vi "ControlProgram5.0.vi"() -> ()   [LabVIEW 2016]
uses:
  <vilib>/Utility/error.llb/DialogType.ctl
  <vilib>/Utility/miscctls.llb/LVPoint32TypeDef.ctl
  <vilib>/DAQmx/write.llb/DAQmx Write (Digital Bool 1Line 1Point).vi
  <vilib>/DAQmx/create/channels.llb/DAQmx Create Channel (DO-Digital Output).vi
  <vilib>/platform/TimedLoop/XDataNode/XDataNode.xnode
  <vilib>/Platform/TimedLoop/XDataNode/nitl_modes.ctl
  <vilib>/Platform/TimedLoop/XDataNode/XDNodeRunTimeDep.lvlib
  <vilib>/Platform/TimedLoop/XDataNode/wakeup.ctl
  <vilib>/Platform/TimedLoop/XDataNode/timing_clust.ctl
  <vilib>/DAQmx/create/channels.llb/DAQmx Create Channel (AI-Voltage-Basic).vi
  <vilib>/DAQmx/create/channels.llb/DAQmx Create Channel (AO-Voltage-Basic).vi
  <vilib>/DAQmx/write.llb/DAQmx Write (Analog 1D DBL NChan 1Samp).vi
  <resource>/objmgr/daqmx.rc
  <vilib>/Analysis/NI_AALBase.lvlib
  <vilib>/Analysis/baseanly.llb/Mean (DBL).vi
  <vilib>/Instr/_visa.llb/VISA Configure Serial Port (Instr).vi
  <vilib>/Utility/inputDevices.llb/mouseAcquire.vi
  <vilib>/Utility/inputDevices.llb/closeMouse.vi
  <vilib>/DAQmx/read.llb/DAQmx Read (Analog 2D DBL NChan NSamp).vi
  <vilib>/DAQmx/configure/timing.llb/DAQmx Timing (Sample Clock).vi
panel:
  out "Chart Freq (Hz)":dbl
  out "Waveform Chart 3":dbl[][](graph)
  out "Cal values":T1={"AX alpha"=672.9952101249002, "BX alpha"=822.8320399167465, "AX kappa"=0.3432739170419873, "BX kappa"=0.22087046979741862, "AX offset"=-0.002065833400375715, "BX offset"=0.010483360643544744, "AY alpha"=702.0654168010462, "BY alpha"=773.6701766674906, "AY kappa"=0.33643150106915, "BY kappa"=0.2444549177225145, "AY offset"=-0.1177594339643395, "BY offset"=0.06470506082263472}
  in  "Inject Pump 1":bool
  in  "Inject Pump 2":bool
  in  "Tab Control 2":T2(tab)
  in  "Force FB script":bool
  in  "Got ADig bead":bool
  in  "Move Cap. 2 (ADig Top)":bool
  in  "Dump beads":bool
  in  "Got DNA bead":bool
  in  "Delta after tether":dbl=3.1
  in  "TA Cancel Save?":bool
  in  "Min fish\ndelta (V)":dbl=2.8 min=0.0 max=10.0 step=0.1
  in  "Max fish\ndelta (V)":dbl=3.8 min=0.0 max=10.0 step=0.1
  in  "Fish Speed (ms)":i32=3000
  in  "Wait (ms)":i32=1500
  in  "# attempts":dbl=10.0
  in  "Cutoff force (pN)":dbl=5.0
  in  "Raster after\n tether?":bool=TRUE
  out "Tether":bool
  out "Attempt #":i32
  in  "Cal @ Delta (V)":dbl=5.0
  in  "Cal stage position":i32=3
  in  "Conv Y (nm/V)":dbl=505.0
  in  "Conv X (nm/V)":dbl=892.0
  out "Cal Final Sampling Rate":dbl
  in  "Cal Averaging":i32=1
  in  "Wait before dip (s)":dbl=3.0
  in  "Start dipping after?":bool
  in  "Start trap delta (V)":dbl=3.85
  in  "Cancel dwell":bool
  in  "Pause dwell":bool
  in  "Return position":dbl=3.0
  in  "Dip duration":dbl=15.0
  in  "Dip position":dbl=4.0
  in  "Dip":bool
  out "Dip time":i32
  out "error out":errorcluster
  in  "Stop":bool=TRUE
  in  "?":T3(tab)=enum."Mouse control"
  in  "Save N sets":bool
  in  "N sets":i32=200
  in  "Cal sets to save":i32=25
  in  "Reset data stream":bool
  out "Buffer Overflow":bool
  out "Stage moving":bool
  in  "Comment":string="wtUvrD 0.5 uM ATP"
  in  "Raster scan":bool
  out "Saving":bool
  in  "Save cal":bool
  in  "Save Data":bool
  in  "Stop saving":bool
  out "Calibrating":bool
  out "Progress":dbl(slide) scale=0.0..100.0
  in  "Read Cal":bool
  in  "Fish":bool
  in  "Averaging Number":i32=1250
  out "Final Sampling Rate":dbl=100.0
  in  "Trap position":cluster{"X":dbl, "Y":dbl}={"X"=1.6, "Y"=4.95}
  in  "Trap delta":dbl=5.1 min=0.0 max=10.0 step=0.1
  in  "Fixed X":dbl=1.6
  in  "Fixed Y":dbl=0.7
  in  "Shutter 1 (B)":bool
  in  "Shutter 2 (A)":bool
  in  "Pulling direction":bool=TRUE
  out "Raster scanning...":bool
  out "Current file name":path
  in  "AX alpha":dbl format="%#_3p"
  in  "BX alpha":dbl format="%#_3g"
  in  "AX kappa":dbl format="%#_3g"
  in  "BX kappa":dbl format="%#_3g"
  in  "AX offset":dbl format="%#_3g"
  in  "BX offset":dbl format="%#_3g"
  in  "AY alpha":dbl format="%#_3g"
  in  "BY alpha":dbl format="%#_3g"
  in  "AY kappa":dbl format="%#_3g"
  in  "BY kappa":dbl format="%#_3g"
  in  "AY offset":dbl format="%#_3g"
  in  "BY offset":dbl format="%#_3g"
  out "Buffer status":u8(slide) scale=0.0..100.0
  in  "dump spot":string="Dump beads spot"
  in  "up flow spot":string="Upper flow spot"
  in  "low flow spot":string="Lower flow spot"
  in  "up cap":string="Upper capillary (ADig beads)"
  in  "bottom cap":string="Lower capillary (DNA beads)"
  in  "Move to Position 5":bool
  in  "Set Position 5":bool
  in  "Saved stage positions":dbl[][](array[numeric])=[[1.0, 0.0, 0.0, 0.0], [2.0, 0.28481, -2.63158, -0.02256], [3.0, 1.27978, -0.73974, 0.0], [4.0, 1.27978, -2.1978, 0.0], [5.0, 0.03306, -2.63158, -0.02256]]
  in  "Set Position 2":bool
  in  "Move to Position 2":bool
  in  "Set Position 1":bool
  in  "Move to Position 1":bool
  in  "Set Position 4":bool
  in  "Move to Position 4":bool
  in  "Set Position 3":bool
  in  "Move to Position 3":bool
  out "Stage error":errorcluster
  in  "Normal \nVolume (ul) 2":dbl
  in  "Normal \nRate (ul/hr)":dbl
  in  "Normal \nVolume (ul)":dbl
  in  "Flush\nRate (ul/min)":dbl
  in  "Flush\nVolume (ul)":dbl
  in  "Flush \nRate (ul/min)  2":dbl
  in  "Flush Pump 2":bool
  in  "Flush\nVolume (ul)  2":dbl
  in  "Flush Pump 1":bool
  in  "Normal \nRate (ul/hr)  2":dbl
  in  "Write Wait":i32=1000
  in  "Use Mouse to Move Trap?":bool
  in  "Pause Mouse/Mirror Connection":bool
  out "Reference Voltage":cluster{dbl, dbl}={0.0, -0.0}
  out "Saved voltage":cluster{dbl, dbl}
  out "Real Coordinates":cluster{"Horizontal":i32, "Vertical":i32}={"Horizontal"=145, "Vertical"=-1746}
  out "CoordinatesMousePressed":T4
  out "Sum error":dbl(knob) scale=-0.2..0.2
  out "Trap sep":waveform(dbl)[](graph)
  in  "Set reading to\nsetpoint":bool
  in  "Offset Y (nm)":dbl format="%0.2f"
  in  "Offset X (nm)":dbl format="%0.2f"
  in  "Remove offsets":bool
  in  "Force Feedback":bool
  out "Feedback Output Voltage 2":cluster{dbl, dbl} {"?" format="%#_4g"; "?" format="%#_4g"}
  in  "Max value X":dbl=10.0 format="%.1f"
  in  "Min value X":dbl format="%0.1f"
  in  "Max value Y":dbl=10.0 format="%.1f"
  in  "Min value Y":dbl format="%.1g"
  in  "Offset":cluster{"Off Y":dbl, "Off X":dbl}={"Off Y"=1.5, "Off X"=0.17}
  in  "Setpoint voltage":cluster{"SP Y":dbl, "SP X":dbl}={"SP Y"=0.6, "SP X"=0.0}
  in  "Feedback const":T5={"Ki_B_Y"=0.5, "Ki_B_X"=0.0, "Kp Y"=1.0, "Kp X"=0.0}
  out "Mean Trap Pos X 2 (nm)":dbl format="%0.2f"
  out "Mean Trp Pos Y 2 (nm)":dbl format="%0.2f"
  out "T2 X RMS (A)":dbl format="%0.2f"
  out "T2 Y RMS (A)":dbl format="%0.2f"
  in  "# scans":i32=1
  in  "Speed (ms)":i32=10000
  in  "Min delta":dbl=3.2
  in  "Load param":bool
  in  "Max delta":dbl=4.1
  in  "Scan Parameters":T6(array[cluster])=[{"Label"="Offset", "Max delta 2"=3.8, "Min delta 2"=2.4, "Speed (ms) 2"=10000, "# scans 2"=1}]
  in  "Trap delta\nafter":dbl=3.6
  in  "Stop raster":bool
  out "Scan Range (nm)":dbl
  out "Scan Speed (nm/s)":dbl
  out "Continue to display?":bool
  out "Video Error":errorcluster
  in  "# Samples/channel (in)":i32=40000 format="%.2f"
  out "Buffer size\n(Samples/channel)":u32
  out "DAQ rate\n(Samples/s)":dbl format="%#_6p"
  out "# Samples/channel":i32=1250
  out "# Samples/channel/s":dbl
  out "AvailSampPerChan":u32
  out "Data update period (s/set)":dbl format="%#_6p"
  out "AvailSampPerChan 2":u32
  in  "PC samp per channel":i32=1000
  in  "Sampling Rate":dbl=125000.0 format="%0.0p"
  in  "DAQ Rate2":dbl=1000000.0 format="%#_6p"
  out "Data period (s)":dbl format="%#_6p"
  in  "Tether break\nforce (pN)":dbl=1.0
  in  "Path":path=path "D:/data"
  in  "Save file index":dbl
  out "Mirror task":refnum<k21>
  in  "HWP1":string="Half waveplate 1: differential trap power"
  in  "HWP0":string="Half waveplate 0: total trap power"
  in  "Move 1":bool
  in  "\"Degrees\" 1":dbl
  in  "Move 0":bool
  in  "\"Degrees\" 0":dbl
  out "Chamber":T7(plugin-control)
  out "Deflection":T4
  in  "Sampling Rate":dbl=125000.0 format="%0.2f"
  in  "Averaging Number":i32=12500
  in  "DAQ Rate":dbl=1000000.0
  out "Final Sampling Rate":dbl
  in  "Tab Control":T8(tab)
  in  "Downsamp\nfact":dbl=250.0
  out "Bead sep":waveform(dbl)[](graph)
  out "Force (pN)":waveform(dbl)[](graph)
  out "Mean force (pN)":dbl format="%0.2f"
  out "Force noise (pN)":dbl format="%0.2f"
  out "Mean Bead Sep\n(nm)":dbl format="%0.2f"
  out "Bead Sep Noise\n(A)":dbl format="%0.2f"
  out "PSD 2":cluster{dbl[], dbl[]}(graph)
  out "PSD 1":cluster{dbl[], dbl[]}(graph)
  out "PSD 1 Sum":dbl(slide) scale=0.0..10.0
  out "PSD 2 Sum":dbl(slide) scale=0.0..10.0
  in  "Start":bool
  out "All signals":waveform(dbl)[](graph)
  # "Bead Calibration"
  # "X"
  # "Y"
  # "Pump #1 Controls"
  # "Pump #2 Controls"
  # "Retract the pumps manually. Change it back to INFUSE when you're done. Suck it up, don't whine."
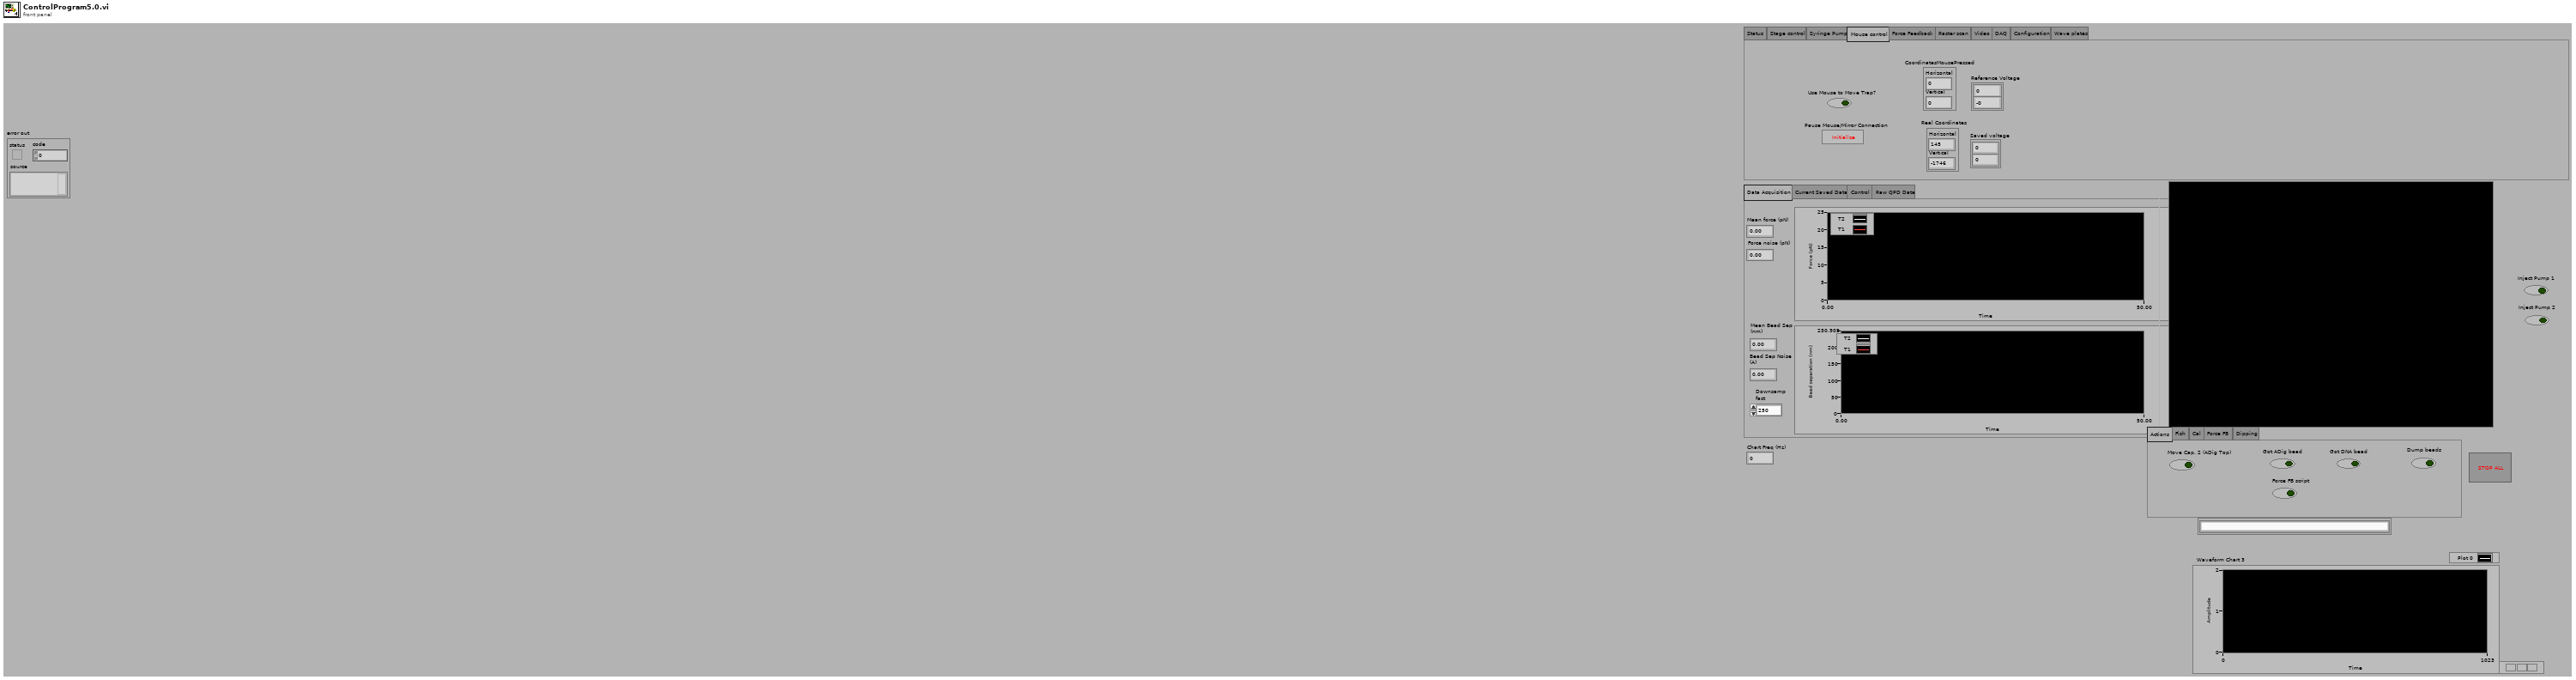
[diagram p1: front panel]
types:
  T1 = cluster{"AX alpha":dbl, "BX alpha":dbl, "AX kappa":dbl, "BX kappa":dbl, "AX offset":dbl, "BX offset":dbl, "AY alpha":dbl, "BY alpha":dbl, "AY kappa":dbl, "BY kappa":dbl, "AY offset":dbl, "BY offset":dbl}
  T2 = enum32{"Actions", "Fish", "Cal", "Force FB", "Dipping"}
  T3 = enum32{"Status", "Stage control", "Syringe Pump", "Mouse control", "Force Feedback", "Raster scan", "Video", "DAQ", "Configuration", "Wave plates"}
  T4 = typedef "LVPoint32TypeDef.ctl" = cluster{"Horizontal":i32, "Vertical":i32}
  T5 = cluster{"Ki_B_Y":dbl, "Ki_B_X":dbl, "Kp Y":dbl, "Kp X":dbl}
  T6 = cluster{"Label":string, "Max delta 2":dbl, "Min delta 2":dbl, "Speed (ms) 2":i32, "# scans 2":i32}[]
  T7 = typedef "IMAQ Image.ctl" = refnum<image>
  T8 = enum32{"Data Acquisition", "Current Saved Data", "Control", "Raw QPD Data"}
  T9 = enum16{"open", "replace", "create", "open or create", "replace or create", "replace or create with confirmation"}
  T10 = enum16{"big-endian, network order", "native, host order", "little-endian"}
  T11 = cluster{string, string, string, string, string, string, string, string}
  T12 = typedef "XDNodeRunTimeDep.lvlib/timing_clust.ctl" = cluster{"Expected End [f-1]":u64, "Actual End [f-1]":u64, "Finished Late? [f-1]":bool, "Expected End [i-1]":u64, "Actual End [i-1]":u64, "Finished Late? [i-1]":bool, "Expected Start [i]":u64, "Actual Start [i]":u64, "Expected Start [f]":u64, "Actual Start [f]":u64, "Source Name":string, "Structure Name":string, "Period":i64, "Deadline":i64, "Offset":i64, "Start":i64, "Priority":i32, "Timeout":i32, "Mode":T13, "Wakeup Reason":T14, "Error":errorcluster, "Source Type":string, "Secondary Source Type":string, "Global End Time":u64, "Global Start Time":u64, "Frame Duration":u64, "Iteration Duration":u64, "Assigned CPU":i32, "I/O Scan Engine Mode":u32}
  T13 = typedef "XDNodeRunTimeDep.lvlib/nitl_modes.ctl" = enum32{"No Change", "Process missed periods, maintain original phase", "Discard missed periods, maintain original phase", "Process missed periods, ignore original phase", "Discard missed periods, ignore original phase"}
  T14 = typedef "XDNodeRunTimeDep.lvlib/wakeup.ctl" = enum32{"Normal", "Aborted", "Asynchronous wakeup", "Timing source error", "Timed loop error", "Timeout"}
  T15 = typedef "DialogType.ctl" = u16
  T16 = cluster{"button 1":bool, "button 2":bool, "button 3":bool, "button 4":bool}
  T17 = cluster{"[0]":dbl, "[1]":dbl, "[2]":dbl, "[3]":dbl, "[4]":dbl, "[5]":dbl, "[6]":dbl, "[7]":dbl, "[8]":dbl, "[9]":dbl, "[10]":dbl, "[11]":dbl}
  T18 = cluster{"Label":string, "Max delta 2":dbl, "Min delta 2":dbl, "Speed (ms) 2":i32, "# scans 2":i32}
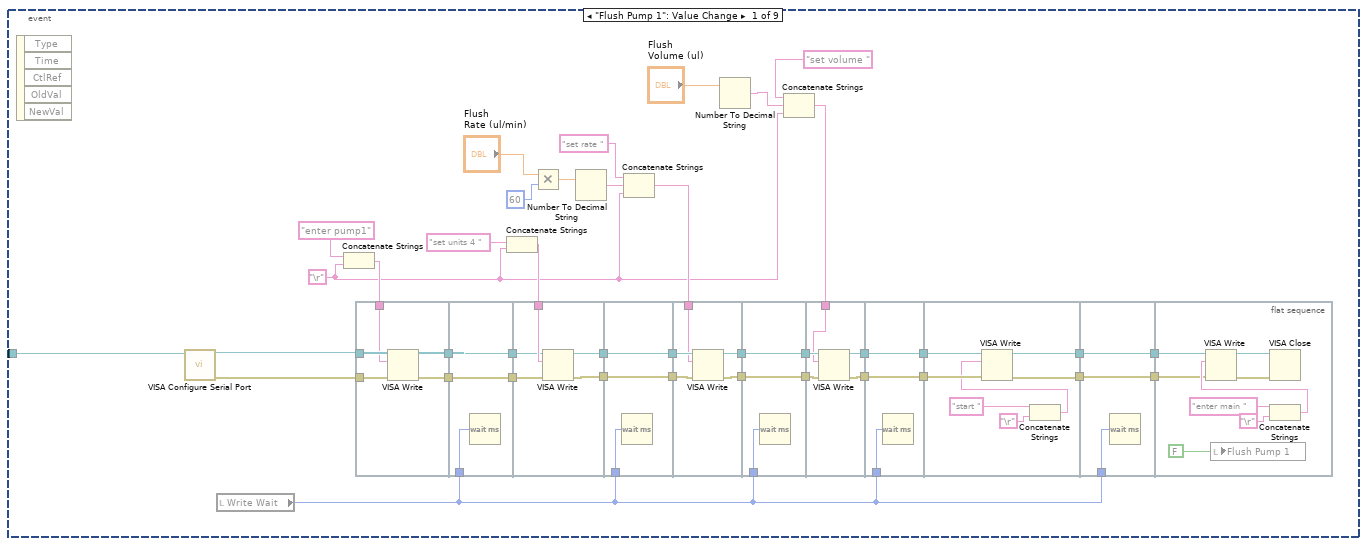
[diagram p2: hidden frame]
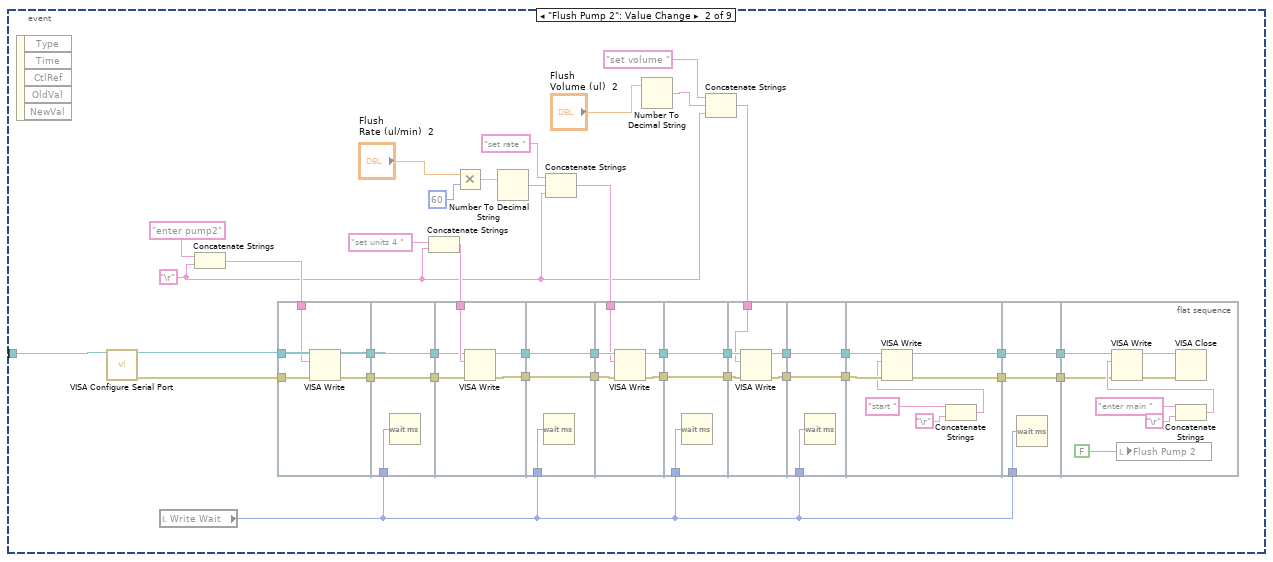
[diagram p3: hidden frame]
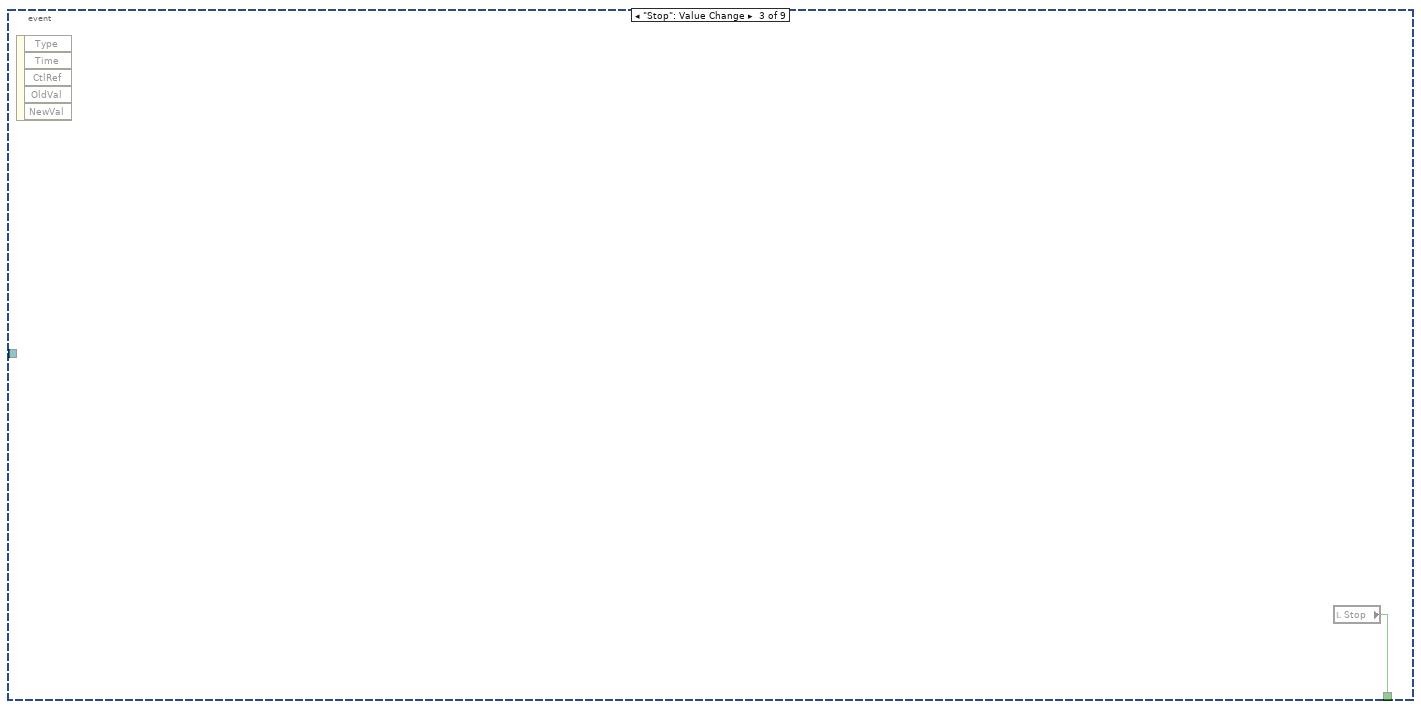
[diagram p4: hidden frame]
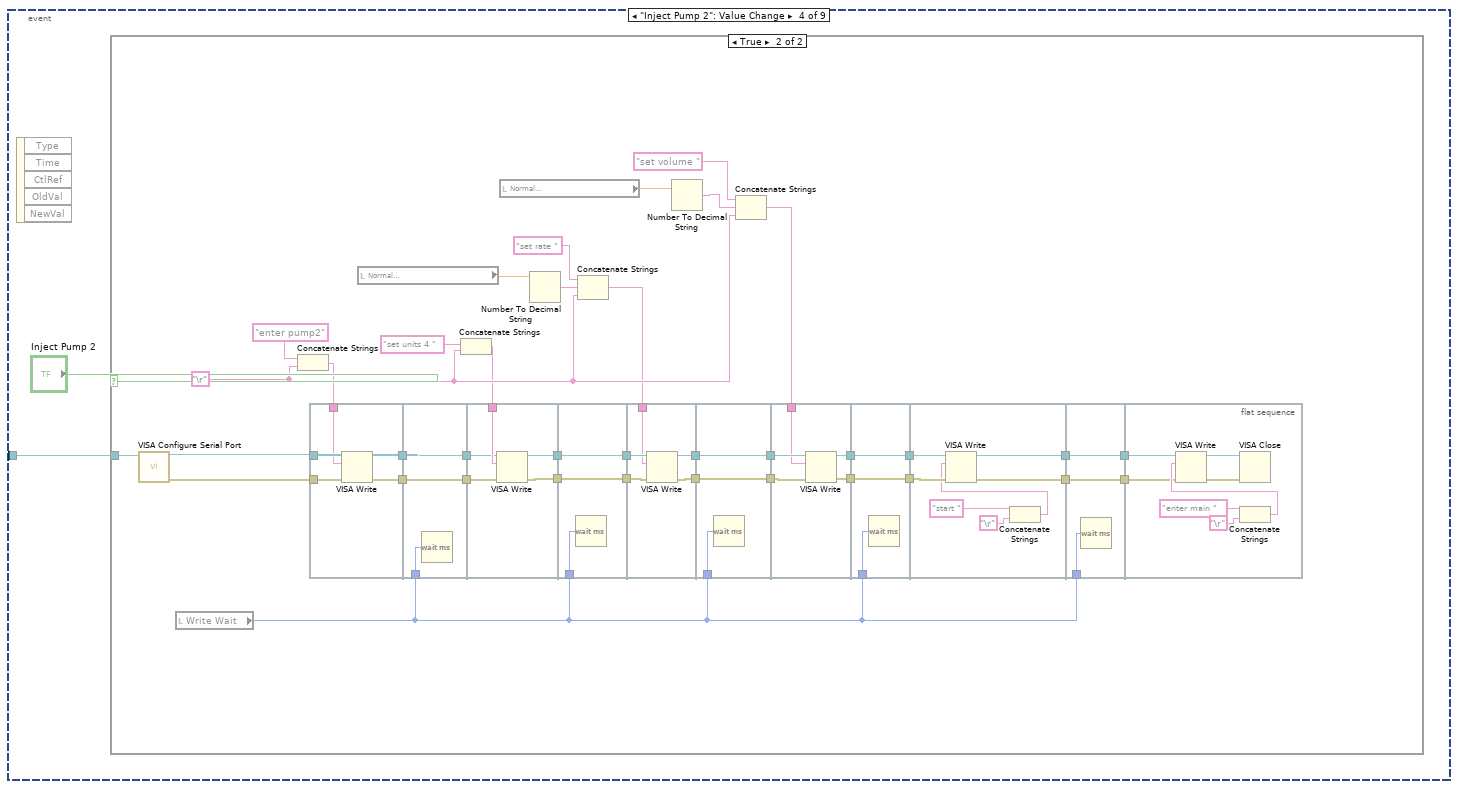
[diagram p5: hidden frame]
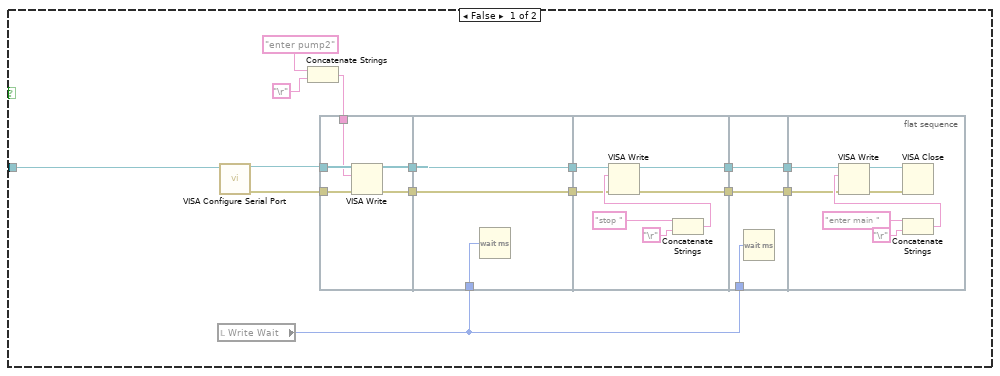
[diagram p6: hidden frame]
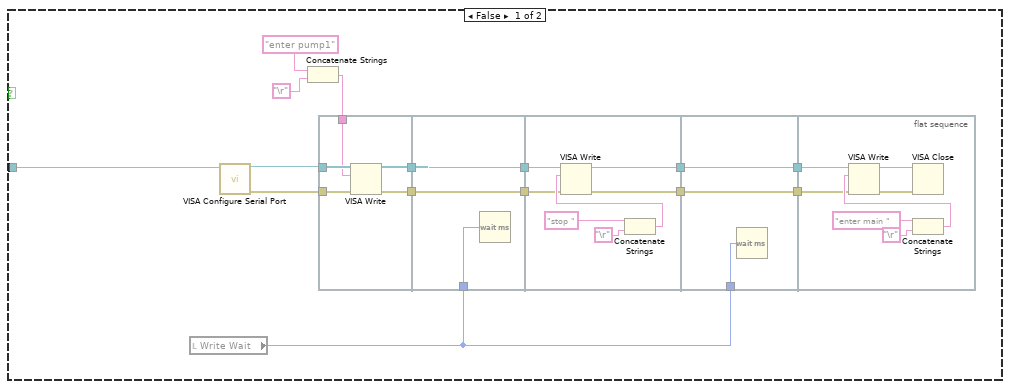
[diagram p7: hidden frame]
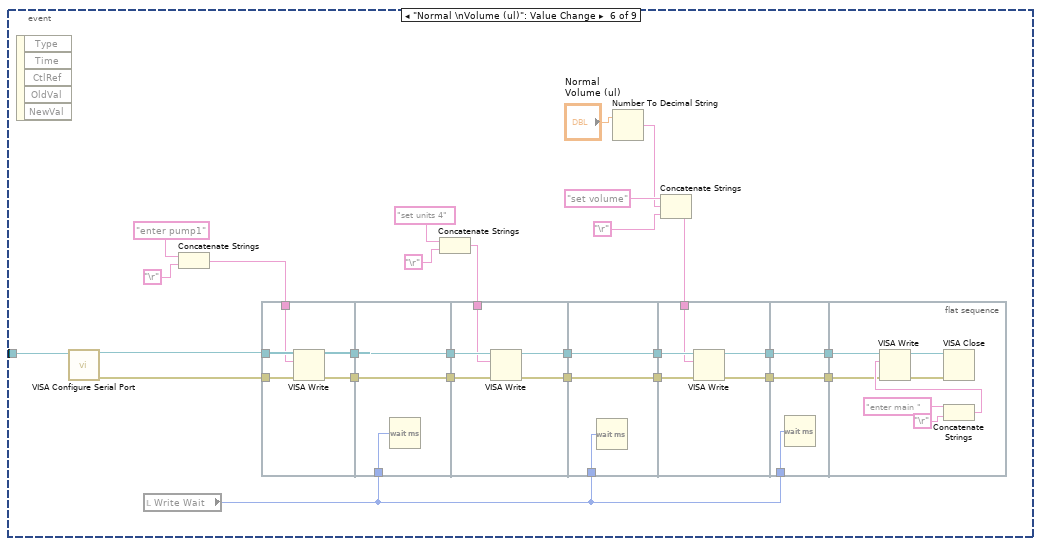
[diagram p8: hidden frame]
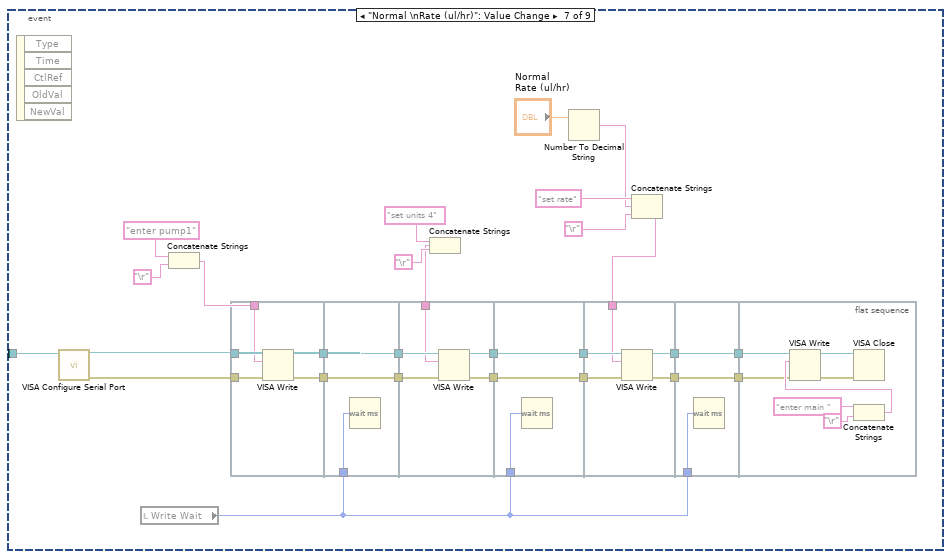
[diagram p9: hidden frame]
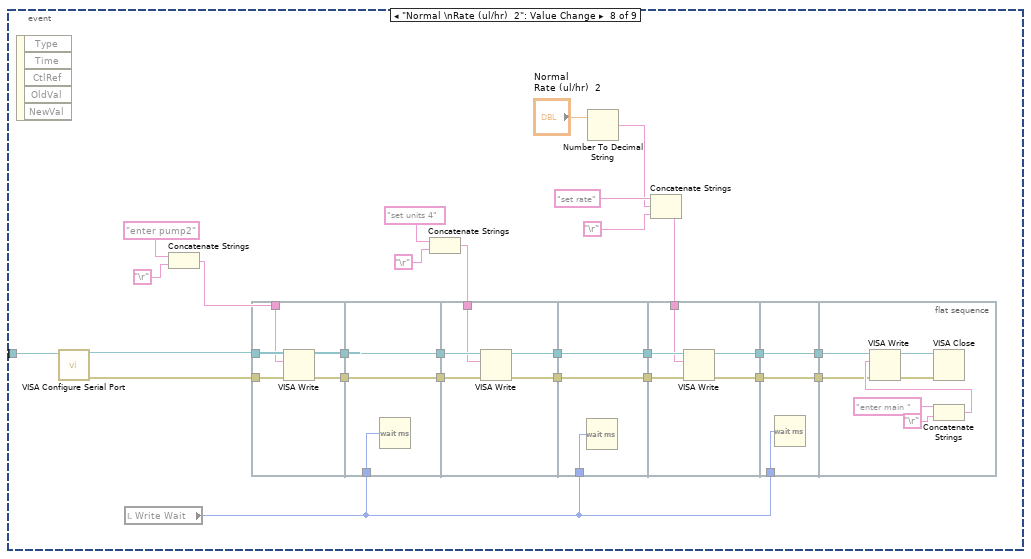
[diagram p10: hidden frame]
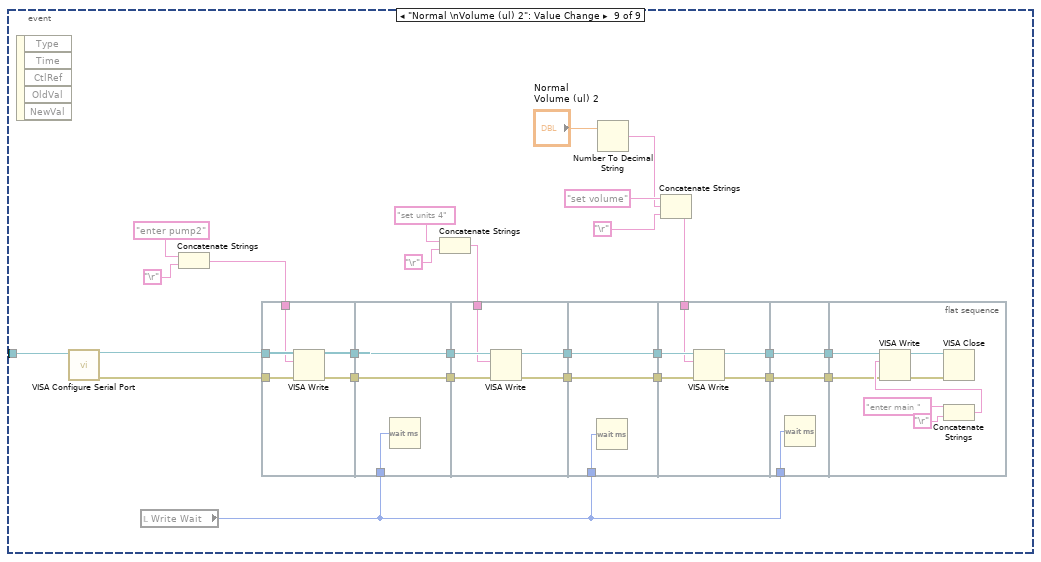
[diagram p11: hidden frame]
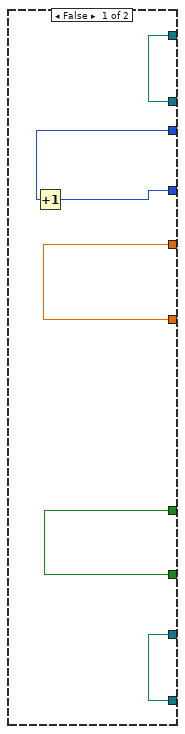
[diagram p18: hidden frame]
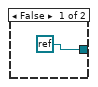
[diagram p19: hidden frame]
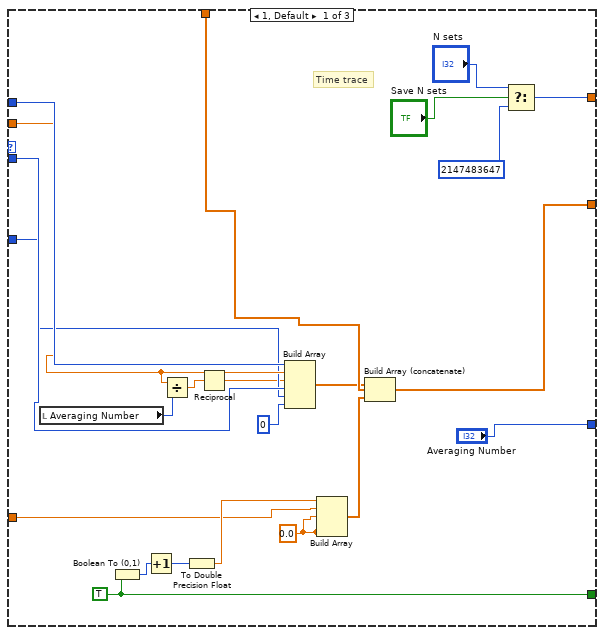
[diagram p20: hidden frame]
diagram:
  w43 = 10.0 ("Minimum Value")
  w44 = -10.0 ("Minimum Value")
  w46 = -2.0 ("Minimum Value")
  w47 = 2.0 ("Maximum Value")
  w72 = 10123 items=["Finite Samples"=10178, "Continuous Samples"=10123] ("sample mode")
  w93 = tag "Dev1/port2/line1"  # Shutter 2
  w96 = tag "Dev1/port1/line4"  # Shutter 1
  # "Create channels for movable mirror"
  # "Create channels for detectors"
  n1 = call-poly <vilib>:"DAQmx Create Virtual Channel.vi"("maximum value"=w47, "minimum value"=w46, "physical channels"=tag "Dev1/ai0" ("Physical Channel")) -> ("task out"=w48:refnum<k21>, "error out"=w71:errorcluster)  [unwired: 11 in]
  n2 = call-poly <vilib>:"DAQmx Create Virtual Channel.vi"("task in"=w48, "maximum value"=w47, "minimum value"=w46, "physical channels"=tag "Dev1/ai1", "error in"=w71) -> ("task out"=w69:refnum<k21>, "error out"=w68:errorcluster)  [unwired: 9 in]
  n3 = call-poly <vilib>:"DAQmx Create Virtual Channel.vi"("task in"=w69, "maximum value"=w47, "minimum value"=w46, "physical channels"=tag "Dev1/ai2", "error in"=w68) -> ("task out"=w60:refnum<k21>, "error out"=w59:errorcluster)  [unwired: 9 in]
  n4 = call-poly <vilib>:"DAQmx Create Virtual Channel.vi"("task in"=w60, "maximum value"=w47, "minimum value"=w46, "physical channels"=tag "Dev1/ai3" ("Physical Channel"), "error in"=w59) -> ("task out"=w45:refnum<k21>, "error out"=w65:errorcluster)  [unwired: 9 in]
  n5 = call-poly <vilib>:"DAQmx Create Virtual Channel.vi"("task in"=w45, "maximum value"=w43, "minimum value"=w44, "physical channels"=tag "Dev1/ai4", "error in"=w65) -> ("task out"=w63:refnum<k21>, "error out"=w62:errorcluster)  [unwired: 9 in]
  n6 = call-poly <vilib>:"DAQmx Create Virtual Channel.vi"("task in"=w63, "maximum value"=w43, "minimum value"=w44, "physical channels"=tag "Dev1/ai5", "error in"=w62) -> ("task out"=w58:refnum<k21>, "error out"=w57:errorcluster)  [unwired: 9 in]
  n7 = call-poly <vilib>:"DAQmx Create Virtual Channel.vi"("task in"=w58, "maximum value"=w43, "minimum value"=w44, "physical channels"=tag "Dev1/ai6", "error in"=w57) -> ("task out"=w52:refnum<k21>, "error out"=w50:errorcluster)  [unwired: 9 in]
  n8 = call-poly <vilib>:"DAQmx Create Virtual Channel.vi"("task in"=w52, "maximum value"=w43, "minimum value"=w44, "physical channels"=tag "Dev1/ai7", "error in"=w50) -> ("task out"=w51:refnum<k21>, "error out"=w49:errorcluster)  [unwired: 9 in]
  n9 = call-poly <vilib>:"DAQmx Timing.vi"("task/channels in"=w51, "sample mode"=w72, "samples per channel"="PC samp per channel", "rate"="Sampling Rate", "error in"=w49) -> ("task out"=w55:refnum<k21>, "error out"=w54:errorcluster)  [unwired: 9 in]
  n10 = call-poly <vilib>:"DAQmx Create Virtual Channel.vi"("maximum value"="Max value Y", "minimum value"="Min value Y", "physical channels"=tag "Dev1/ao1" ("Trap X Axis")) -> ("task out"=w39:refnum<k21>, "error out"=w41:errorcluster)  [unwired: 11 in]
  n11 = property class="DAQmx Timing"(reference=w55, error in=w54, "More:AI Convert:Rate"="DAQ Rate2") -> (reference out=w6:refnum<k21>, error out=w5:errorcluster, "SampClk.Rate"=→"DAQ rate\n(Samples/s)":dbl)
  n12 = call-poly <vilib>:"DAQmx Create Virtual Channel.vi"("task in"=w39, "maximum value"="Max value X", "minimum value"="Min value X", "physical channels"=tag "Dev1/ao0" ("Trap Y Axis"), "error in"=w41) -> ("task out"=w30:refnum<k21>, "error out"=w29:errorcluster)  [unwired: 9 in]
  "Mirror task" <- w30
  n13 = property class="DAQmx Buffer"(reference=w6, error in=w5) -> (reference out=w3:refnum<k21>, error out=w2:errorcluster, "Input.OnbrdBufSize"=→"Buffer size\n(Samples/channel)":u32)
  n14 = call <vilib>:"DAQmx Start Task.vi"("task/channels in"=w3, "error in"=w2) -> ("task out"=w31:refnum<k21>, "error out"=→"error out":errorcluster)  [unwired: 12 in]
  n15 = while {
    tunnel: [w412] -> w78
    tunnel: [w304] -> w79
    tunnel: [w420] -> w77
    tunnel: [w417] -> w74
    tunnel: w31 -> [w115]
    tunnel: w30 -> [w413]
    tunnel: w29 -> [w418]
    stop <- w417 stop-if-true
    w146 = "NI_ChannelName" ("name")
    w224 = -1
    # "Rewire everything"
    # "Invert these because changed\nfrom PSD to QPD"
    # "Trap Y"
    # "Trap X"
    # "Convert to\npN"
    # "Convert to\nnm"
    # "Subtract\noffset"
    # "Normalize by\nsum"
    # "B sum"
    # "BX"
    # "BY"
    # "AX"
    # "AY"
    # "A sum"
    # "Close files when done saving"
    n16 = property class="DAQmx Read"(reference=w115) -> (reference out=w114:refnum<k21>, "AvailSampPerChan"=→"AvailSampPerChan 2":u32)  [unwired: 1 in, 1 out]
    n17 = local read "Averaging Number"() -> (w110:i32)
    n18 = local read "Averaging Number"() -> (w116:i32)
    "# Samples/channel" <- w116
    n19 = local read "Sampling Rate"() -> (w416:dbl)
    n20 = call-poly <vilib>:"DAQmx Read.vi"("task/channels in"=w114, "number of samples per channel"=w110, "timeout"=10.0) -> ("task out"=w303:refnum<k21>, "data"=w111:dbl[][], "error out"=w227:errorcluster)  [unwired: 10 in]
    n21 = Unbundle By Name(w227) -> ("status"=w352:bool)
    n22 = Divide(x=w416, y="Cal Averaging") -> (x/y=→"Cal Final Sampling Rate":dbl)
    n23 = Divide(x=w416, y=w116) -> (x/y=→"Final Sampling Rate" →"# Samples/channel/s":dbl)
    n24 = case shown="True" w352 {
      frame False {
      }
      frame True {
        n25 = call <vilib>:"Beep.vi"() -> ()  [unwired: 12 in]
        "Buffer Overflow" <- TRUE
      }
    }
    n26 = local read "Buffer size\n(Samples/channel)"() -> (w299:u32)
    n27 = property class="DAQmx Read"(reference=w303) -> (reference out=w302:refnum<k21>, "AvailSampPerChan"=w300:u32)  [unwired: 1 in, 1 out]
    "AvailSampPerChan" <- w300
    n28 = local read "Cal values"() -> (w344:T1)
    n29 = Index Array(array=w111, index (row)=4) -> (element=w216:dbl[])  [unwired: 1 in]
    n30 = Index Array(array=w111, index (row)=0) -> (element=w226:dbl[])  [unwired: 1 in]
    n31 = Index Array(array=w111, index (row)=2) -> (element=w221:dbl[])  [unwired: 1 in]
    n32 = Index Array(array=w111, index (row)=1) -> (element=w225:dbl[])  [unwired: 1 in]
    n33 = Index Array(array=w111, index (row)=3) -> (element=w219:dbl[])  [unwired: 1 in]
    n34 = Index Array(array=w111, index (row)=6) -> (element=w218:dbl[])  [unwired: 1 in]
    n35 = Index Array(array=w111, index (row)=7) -> (element=w217:dbl[])  [unwired: 1 in]
    n36 = Index Array(array=w111, index (row)=5) -> (element=w215:dbl[])  [unwired: 1 in]
    n37 = Divide(x=w300, y=w299) -> (x/y=→"Buffer status":dbl)
    n38 = Unbundle(w344) -> ("AX alpha"=w332:dbl, "BX alpha"=w328:dbl, "AX kappa"=w324:dbl, "BX kappa"=w320:dbl, "AX offset"=w338:dbl, "BX offset"=w336:dbl, "AY alpha"=w335:dbl, "BY alpha"=w330:dbl, "AY kappa"=w326:dbl, "BY kappa"=w322:dbl, "AY offset"=w342:dbl, "BY offset"=w340:dbl)
    n39 = Multiply(x=w225, y=w224) -> (x*y=w220:dbl[])
    n40 = Multiply(x=w226, y=w224) -> (x*y=w222:dbl[])
    n41 = local write "AX alpha"(w332) -> ()
    n42 = local write "BY offset"(w340) -> ()
    n43 = Build Array(w222, w221, w220, w219, w218, w217, w216, w215) -> (w143:dbl[][])
    n44 = local write "BX alpha"(w328) -> ()
    n45 = case shown="True" "Reset data stream" {
      selector: "Reset data stream" -> [_ w449]
      tunnel: w302 -> [w441 w447]
      tunnel: [w441 w445] -> w304
      tunnel: w227 -> [w440 w444]
      tunnel: [w440 w442] -> _
      frame False {
      }
      frame True {
        n46 = Not(x=w449) -> (.not. x?=w448:bool)
        n47 = call <vilib>:"DAQmx Stop Task.vi"("task/channels in"=w447, "error in"=w444) -> ("task out"=w446:refnum<k21>, "error out"=w443:errorcluster)  [unwired: 12 in]
        n48 = local write "Reset data stream"(w448) -> ()
        n49 = local write "Buffer Overflow"(w448) -> ()
        n50 = call <vilib>:"DAQmx Start Task.vi"("task/channels in"=w446, "error in"=w443) -> ("task out"=w445:refnum<k21>, "error out"=w442:errorcluster)  [unwired: 12 in]
      }
    }
    n51 = call-poly <vilib>:"Mean.vi"("X"=w215) -> ("mean"=w358:dbl)  [unwired: 1 out]
    n52 = local write "AY offset"(w342) -> ()
    n53 = call-poly <vilib>:"Mean.vi"("X"=w216) -> ("mean"=w359:dbl)  [unwired: 1 out]
    n54 = call-poly <vilib>:"Mean.vi"("X"=w221) -> ("mean"=w365:dbl)  [unwired: 1 out]
    n55 = call-poly <vilib>:"Mean.vi"("X"=w219) -> ("mean"=w363:dbl)  [unwired: 1 out]
    n56 = call-poly <vilib>:"Mean.vi"("X"=w218) -> ("mean"=w362:dbl)  [unwired: 1 out]
    n57 = call-poly <vilib>:"Mean.vi"("X"=w217) -> ("mean"=w361:dbl)  [unwired: 1 out]
    n58 = local read "Averaging Number"() -> (w109:i32)
    n59 = local write "BY kappa"(w322) -> ()
    n60 = local write "AX kappa"(w324) -> ()
    n61 = call-poly <vilib>:"Mean.vi"("X"=w220) -> ("mean"=w364:dbl)  [unwired: 1 out]
    n62 = local write "AY kappa"(w326) -> ()
    n63 = call-poly <vilib>:"Mean.vi"("X"=w222) -> ("mean"=w366:dbl)  [unwired: 1 out]
    n64 = local read "DAQ rate\n(Samples/s)"() -> (w121:dbl)
    n65 = Build Array(w359, w358) -> (w357:dbl[])
    n66 = local write "BX kappa"(w320) -> ()
    n67 = local write "BY alpha"(w330) -> ()
    n68 = local write "AX offset"(w338) -> ()
    n69 = local write "BX offset"(w336) -> ()
    n70 = local write "AY alpha"(w335) -> ()
    n71 = Build Array(w366, w365, w364, w363, w362, w361) -> (w355:dbl[])
    n72 = Divide(x=w109, y=w121) -> (x/y=w118:dbl)
    "Data update period (s/set)" <- w118
    n73 = Reciprocal(x=w121) -> (1/x=w122:dbl)
    "Data period (s)" <- w122
    n74 = Divide(x=w366, y=w362) -> (x/y=w396:dbl)
    n75 = Divide(x=w365, y=w362) -> (x/y=w397:dbl)
    n76 = Divide(x=w364, y=w361) -> (x/y=w404:dbl)
    n77 = Divide(x=w363, y=w361) -> (x/y=w405:dbl)
    n78 = Subtract(x=w396, y="AY offset") -> (x-y=w378:dbl)
    n79 = Subtract(x=w397, y="AX offset") -> (x-y=w379:dbl)
    n80 = Subtract(x=w404, y="BY offset") -> (x-y=w377:dbl)
    n81 = Subtract(x=w405, y="BX offset") -> (x-y=w380:dbl)
    n82 = Subtract(x=w404, y=w396) -> (x-y=w394:dbl)
    n83 = Subtract(x=w405, y=w397) -> (x-y=w395:dbl)
    n84 = feedback #1(0.0) -> (w298:dbl)
    n85 = Multiply(x="Downsamp\nfact", y=w122) -> (x*y=w123:dbl)
    n86 = Multiply(x=w378, y="AY alpha") -> (x*y=w312:dbl)
    n87 = Multiply(x=w379, y="AX alpha") -> (x*y=w310:dbl)
    n88 = Multiply(x=w380, y="BX alpha") -> (x*y=w311:dbl)
    n89 = Multiply(x=w377, y="BY alpha") -> (x*y=w313:dbl)
    n90 = Add(x=w118, y=w298) -> (x+y=w296:dbl)
    n91 = feedback-in #1(w296) -> ()
    n92 = Square(x=w312) -> (x^2=w388:dbl)
    n93 = Square(x=w310) -> (x^2=w389:dbl)
    n94 = Square(x=w313) -> (x^2=w390:dbl)
    n95 = Square(x=w311) -> (x^2=w391:dbl)
    n96 = Bundle(w394, w395) -> (w112:cluster{dbl, dbl})  [unwired: 1 in]
    n97 = case shown="True" "Set reading to\nsetpoint" {
      tunnel: w112 -> [_ w438]
      frame False {
      }
      frame True {
        n98 = local write "Set reading to\nsetpoint"(FALSE ("Set reading to\nsetpoint")) -> ()
        n99 = local read "Trap position"() -> (w437:cluster{"X":dbl, "Y":dbl})
        n100 = property on="Setpoint voltage" class="Clust (strict)"("Val(Sgnl)"=w438) -> ()  [unwired: 2 in, 2 out]
        n101 = Unbundle(w437) -> ("X"=w436:dbl, "Y"=w435:dbl)
        n102 = Bundle("Y"=w435, "X"=w436) -> (w434:cluster{"Y":dbl, "X":dbl})  [unwired: 1 in]
        n103 = property on="Offset" class="Clust (strict)"("Val(Sgnl)"=w434) -> ()  [unwired: 2 in, 2 out]
      }
    }
    n104 = Reciprocal(x=w123) -> (1/x=→"Chart Freq (Hz)":dbl)
    n105 = To Time Stamp(1:w296) -> (0:w295:timestamp)
    n106 = Add(x=w388, y=w389) -> (x+y=w392:dbl)
    n107 = Add(x=w390, y=w391) -> (x+y=w403:dbl)
    n108 = Multiply(x=w310, y="AX kappa") -> (x*y=w306:dbl)
    n109 = Bundle("A y", "A x", "B y", "B x", "A sum", "B sum", "Trap x", "Trap y") -> (w286:T11)  [unwired: 1 in]
    n110 = Multiply(x=w311, y="BX kappa") -> (x*y=w307:dbl)
    n111 = Square Root(x=w392) -> (sqrt(x)=w408:dbl)
    n112 = Square Root(x=w403) -> (sqrt(x)=w407:dbl)
    n113 = Multiply(x=w312, y="AY kappa") -> (x*y=w308:dbl)
    n114 = Multiply(x=w313, y="BY kappa") -> (x*y=w309:dbl)
    n115 = Subtract(x=w358, y="Fixed Y") -> (x-y=w393:dbl)
    n116 = Subtract(x=w359, y="Fixed X") -> (x-y=w398:dbl)
    n117 = Cluster To Array(cluster=w286) -> (array=w285:string[])
    n118 = for {
      tunnel: w143 -> [w426] mode=indexing
      tunnel: w123 -> [w425]
      tunnel: "Downsamp\nfact" -> [w431]
      tunnel: [w429] -> w201 mode=indexing
      tunnel: w295 -> [w433]
      tunnel: w285 -> [w428] mode=indexing
      tunnel: "NI_ChannelName" ("name") -> [w427]
      n119 = call "Downsample 1D array.vi"("Ave N"=w431, "Arrray In"=w426) -> ("Array Out"=w432:dbl[])  [unwired: 9 in]
      n120 = Bundle By Name("Y"=w432, "dt"=w425, "t0"=w433) -> (w430:waveform(dbl))  [unwired: 1 in]
      n121 = Set Waveform Attribute(5:w428, 6:w427, 7:w430) -> (3:w429:waveform(dbl))  [unwired: 1 in, 2 out]
    }
    "All signals" <- w201
    n122 = Square(x=w308) -> (x^2=w381:dbl)
    n123 = Square(x=w306) -> (x^2=w382:dbl)
    n124 = Square(x=w309) -> (x^2=w383:dbl)
    n125 = Square(x=w307) -> (x^2=w384:dbl)
    n126 = Add(x=w381, y=w382) -> (x+y=w385:dbl)
    n127 = Add(x=w383, y=w384) -> (x+y=w386:dbl)
    n128 = Multiply(x=w393, y="Conv Y (nm/V)") -> (x*y=w315:dbl)
    n129 = Multiply(x=w398, y="Conv X (nm/V)") -> (x*y=w316:dbl)
    n130 = feedback #2() -> (w353:cluster{"B_Y":dbl, "B_X":dbl})  [unwired: 1 in]
    n131 = case shown="True" "Force Feedback" {
      tunnel: [w709 w725] -> w412
      tunnel: [w708 w724] -> w420
      tunnel: w112 -> [_ w723]
      tunnel: [cluster{"B_Y":dbl, "B_X":dbl} {"B_Y"=0.0, "B_X"=0.0} ("Sum error past") w715] -> w354
      tunnel: w353 -> [_ w722]
      tunnel: w413 -> [w709 w718]
      tunnel: w418 -> [w708 w717]
      frame False {
        # "Force feedback"
      }
      frame True {
        n132 = call "ForceFeedback2.vi"("PSD/Mirror Voltages"=w723, "Sum error"=w722, "task/channels in"=w718, "error in"=w717, "Desired voltage"="Setpoint voltage", "Feedback const"="Feedback const", "offset"="Offset") -> ("task out"=w725:refnum<k21>, "Sum error past"=w715:cluster{"B_Y":dbl, "B_X":dbl}, "Output Voltage"=→"Feedback Output Voltage 2":cluster{dbl, dbl}, "error out"=w724:errorcluster)  [unwired: 8 in, 1 out]
        n133 = local read "Pulling direction"() -> (w714:bool)
        n134 = Unbundle(w715) -> ("B_Y"=w712:dbl, "B_X"=w711:dbl)
        n135 = Select(t=w712, s=w714, f=w711) -> (s? t:f=→"Sum error":dbl)
      }
    }
    n136 = feedback-in #2(w354) -> ()
    n137 = Square Root(x=w385) -> (sqrt(x)=w314:dbl)
    n138 = Square Root(x=w386) -> (sqrt(x)=w409:dbl)
    n139 = Add(x=w314, y=w409) -> (x+y=w387:dbl)
    n140 = Build Array(w396, w397, w404, w405, w362, w361, w314, w409, w408, w407, w316, w315) -> ()  [unwired: 1 out]
    n141 = Divide(x=w387, y=2.0) -> (x/y=w351:dbl)
    n142 = Index Array(array=w201, index=6) -> (element=w148:waveform(dbl))
    n143 = Index Array(array=w201, index=7) -> (element=w150:waveform(dbl))
    n144 = local read "Fixed X"() -> (w205:dbl)
    n145 = local read "Fixed Y"() -> (w207:dbl)
    n146 = Unbundle By Name(w148) -> ("Y"=w209:dbl[])
    n147 = Unbundle By Name(w150) -> ("Y"=w208:dbl[])
    n148 = Index Array(array=w201, index=0) -> (element=w156:waveform(dbl))
    n149 = Index Array(array=w201, index=1) -> (element=w282:waveform(dbl))
    n150 = Index Array(array=w201, index=4) -> (element=w276:waveform(dbl))
    n151 = Subtract(x=w209, y=w205) -> (x-y=w206:dbl[])
    n152 = Subtract(x=w208, y=w207) -> (x-y=w203:dbl[])
    n153 = Unbundle By Name(w156) -> ("Y"=w274:dbl[])
    n154 = Unbundle By Name(w282) -> ("Y"=w273:dbl[])
    n155 = Unbundle By Name(w276) -> ("Y"=w272:dbl[])
    n156 = Index Array(array=w201, index=5) -> (element=w275:waveform(dbl))
    n157 = local read "Conv X (nm/V)"() -> (w204:dbl)
    n158 = local read "Conv Y (nm/V)"() -> (w202:dbl)
    n159 = Index Array(array=w201, index=2) -> (element=w153:waveform(dbl))
    n160 = Index Array(array=w201, index=3) -> (element=w279:waveform(dbl))
    n161 = Set Waveform Attribute(5:"T2 X", 6:w146, 7:w148) -> (3:w147:waveform(dbl))  [unwired: 1 in, 2 out]
    n162 = Set Waveform Attribute(5:"T2 Y", 6:w146, 7:w150) -> (3:w149:waveform(dbl))  [unwired: 1 in, 2 out]
    n163 = Unbundle By Name(w275) -> ("Y"=w269:dbl[])
    n164 = Unbundle By Name(w153) -> ("Y"=w271:dbl[])
    n165 = Unbundle By Name(w279) -> ("Y"=w270:dbl[])
    n166 = local read "Saving"() -> (w317:bool)
    n167 = local read "Tether"() -> (w318:bool)
    n168 = Divide(x=w274, y=w272) -> (x/y=w172:dbl[])
    n169 = Divide(x=w273, y=w272) -> (x/y=w170:dbl[])
    n170 = local read "AY offset"() -> (w260:dbl)
    n171 = local read "AX offset"() -> (w258:dbl)
    n172 = Multiply(x=w206, y=w204) -> (x*y=w140:dbl[])
    n173 = Multiply(x=w203, y=w202) -> (x*y=w142:dbl[])
    n174 = Less?(x=w351, y="Tether break\nforce (pN)") -> (x < y?=w349:bool)
    n175 = Divide(x=w270, y=w269) -> (x/y=w171:dbl[])
    n176 = Subtract(x=w170, y=w258) -> (x-y=w261:dbl[])
    n177 = local read "BY offset"() -> (w265:dbl)
    n178 = local read "BX offset"() -> (w268:dbl)
    n179 = Subtract(x=w172, y=w260) -> (x-y=w262:dbl[])
    n180 = Divide(x=w271, y=w269) -> (x/y=w173:dbl[])
    n181 = local read "AY alpha"() -> (w259:dbl)
    n182 = local read "AX alpha"() -> (w257:dbl)
    n183 = Compound Arithmetic op=AND(w317, w318, w349) -> (w348:bool)
    n184 = call-poly <vilib>:"Mean.vi"("X"=w142) -> ("mean"=w183:dbl)  [unwired: 1 out]
    "Mean Trp Pos Y 2 (nm)" <- w183
    n185 = Subtract(x=w173, y=w172) -> (x-y=w169:dbl[])
    n186 = Subtract(x=w171, y=w170) -> (x-y=w168:dbl[])
    n187 = Subtract(x=w140, y="Offset X (nm)") -> (x-y=w139:dbl[])
    n188 = Subtract(x=w142, y="Offset Y (nm)") -> (x-y=w141:dbl[])
    n189 = Subtract(x=w173, y=w265) -> (x-y=w267:dbl[])
    n190 = Subtract(x=w171, y=w268) -> (x-y=w266:dbl[])
    n191 = Subtract(x=w183, y=w142) -> (x-y=w182:dbl[])
    n192 = call-poly <vilib>:"Mean.vi"("X"=w140) -> ("mean"=w187:dbl)  [unwired: 1 out]
    "Mean Trap Pos X 2 (nm)" <- w187
    n193 = Build Array(w169, w168) -> (w166:dbl[][])
    n194 = Index Array(array=w166, index (row)=0) -> (element=w164:dbl[])  [unwired: 1 in]
    n195 = Index Array(array=w166, index (row)=1) -> (element=w163:dbl[])  [unwired: 1 in]
    n196 = call-poly <vilib>:"Mean.vi"("X"=w164) -> ("mean"=w162:dbl)  [unwired: 1 out]
    n197 = call-poly <vilib>:"Mean.vi"("X"=w163) -> ("mean"=w161:dbl)  [unwired: 1 out]
    n198 = Bundle("mean"=w162, "mean"=w161) -> ()  [unwired: 1 in, 1 out]
    n199 = local read "BY alpha"() -> (w264:dbl)
    n200 = local read "BX alpha"() -> (w263:dbl)
    n201 = Multiply(x=w262, y=w259) -> (x*y=w250:dbl[])
    n202 = Multiply(x=w261, y=w257) -> (x*y=w249:dbl[])
    n203 = Square(x=w182) -> (x^2=w181:dbl[])
    n204 = Subtract(x=w187, y=w140) -> (x-y=w186:dbl[])
    n205 = Bundle By Name(cluster=w149, "Y"=w141) -> (w199:waveform(dbl))
    n206 = case shown="True" w348 {
      selector: w348 -> [_ w452]
      frame False {
      }
      frame True {
        n207 = call <vilib>:"Beep.vi"() -> ()  [unwired: 12 in]
        n208 = Not(x=w452) -> (.not. x?=w450:bool)
        n209 = local write "Tether"(w450) -> ()
        n210 = local write "Force Feedback"(w450) -> ()
        n211 = property on="Stop saving" class="Bool (strict)"("Val(Sgnl)"="TA Cancel Save?") -> ()  [unwired: 2 in, 2 out]
      }
    }
    n212 = Bundle By Name(cluster=w147, "Y"=w139) -> (w200:waveform(dbl))
    n213 = Square(x=w186) -> (x^2=w185:dbl[])
    n214 = call-poly <vilib>:"Mean.vi"("X"=w181) -> ("mean"=w180:dbl)  [unwired: 1 out]
    n215 = Square(x=w250) -> (x^2=w256:dbl[])
    n216 = Multiply(x=w267, y=w264) -> (x*y=w248:dbl[])
    n217 = Square(x=w249) -> (x^2=w255:dbl[])
    n218 = Multiply(x=w266, y=w263) -> (x*y=w247:dbl[])
    n219 = call-poly <vilib>:"Mean.vi"("X"=w185) -> ("mean"=w184:dbl)  [unwired: 1 out]
    n220 = Build Array(w200, w199) -> (→"Trap sep":waveform(dbl)[])
    n221 = Square Root(x=w180) -> (sqrt(x)=w179:dbl)
    n222 = Square(x=w248) -> (x^2=w254:dbl[])
    n223 = Square(x=w247) -> (x^2=w253:dbl[])
    n224 = Add(x=w256, y=w255) -> (x+y=w252:dbl[])
    n225 = Square Root(x=w184) -> (sqrt(x)=w177:dbl)
    n226 = Multiply(x=w179, y=10) -> (x*y=→"T2 Y RMS (A)":dbl)
    n227 = Square Root(x=w252) -> (sqrt(x)=w135:dbl[])
    n228 = Add(x=w254, y=w253) -> (x+y=w251:dbl[])
    n229 = Set Waveform Attribute(5:"T2", 6:"NI_ChannelName" ("name"), 7:w156) -> (3:w155:waveform(dbl))  [unwired: 1 in, 2 out]
    n230 = Set Waveform Attribute(5:"T1", 6:"NI_ChannelName" ("name"), 7:w153) -> (3:w152:waveform(dbl))  [unwired: 1 in, 2 out]
    n231 = Square Root(x=w251) -> (sqrt(x)=w134:dbl[])
    n232 = Multiply(x=w177, y=10) -> (x*y=→"T2 X RMS (A)":dbl)
    n233 = Bundle By Name(cluster=w155, "Y"=w135) -> (w159:waveform(dbl))
    n234 = Bundle By Name(cluster=w152, "Y"=w134) -> (w229:waveform(dbl))
    n235 = Add(x=w135, y=w134) -> (x+y=w133:dbl[])
    n236 = case shown="True" "Remove offsets" {
      selector: "Remove offsets" -> [_ w423]
      frame False {
      }
      frame True {
        n237 = local read "Mean Trp Pos Y 2 (nm)"() -> (w421:dbl)
        n238 = Not(x=w423) -> (.not. x?=w424:bool)
        n239 = local read "Mean Trap Pos X 2 (nm)"() -> (w422:dbl)
        n240 = local write "Remove offsets"(w424) -> ()
        n241 = local write "Offset Y (nm)"(w421) -> ()
        n242 = local write "Offset X (nm)"(w422) -> ()
      }
    }
    n243 = Build Array(w159, w229) -> (→"Bead sep":waveform(dbl)[])
    n244 = local read "AY kappa"() -> (w246:dbl)
    n245 = local read "AX kappa"() -> (w245:dbl)
    n246 = Divide(x=w133, y=2) -> (x/y=w131:dbl[])
    n247 = local read "BX kappa"() -> (w243:dbl)
    n248 = local read "BY kappa"() -> (w244:dbl)
    n249 = call-poly <vilib>:"Mean.vi"("X"=w131) -> ("mean"=w130:dbl)  [unwired: 1 out]
    "Mean Bead Sep\n(nm)" <- w130
    n250 = local read "Calibrating"() -> (w410:bool)
    n251 = Multiply(x=w250, y=w246) -> (x*y=w239:dbl[])
    n252 = Multiply(x=w249, y=w245) -> (x*y=w240:dbl[])
    n253 = Square(x=w239) -> (x^2=w238:dbl[])
    n254 = Square(x=w240) -> (x^2=w237:dbl[])
    n255 = Subtract(x=w131, y=w130) -> (x-y=w129:dbl[])
    n256 = Multiply(x=w248, y=w244) -> (x*y=w241:dbl[])
    n257 = Multiply(x=w247, y=w243) -> (x*y=w242:dbl[])
    n258 = Add(x=w238, y=w237) -> (x+y=w234:dbl[])
    n259 = Square(x=w129) -> (x^2=w128:dbl[])
    n260 = Square Root(x=w234) -> (sqrt(x)=w197:dbl[])
    n261 = Square(x=w241) -> (x^2=w236:dbl[])
    n262 = Square(x=w242) -> (x^2=w235:dbl[])
    n263 = call-poly <vilib>:"Mean.vi"("X"=w128) -> ("mean"=w127:dbl)  [unwired: 1 out]
    n264 = Add(x=w236, y=w235) -> (x+y=w233:dbl[])
    n265 = Bundle By Name(cluster=w155, "Y"=w197) -> (w232:waveform(dbl))
    n266 = local read "Saving"() -> (w347:bool)
    n267 = Or(x=w410, y=w347) -> ()  [unwired: 1 out]
    n268 = Square Root(x=w127) -> (sqrt(x)=w126:dbl)
    n269 = local read "Raster scan"() -> (w160:bool)
    n270 = Square Root(x=w233) -> (sqrt(x)=w196:dbl[])
    n271 = Multiply(x=10, y=w126) -> (x*y=→"Bead Sep Noise\n(A)":dbl)
    n272 = Bundle By Name(cluster=w152, "Y"=w196) -> (w231:waveform(dbl))
    n273 = Add(x=w197, y=w196) -> (x+y=w195:dbl[])
    n274 = Build Array(w232, w231) -> (→"Force (pN)":waveform(dbl)[])
    n275 = flat-sequence {
      tunnel: w410 -> [w490]
      tunnel: w347 -> [_]
      tunnel: w410 -> [_]
      tunnel: w347 -> [_]
      tunnel: w143 -> [w474]
      tunnel: [w474] -> w368
      tunnel: w227 -> [w473]
      tunnel: [w473] -> w367
      tunnel: w355 -> [w472]
      tunnel: [w472] -> w360
      tunnel: w357 -> [w471]
      tunnel: [w471] -> w356
      tunnel: [w468] -> w346
      tunnel: [w465] -> w345
      tunnel: [w462] -> w214
      tunnel: [w461] -> w213
      tunnel: [w458] -> w212
      tunnel: w160 -> [w454]
      tunnel: w368 -> [w640]
      tunnel: w367 -> [w639]
      tunnel: w360 -> [_]
      tunnel: w356 -> [_]
      tunnel: w346 -> [w638]
      tunnel: w345 -> [w637]
      tunnel: w214 -> [w636]
      tunnel: w213 -> [w635]
      tunnel: w212 -> [w634]
      frame #0 {
        w485 = 0.0
        # "1: old trap\n0: fleezers"
        # "Create files if saving data"
        n276 = local read "Save N sets"() -> (w457:bool)
        n277 = local read "Sampling Rate"() -> (w488:dbl)
        n278 = Or(x=w457, y="Save Data") -> (x .or. y?=w455:bool)
        n279 = Build Array(w455, "Save cal", w454) -> (w476:bool[])
        n280 = Compound Arithmetic op=OR("Save Data", "Save cal", w454) -> (w478:bool)
        n281 = Boolean Array To Number(Boolean array=w476) -> (number=w475:u32)
        n282 = local read "Trap position"() -> (w484:cluster{"X":dbl, "Y":dbl})
        n283 = Unbundle(w484) -> ("X"=w482:dbl, "Y"=w483:dbl)
        n284 = Build Array(w485, w485, w483, w482, w485, w485) -> (w481:dbl[])
        n285 = feedback #3(refnum<k0> refnum) -> (w466:refnum<file>)
        n286 = feedback #4() -> (w463:dbl)  [unwired: 1 in]
        n287 = feedback #5(FALSE) -> (w459:bool)
        n288 = feedback #6(0) -> (w479:i32)
        n289 = feedback #7(refnum<k0> refnum) -> (w469:refnum<file>)
        n290 = case shown="True" w478 {
          tunnel: w490 -> [_ _]
          tunnel: 9 -> [_ w532]
          tunnel: w488 -> [_ w531]
          tunnel: 6 -> [_ w530]
          tunnel: 5 -> [_ w529]
          tunnel: w481 -> [_ w528]
          tunnel: [w495 1] -> w462
          tunnel: w479 -> [w496 _]
          tunnel: w475 -> [_ w503]
          tunnel: [w494 w501] -> w468
          tunnel: w469 -> [w494 _]
          tunnel: [w493 w500] -> w465
          tunnel: w466 -> [w493 _]
          tunnel: 1.0 -> [_ w499]
          tunnel: [w492 w498] -> w461
          tunnel: w463 -> [w492 _]
          tunnel: [w491 w497] -> w458
          tunnel: w459 -> [w491 _]
          frame False {
            n291 = Increment(x=w496) -> (x+1=w495:i32)
          }
          frame True {
            w504 = FALSE ("Save Data")
            w510 = FALSE
            w511 = T10."big-endian, network order" ("byte order (0:big-endian, network order)")
            n292 = local write "Save cal"(w504) -> ()
            n293 = local write "Save Data"(w504) -> ()
            n294 = case shown="4" w503 {
              tunnel: w532 -> [w578 w596 w632]
              tunnel: w531 -> [w577 w595 w631]
              tunnel: w530 -> [w576 w593 w627]
              tunnel: w529 -> [w575 w592 w626]
              tunnel: w528 -> [w573 w589 w623]
              tunnel: [w572 w588 w609] -> w525
              tunnel: [w574 w585 w608] -> w497
              tunnel: ["Averaging Number" 200 w606] -> _
              tunnel: w499 -> [w560 w580 w605]
              tunnel: [w556 "Cal sets to save" w598] -> w498
              frame 1, Default {
                w574 = TRUE
                w561 = 0.0
                # "Time trace"
                n295 = local read "Averaging Number"() -> (w571:i32)
                n296 = Boolean To (0,1)(Boolean=w574) -> (0, 1=w566:i16)
                n297 = Increment(x=w566) -> (x+1=w565:i16)
                n298 = Divide(x=w577, y=w571) -> (x/y=w570:dbl)
                n299 = To Double Precision Float(number=w565) -> (double precision float=w564:dbl)
                n300 = Reciprocal(x=w570) -> (1/x=w569:dbl)
                n301 = Build Array(w578, w577, w569, w576, w575, 0 ("f")) -> (w568:dbl[])
                n302 = Build Array(w564, w560, w561, w561, w561) -> (w567:dbl[])
                n303 = Build Array (concatenate)(w568, w573, w567) -> (w572:dbl[])
                n304 = Select(t="N sets", s="Save N sets", f=2147483647) -> (s? t:f=w556:i32)
              }
              frame 2 {
                w585 = FALSE
                w583 = 0.0
                # "Calibration file"
                n305 = Reciprocal(x=w595) -> (1/x=w594:dbl)
                n306 = Boolean To (0,1)(Boolean=w585) -> (0, 1=w587:i16)
                n307 = To Double Precision Float(number=w587) -> (double precision float=w586:dbl)
                n308 = Build Array(w596, w594, w594, w593, w592, 1) -> (w590:dbl[])
                n309 = Build Array(w586, w580, w583, w583, w583) -> (w584:dbl[])
                n310 = Build Array (concatenate)(w590, w589, w584) -> (w588:dbl[])
                "Calibrating" <- TRUE ("Calibrating")
              }
              frame 4 {
                w607 = 0
                w619 = 0.0
                w608 = TRUE
                # "Not using nsteps yet"
                # "FX curve"
                n311 = local read "Averaging Number"() -> (w630:i32)
                n312 = Boolean To (0,1)(Boolean=w608) -> (0, 1=w622:i16)
                n313 = Increment(x=w622) -> (x+1=w621:i16)
                n314 = To Double Precision Float(number=w621) -> (double precision float=w620:dbl)
                n315 = local write "Raster scan"(FALSE ("Raster scan")) -> ()
                n316 = Divide(x=w631, y=w630) -> (x/y=w629:dbl)
                n317 = Reciprocal(x=w629) -> (1/x=w628:dbl)
                n318 = Build Array(w620, w605, w619, w619, w619) -> (w618:dbl[])
                n319 = Build Array(w632, w631, w628, w627, w626, 2) -> (w624:dbl[])
                n320 = local read "Data update period (s/set)"() -> (w601:dbl)
                n321 = local read "Pulling direction"() -> (w616:bool)
                n322 = local read "Max delta"() -> (w614:dbl)
                n323 = local read "Min delta"() -> (w613:dbl)
                n324 = local read "# scans"() -> (w611:i32)
                n325 = local read "Speed (ms)"() -> (w602:i32)
                n326 = Subtract(x=w614, y=w613) -> (x-y=w612:dbl)
                n327 = Not(x=w616) -> (.not. x?=w615:bool)
                n328 = local read "Averaging Number"() -> (w606:i32)
                n329 = Boolean To (0,1)(Boolean=w615) -> (0, 1=w617:i16)
                n330 = Multiply(x=750.0, y=w601) -> (x*y=w599:dbl)
                n331 = Build Array(w617, w612, w607, w607, w611) -> (w610:dbl[])
                n332 = Divide(x=w602, y=w599) -> (x/y=w597:dbl)
                n333 = Build Array (concatenate)(w624, w623, w618, w610) -> (w609:dbl[])
                n334 = Round Toward +Infinity(x=w597) -> (ceil(x): smallest int >= x=w598:dbl)
                "Raster scanning..." <- TRUE ("Raster scanning...")
              }
            }
            n335 = call "CreateSaveFile.vi"("Index In"="Save file index", "Ext"=".dat", "Insert"="", "Directory"="Path") -> ("Path Out"=w509:path)  [unwired: 6 in, 1 out]
            "Current file name" <- w509
            n336 = Open/Create/Replace File(file path (use dialog)=w509, operation (0:open)=T9."create", access (0:read/write)=enum16{"read/write", "read-only", "write-only"}."write-only") -> (refnum out=w518:refnum<file>, error out=w519:errorcluster)  [unwired: 3 in, 1 out]
            n337 = Array Size(array=w525) -> (size(s)=w527:i32)
            n338 = case shown="True" w497 {
              tunnel: w509 -> [_ w555]
              tunnel: [refnum<k0> refnum w534] -> w500
              frame False {
              }
              frame True {
                w541 = 0.0
                n339 = Path To String(path=w555) -> (string=w551:string)
                n340 = Build Array(w541, w541, w541, w541, w541, w541, w541, w541) -> (w538:dbl[])
                n341 = String Length(string=w551) -> (length=w554:i32)
                n342 = Array Size(array=w538) -> (size(s)=w540:i32)
                n343 = Subtract(x=w554, y=4) -> (x-y=w552:i32)
                n344 = To Double Precision Float(number=w540) -> (double precision float=w539:dbl)
                n345 = String Subset(string=w551, length (rest)=w552) -> (substring=w550:string)  [unwired: 1 in]
                n346 = Build Array (concatenate)(w539, w538) -> (w537:dbl[])
                n347 = Concatenate Strings(w550, "_pos.dat" ("string")) -> (w548:string)
                n348 = String To Path(string=w548) -> (path=w547:path)
                n349 = Open/Create/Replace File(file path (use dialog)=w547, operation (0:open)=T9."create", access (0:read/write)=enum16{"read/write", "read-only", "write-only"}."write-only") -> (refnum out=w543:refnum<file>, error out=w544:errorcluster)  [unwired: 3 in, 1 out]
                n350 = Deny Access(4:w544, 7:w543) -> (3:w542:refnum<file>)  [unwired: 1 in, 1 out]
                n351 = Write to Binary File(file (use dialog)=w542, data=w537, 5:FALSE ("prepend array or string size? (T)"), 9:T10."big-endian, network order" ("byte order (0:big-endian, network order)")) -> (refnum out=w534:refnum<file>)  [unwired: 2 in, 2 out]
              }
            }
            n352 = Deny Access(4:w519, 7:w518) -> (0:w508:errorcluster, 3:w517:refnum<file>)  [unwired: 1 in]
            n353 = String Length(string="Comment") -> (length=w524:i32)
            n354 = To Double Precision Float(number=w527) -> (double precision float=w526:dbl)
            n355 = To Double Precision Float(number=w524) -> (double precision float=w523:dbl)
            n356 = Build Array (concatenate)(w526, w525, w523) -> (w514:dbl[])
            n357 = Write to Binary File(file (use dialog)=w517, data=w514, error in=w508, 5:w510, 9:w511) -> (refnum out=w513:refnum<file>, error out=w507:errorcluster)  [unwired: 1 in, 1 out]
            n358 = Write to Binary File(file (use dialog)=w513, data="Comment", error in=w507, 5:w510, 9:w511) -> (refnum out=w501:refnum<file>)  [unwired: 1 in, 2 out]
            "Saving" <- TRUE
          }
        }
        n359 = feedback-in #3(w465) -> ()
        n360 = feedback-in #4(w461) -> ()
        n361 = feedback-in #5(w458) -> ()
        n362 = feedback-in #6(w462) -> ()
        n363 = feedback-in #7(w468) -> ()
      }
      frame #1 {
        n364 = local read "Saving"() -> (w633:bool)
        n365 = case shown="True" w633 {
          tunnel: w640 -> [_ w657]
          tunnel: w639 -> [_ w656]
          tunnel: w638 -> [_ w655]
          tunnel: w637 -> [_ w654]
          tunnel: w636 -> [_ w644]
          tunnel: w635 -> [_ w645]
          tunnel: w634 -> [_ w648]
          frame False {
            (unwired) FALSE ("Calibrating")
          }
          frame True {
            n366 = local read "Stop"() -> (w652:bool)
            n367 = Less Or Equal?(x=w644, y=w645) -> (x <= y?=w653:bool)
            n368 = Divide(x=w644, y=w645) -> (x/y=w643:dbl)
            n369 = Or(x=w652, y="Stop saving") -> (x .or. y?=w651:bool)
            n370 = Not(x=w651) -> (.not. x?=w650:bool)
            n371 = Multiply(x=100.0, y=w643) -> (x*y=w642:dbl)
            n372 = And(x=w653, y=w650) -> (x .and. y?=w649:bool)
            n373 = case shown="True" w649 {
              tunnel: w655 -> [w662 w669]
              tunnel: w656 -> [_ w668]
              tunnel: w657 -> [_ w667]
              tunnel: w654 -> [w661 w666]
              tunnel: w648 -> [w659 _]
              tunnel: [0.0 ("Progress") w665] -> w647
              tunnel: w642 -> [_ w665]
              frame False {
                w660 = FALSE
                n374 = Close File(refnum=w662) -> ()  [unwired: 1 in, 2 out]
                n375 = case shown="True" w659 {
                  tunnel: w661 -> [_ w663]
                  frame False {
                  }
                  frame True {
                    n376 = Close File(refnum=w663) -> ()  [unwired: 1 in, 2 out]
                  }
                }
                n377 = call <vilib>:"Beep.vi"() -> ()  [unwired: 12 in]
                n378 = local write "Saving"(w660) -> ()
                n379 = local write "Stop saving"(w660) -> ()
                n380 = local write "Calibrating"(w660) -> ()
              }
              frame True {
                n381 = local read "Calibrating"() -> (w664:bool)
                n382 = case shown="False" w664 {
                  tunnel: w669 -> [w691 w707]
                  tunnel: w668 -> [_ w706]
                  tunnel: w667 -> [w678 w700]
                  tunnel: w666 -> [w677 _]
                  frame False {
                    n383 = local read "Averaging Number"() -> (w685:i32)
                    n384 = Array Subset(array=w678, index (row)=0 ("index"), length (row)=6 ("length")) -> (w674:dbl[][])  [unwired: 2 in]
                    n385 = Array Subset(array=w678, index (row)=6 ("index"), length (row)=2 ("length")) -> (w673:dbl[][])  [unwired: 2 in]
                    n386 = Array Size(array=w673) -> (size(s)=w684:i32[])
                    n387 = Array Size(array=w674) -> (size(s)=w681:i32[])
                    n388 = for {
                      tunnel: w674 -> [w695] mode=indexing
                      tunnel: w685 -> [w697]
                      tunnel: [w696] -> w672 mode=indexing
                      n389 = call "Downsample 1D array.vi"("Ave N"=w697, "Arrray In"=w695) -> ("Array Out"=w696:dbl[])  [unwired: 9 in]
                    }
                    n390 = Multiply Array Elements(1:w681) -> (0:w680:i32)
                    n391 = for {
                      tunnel: w673 -> [w694] mode=indexing
                      tunnel: w685 -> [w693]
                      tunnel: [w692] -> w676 mode=indexing
                      n392 = call "Downsample 1D array.vi"("Ave N"=w693, "Arrray In"=w694) -> ("Array Out"=w692:dbl[])  [unwired: 9 in]
                    }
                    n393 = Multiply Array Elements(1:w684) -> (0:w683:i32)
                    n394 = Divide(x=w680, y=w685) -> (x/y=w686:dbl)
                    n395 = Divide(x=w683, y=w685) -> (x/y=w682:dbl)
                    n396 = Transpose 2D Array(2D array=w672) -> (transposed array=w671:dbl[][])
                    n397 = Transpose 2D Array(2D array=w676) -> (transposed array=w670:dbl[][])
                    "Waveform Chart 3" <- w670
                    n398 = Reshape Array(w671, w686) -> (w675:dbl[])
                    n399 = Reshape Array(w670, w682) -> (w679:dbl[])
                    n400 = call <vilib>:"Write File+ [SGL].vi"("1D array"=w679, "refnum"=w677) -> ()  [unwired: 7 in, 3 out]
                    n401 = call <vilib>:"Write File+ [SGL].vi"("1D array"=w675, "refnum"=w691) -> ()  [unwired: 7 in, 3 out]
                  }
                  frame True {
                    n402 = Array Subset(array=w700, index (row)=0 ("index"), length (row)=6 ("length")) -> (w698:dbl[][])  [unwired: 2 in]
                    n403 = Transpose 2D Array(2D array=w698) -> (transposed array=w704:dbl[][])
                    n404 = Array Size(array=w698) -> (size(s)=w699:i32[])
                    n405 = Multiply Array Elements(1:w699) -> (0:w705:i32)
                    n406 = Reshape Array(w704, w705) -> (w703:dbl[])
                    n407 = call <vilib>:"Write File+ [SGL].vi"("1D array"=w703, "error in (no error)"=w706, "refnum"=w707) -> ()  [unwired: 6 in, 3 out]
                  }
                }
              }
            }
            "Progress" <- w647
          }
        }
      }
    }
    n408 = Divide(x=w195, y=2) -> (x/y=w192:dbl[])
    n409 = call-poly <vilib>:"Mean.vi"("X"=w192) -> ("mean"=w193:dbl)  [unwired: 1 out]
    "Mean force (pN)" <- w193
    n410 = Subtract(x=w193, y=w192) -> (x-y=w191:dbl[])
    n411 = Square(x=w191) -> (x^2=w190:dbl[])
    n412 = call-poly <vilib>:"Mean.vi"("X"=w190) -> ("mean"=w189:dbl)  [unwired: 1 out]
    n413 = Square Root(x=w189) -> (sqrt(x)=→"Force noise (pN)":dbl)
    n414 = local read "Stop"() -> (w417:bool)
  }
  n415 = local write "Progress"(u8 0 ("Progress")) -> ()
  n416 = local write "Calibrating"(FALSE ("Calibrating")) -> ()
  n417 = call "InitializeChamberImage.vi"() -> ("error out"=w102:errorcluster, "IMAQ Session Out"=w103:refnum<k11>, "Display Out"=w104:T7, "Acquired Image"=w9:T7)  [unwired: 8 in]
  n418 = node-c288(i64 10 ("Period"), 2 ("Processor")) -> (w15:T12)  [unwired: 2 in]
  n419 = timed-loop {
    tunnel: w104 -> [w735]
    tunnel: w103 -> [w734]
    tunnel: w102 -> [w733]
    tunnel: [w731] -> w101
    tunnel: [w730] -> w100
    timing: w15 -> [_]
    timing-out: [_] -> w14
    i -> [w732]
    stop <- w726 continue-if-true
    n420 = node-c288() -> ()  [unwired: 1 in, 1 out]
    n421 = call <vilib>:"IMAQ Copy Acquired Buffer.vi"("IMAQ Session In"=w734, "Image In"=w735, "Buffer Number"=w732, "error in (no error)"=w733) -> ("IMAQ Session Out"=w731:refnum<k11>, "Image Out"=→"Chamber":T7, "error out"=w730:errorcluster)  [unwired: 7 in, 2 out]
    "Video Error" <- w730
    n422 = local read "Stop"() -> (w728:bool)
    n423 = Unbundle By Name(w730) -> ("status"=w729:bool)
    n424 = Not Or(1:w728, 2:w729) -> (0:w726:bool)
    "Continue to display?" <- w726
    n425 = node-c288() -> ()  [unwired: 1 in, 1 out]
  }
  n426 = node-c288(w14) -> ()  [unwired: 1 out]
  n427 = call <vilib>:"IMAQ Close.vi"("error in (no error)"=w100, "IMAQ Session In"=w101) -> ("error out"=w108:errorcluster)  [unwired: 9 in]
  n428 = call "IMAQ Dispose"("error in (no error)"=w108) -> ("error out"=w107:errorcluster)  [unwired: 5 in]
  n429 = call-poly "VISA Configure Serial Port"("VISA resource name"=refnum<visa-resource-name> "COM3") -> ("VISA resource name out"=w21:refnum<visa-resource-name>, "error out"=w20:errorcluster)  [unwired: 13 in]
  n430 = node-c288(i64 100 ("Period"), 2 ("Processor")) -> (w23:T12)  [unwired: 2 in]
  n431 = call "IMAQ Dispose"("Image"=w9, "error in (no error)"=w107) -> ("error out"=w106:errorcluster)  [unwired: 4 in]
  n432 = timed-loop {
    timing: w23 -> [_]
    timing-out: [_] -> w22
    tunnel: w21 -> [w738]
    tunnel: w20 -> [w740]
    tunnel: [w738] -> w19
    stop <- w739 stop-if-true
    n433 = node-c288() -> ()  [unwired: 1 in, 1 out]
    n434 = event shown="[7] \"Force FB script\": Value Change" {
      selector: _ -> [_ _ _ _ _ _ _ _ _ _ _]
      dyn-events: _ -> [_ _ _ _ _ _ _ _ _ _ _]
      timeout: _ -> [_ _ _ _ _ _ _ _ _ _ _]
      tunnel: w738 -> [w747 w781 w799 w813 w827 w846 w866 _ _ _ _]
      tunnel: w740 -> [w746 w780 w798 w812 w826 w845 w865 _ _ _ _]
      tunnel: [_ _ _ _ _ _ _ _ _ _ w915] -> w739
      event "Got DNA bead": Value Change {
        n435 = event-data() -> ()  [unwired: 1 in, 5 out]
        n436 = flat-sequence {
          tunnel: w747 -> [w750]
          tunnel: w746 -> [w748]
          tunnel: [w763] -> w745
          tunnel: w745 -> [w766]
          tunnel: [w766] -> w744
          tunnel: w744 -> [w768]
          tunnel: [w768] -> w743
          tunnel: w743 -> [w772]
          tunnel: [w772] -> w742
          tunnel: w742 -> [w774]
          tunnel: [w774] -> w741
          tunnel: w741 -> [w776]
          frame #0 {
            n437 = local read "Saved stage positions"() -> (w751:dbl[][])
            n438 = disable-structure shown="Disabled" {
              frame Disabled {
                n439 = property on="Inject Pump 2" class="Bool (strict)"("Val(Sgnl)"=FALSE ("Inject Pump 2")) -> ()  [unwired: 2 in, 2 out]
              }
              frame Enabled {
              }
            }
            n440 = local write "Stage moving"(TRUE ("Stage moving")) -> ()
            n441 = property on="Trap delta" class="DigNum (strict)"("Val(Sgnl)"="Cal @ Delta (V)") -> ()  [unwired: 2 in, 2 out]
            n442 = call "move to saved stage position.vi"("error in"=w748, "Stage VISA resource name in"=w750, "Position"="Cal stage position", "Saved Stage Positions"=w751) -> ()  [unwired: 2 out]
          }
          frame #1 {
            n443 = local write "Stage moving"(FALSE ("Stage moving")) -> ()
            n444 = call <vilib>:"Beep.vi"() -> ()  [unwired: 12 in]
          }
          frame #2 {
            n445 = Wait (ms)(milliseconds to wait=u32 1000) -> ()  [unwired: 1 out]
          }
          frame #3 {
            n446 = property on="Save cal" class="Bool (strict)"("Val(Sgnl)"=TRUE ("Value (Signaling)")) -> ()  [unwired: 2 in, 2 out]
          }
          frame #4 {
            n447 = Wait (ms)(milliseconds to wait=u32 2000) -> ()  [unwired: 1 out]
          }
          frame #5 {
            n448 = while {
              stop <- w760 stop-if-true
              n449 = local read "Saving"() -> (w761:bool)
              n450 = Not(x=w761) -> (.not. x?=w760:bool)
              n451 = Wait (ms)(milliseconds to wait=u32 100) -> ()  [unwired: 1 out]
            }
          }
          frame #6 {
            n452 = Wait (ms)(milliseconds to wait=u32 2000) -> ()  [unwired: 1 out]
          }
          frame #7 {
            # "Only continue if there is no buffer\noverflow error"
            n453 = local read "Buffer Overflow"() -> (w764:bool)
            n454 = Not(x=w764) -> (.not. x?=w763:bool)
            n455 = case shown="True" w763 {
              frame False {
              }
              frame True {
                n456 = property on="Raster scan" class="Bool (strict)"("Val(Sgnl)"=TRUE ("Value (Signaling)")) -> ()  [unwired: 2 in, 2 out]
              }
            }
          }
          frame #8 {
            n457 = case shown="True" w766 {
              frame False {
              }
              frame True {
                n458 = Wait (ms)(milliseconds to wait=u32 2000) -> ()  [unwired: 1 out]
              }
            }
          }
          frame #9 {
            n459 = case shown="True" w768 {
              frame False {
              }
              frame True {
                n460 = while {
                  stop <- w770 stop-if-true
                  n461 = local read "Saving"() -> (w771:bool)
                  n462 = Not(x=w771) -> (.not. x?=w770:bool)
                  n463 = Wait (ms)(milliseconds to wait=u32 100) -> ()  [unwired: 1 out]
                }
              }
            }
          }
          frame #10 {
            n464 = case shown="True" w772 {
              frame False {
              }
              frame True {
                n465 = property on="Read Cal" class="Bool (strict)"("Val(Sgnl)"=TRUE ("Value (Signaling)")) -> ()  [unwired: 2 in, 2 out]
              }
            }
          }
          frame #11 {
            n466 = case shown="True" w774 {
              frame False {
              }
              frame True {
                n467 = Wait (ms)(milliseconds to wait=u32 1000) -> ()  [unwired: 1 out]
              }
            }
          }
          frame #12 {
            n468 = case shown="True" w776 {
              frame False {
              }
              frame True {
                n469 = property on="Fish" class="Bool (strict)"("Val(Sgnl)"=TRUE ("Value (Signaling)")) -> ()  [unwired: 2 in, 2 out]
              }
            }
          }
        }
      }
      event "Dump beads": Value Change {
        n470 = event-data() -> ()  [unwired: 1 in, 5 out]
        n471 = flat-sequence {
          tunnel: w780 -> [w784]
          tunnel: w781 -> [w785]
          tunnel: [w785] -> w779
          tunnel: [w784] -> w778
          tunnel: w779 -> [w787]
          tunnel: w778 -> [w786]
          frame #0 {
            w783 = FALSE ("Fish")
            n472 = local read "Saving"() -> (w782:bool)
            n473 = local write "Force Feedback"(w783) -> ()
            n474 = local write "Dump beads"(w783) -> ()
            n475 = property on="Stop saving" class="Bool (strict)"("Val(Sgnl)"=w782) -> ()  [unwired: 2 in, 2 out]
            n476 = local write "Fish"(w783) -> ()
          }
          frame #1 {
            n477 = local read "Saved stage positions"() -> (w789:dbl[][])
            n478 = local write "Stage moving"(TRUE ("Stage moving")) -> ()
            n479 = call "move to saved stage position.vi"("error in"=w786, "Stage VISA resource name in"=w787, "Position"=5, "Saved Stage Positions"=w789) -> ()  [unwired: 2 out]
          }
          frame #2 {
            n480 = local read "Shutter 1 (B)"() -> (w793:bool)
            n481 = local read "Shutter 2 (A)"() -> (w792:bool)
            n482 = call <vilib>:"Beep.vi"() -> ()  [unwired: 12 in]
            n483 = case shown="True" w793 {
              frame False {
              }
              frame True {
                n484 = property on="Shutter 1 (B)" class="Bool (strict)"("Val(Sgnl)"=FALSE ("Value (Signaling)")) -> ()  [unwired: 2 in, 2 out]
              }
            }
            n485 = case shown="True" w792 {
              frame False {
              }
              frame True {
                n486 = property on="Shutter 2 (A)" class="Bool (strict)"("Val(Sgnl)"=FALSE) -> ()  [unwired: 2 in, 2 out]
              }
            }
            n487 = local write "Stage moving"(FALSE ("Stage moving")) -> ()
            n488 = local write "Tether"(FALSE ("Tether")) -> ()
          }
          frame #3 {
            n489 = property on="Move Cap. 2 (ADig Top)" class="Bool (strict)"("Val(Sgnl)"=TRUE ("Value (Signaling)")) -> ()  [unwired: 2 in, 2 out]
          }
        }
      }
      event "Move Cap. 2 (ADig Top)": Value Change {
        n490 = event-data() -> ()  [unwired: 1 in, 5 out]
        n491 = flat-sequence {
          tunnel: w799 -> [w801]
          tunnel: w798 -> [w800]
          frame #0 {
            n492 = local read "Saved stage positions"() -> (w803:dbl[][])
            n493 = local write "Move Cap. 2 (ADig Top)"(FALSE ("Move Cap. 2 (ADig Top)")) -> ()
            n494 = local write "Stage moving"(TRUE ("Stage moving")) -> ()
            n495 = call "move to saved stage position.vi"("error in"=w800, "Stage VISA resource name in"=w801, "Position"=2, "Saved Stage Positions"=w803) -> ()  [unwired: 2 out]
          }
          frame #1 {
            # "Make sure you don't reverse\nwhich is ON and OFF"
            n496 = local read "Cal @ Delta (V)"() -> (w807:dbl)
            n497 = local write "Stage moving"(FALSE ("Stage moving")) -> ()
            n498 = call <vilib>:"Beep.vi"() -> ()  [unwired: 12 in]
            n499 = property on="Trap delta" class="DigNum (strict)"("Val(Sgnl)"=w807) -> ()  [unwired: 2 in, 2 out]
            n500 = disable-structure shown="Disabled" {
              frame Disabled {
                n501 = property on="Inject Pump 1" class="Bool (strict)"("Val(Sgnl)"=TRUE ("Inject Pump 2")) -> ()  [unwired: 2 in, 2 out]
              }
              frame Enabled {
              }
            }
            n502 = local read "Shutter 2 (A)"() -> (w806:bool)
            n503 = case shown="False" w806 {
              frame False {
                n504 = property on="Shutter 2 (A)" class="Bool (strict)"("Val(Sgnl)"=TRUE ("Value (Signaling)")) -> ()  [unwired: 2 in, 2 out]
              }
              frame True {
              }
            }
          }
        }
      }
      event "Got ADig bead": Value Change {
        n505 = event-data() -> ()  [unwired: 1 in, 5 out]
        n506 = flat-sequence {
          tunnel: w813 -> [w816]
          tunnel: w812 -> [w815]
          frame #0 {
            n507 = local read "Saved stage positions"() -> (w818:dbl[][])
            n508 = property on="Inject Pump 1" class="Bool (strict)"("Val(Sgnl)"=FALSE ("Inject Pump 2")) -> ()  [unwired: 2 in, 2 out]
            n509 = local write "Stage moving"(TRUE ("Stage moving")) -> ()
            n510 = call "move to saved stage position.vi"("error in"=w815, "Stage VISA resource name in"=w816, "Position"=1, "Saved Stage Positions"=w818) -> ()  [unwired: 2 out]
          }
          frame #1 {
            n511 = local read "Shutter 1 (B)"() -> (w820:bool)
            n512 = disable-structure shown="Disabled" {
              frame Disabled {
                n513 = property on="Inject Pump 2" class="Bool (strict)"("Val(Sgnl)"=TRUE ("Inject Pump 2")) -> ()  [unwired: 2 in, 2 out]
              }
              frame Enabled {
              }
            }
            n514 = local write "Stage moving"(FALSE ("Stage moving")) -> ()
            n515 = case shown="False" w820 {
              frame False {
                n516 = property on="Shutter 1 (B)" class="Bool (strict)"("Val(Sgnl)"=TRUE ("Value (Signaling)")) -> ()  [unwired: 2 in, 2 out]
              }
              frame True {
              }
            }
            n517 = call <vilib>:"Beep.vi"() -> ()  [unwired: 12 in]
          }
        }
        n518 = local write "Got ADig bead"(FALSE ("Got ADig bead")) -> ()
      }
      event "Set Position 1", "Set Position 2", "Set Position 3", "Set Position 4", "Set Position 5": Value Change {
        n519 = event-data() -> ()  [unwired: 1 in, 5 out]
        n520 = Build Array("Set Position 1", "Set Position 2", "Set Position 3", "Set Position 4", "Set Position 5") -> (w839:bool[])
        n521 = Boolean Array To Number(Boolean array=w839) -> (number=w838:u32)
        n522 = call "Read Stage Position.vi"("error in"=w826, "VISA resource name in"=w827) -> ("Current Position"=w824:cluster{dbl, dbl, dbl}, "error out"=→"Stage error":errorcluster)  [unwired: 1 in, 1 out]
        n523 = Logarithm Base 2(1:w838) -> (0:w832:dbl)
        n524 = Cluster To Array(cluster=w824) -> (array=w834:dbl[])
        n525 = Increment(x=w832) -> (x+1=w835:dbl)
        n526 = Build Array (concatenate)(w835, w834) -> (w833:dbl[])
        n527 = Replace Array Subset(array="Saved stage positions", new element=w833, index (row)=w832) -> (w836:dbl[][])  [unwired: 1 in]
        n528 = local write "Saved stage positions"(w836) -> ()
      }
      event "Move to Position 2", "Move to Position 4", "Move to Position 3", "Move to Position 5", "Move to Position 1": Value Change {
        n529 = event-data() -> ()  [unwired: 1 in, 5 out]
        n530 = Build Array("Move to Position 1", "Move to Position 2", "Move to Position 3", "Move to Position 4", "Move to Position 5") -> (w849:bool[])
        n531 = Boolean Array To Number(Boolean array=w849) -> (number=w848:u32)
        n532 = Logarithm Base 2(1:w848) -> (0:w847:dbl)
        n533 = flat-sequence {
          tunnel: w847 -> [w854]
          tunnel: w846 -> [w853]
          tunnel: w845 -> [w852]
          frame #0 {
            n534 = local read "Saved stage positions"() -> (w855:dbl[][])
            n535 = Increment(x=w854) -> (x+1=w851:dbl)
            n536 = call "move to saved stage position.vi"("error in"=w852, "Stage VISA resource name in"=w853, "Position"=w851, "Saved Stage Positions"=w855) -> ()  [unwired: 2 out]
            "Stage moving" <- TRUE ("Stage moving")
          }
          frame #1 {
            n537 = call <vilib>:"Beep.vi"() -> ()  [unwired: 12 in]
            n538 = local write "Stage moving"(FALSE ("Stage moving")) -> ()
          }
        }
      }
      event "Dip": Value Change {
        n539 = event-data() -> ()  [unwired: 1 in, 5 out]
        n540 = local write "Dip"(FALSE ("Dip")) -> ()
        n541 = flat-sequence {
          tunnel: w866 -> [w868]
          tunnel: w865 -> [w867]
          tunnel: [w869] -> w863
          tunnel: [w868] -> w861
          tunnel: [w867] -> w859
          tunnel: [w877] -> w864
          tunnel: w863 -> [w877]
          tunnel: [w876] -> w862
          tunnel: w861 -> [w876]
          tunnel: [w875] -> w860
          tunnel: w859 -> [w875]
          tunnel: w864 -> [w894]
          tunnel: w862 -> [w893]
          tunnel: w860 -> [w892]
          frame #0 {
            n542 = local read "Saved stage positions"() -> (w869:dbl[][])
            n543 = local write "Stage moving"(TRUE) -> ()
            n544 = call "move to saved stage position.vi"("error in"=w867, "Stage VISA resource name in"=w868, "Position"="Dip position", "Saved Stage Positions"=w869) -> ()  [unwired: 2 out]
          }
          frame #1 {
            n545 = node-c288() -> (w874:T12)  [unwired: 4 in]
            n546 = timed-loop {
              timing: w874 -> [_]
              timing-out: [_] -> w873
              i -> [w885]
              stop <- w881 stop-if-true
              n547 = node-c288() -> ()  [unwired: 1 in, 1 out]
              n548 = Greater Or Equal?(x=w885, y="Dip duration") -> (x >= y?=w880:bool)
              n549 = Or(x=w880, y="Cancel dwell") -> (x .or. y?=w878:bool)
              n550 = Not(x="Pause dwell") -> (.not. x?=w882:bool)
              n551 = node-c288() -> ()  [unwired: 1 in, 1 out]
              n552 = And(x=w882, y=w878) -> (x .and. y?=w881:bool)
              "Dip time" <- w885
            }
            n553 = local write "Stage moving"(FALSE ("Stage moving")) -> ()
            n554 = node-c288(w873) -> ()  [unwired: 1 out]
          }
          frame #2 {
            n555 = local write "Cancel dwell"(FALSE ("Cancel dwell")) -> ()
            n556 = call "move to saved stage position.vi"("error in"=w892, "Stage VISA resource name in"=w893, "Position"="Return position", "Saved Stage Positions"=w894) -> ()  [unwired: 2 out]
          }
          frame #3 {
            n557 = local write "Stage moving"(FALSE ("Stage moving")) -> ()
          }
        }
      }
      event "Force FB script": Value Change {
        n558 = event-data() -> ()  [unwired: 1 in, 5 out]
        n559 = flat-sequence {
          frame #0 {
            n560 = disable-structure shown="Disabled" {
              frame Disabled {
                n561 = local read "# Samples/channel"() -> (w898:i32)
                n562 = local write "# Samples/channel (in)"(w898) -> ()
              }
              frame Enabled {
              }
            }
            n563 = local write "Force FB script"(FALSE ("Force FB script")) -> ()
            n564 = property on="Trap delta" class="DigNum (strict)"("Val(Sgnl)"="Start trap delta (V)") -> ()  [unwired: 2 in, 2 out]
          }
          frame #1 {
            n565 = Wait (ms)(milliseconds to wait=u32 500) -> ()  [unwired: 1 out]
          }
          frame #2 {
            n566 = property on="Set reading to\nsetpoint" class="Bool (strict)"("Val(Sgnl)"=TRUE ("Value (Signaling)")) -> ()  [unwired: 2 in, 2 out]
          }
          frame #3 {
            n567 = Wait (ms)(milliseconds to wait=u32 300) -> ()  [unwired: 1 out]
          }
          frame #4 {
            n568 = local write "Force Feedback"(TRUE ("Force Feedback")) -> ()
          }
          frame #5 {
            n569 = property on="Save Data" class="Bool (strict)"("Val(Sgnl)"=TRUE ("Value (Signaling)")) -> ()  [unwired: 2 in, 2 out]
          }
          frame #6 {
            n570 = Multiply(x="Wait before dip (s)", y=1000) -> (x*y=w904:dbl)
            n571 = Wait (ms)(milliseconds to wait=w904) -> ()  [unwired: 1 out]
          }
          frame #7 {
            n572 = case shown="True" "Start dipping after?" {
              selector: "Start dipping after?" -> [_ w908]
              frame False {
              }
              frame True {
                n573 = property on="Dip" class="Bool (strict)"("Val(Sgnl)"=w908) -> ()  [unwired: 2 in, 2 out]
              }
            }
          }
        }
      }
      event "Move 0": Value Change {
        n574 = event-data() -> ()  [unwired: 1 in, 5 out]
        n575 = local write "Move 0"(FALSE) -> ()
        n576 = call "HalfWavePlate.vi"("Degrees"="\"Degrees\" 0", "Motor"=0) -> ()  [unwired: 1 in]
      }
      event "Move 1": Value Change {
        n577 = event-data() -> ()  [unwired: 1 in, 5 out]
        n578 = local write "Move 1"(FALSE) -> ()
        n579 = call "HalfWavePlate.vi"("Degrees"="\"Degrees\" 1", "Motor"=1) -> ()  [unwired: 1 in]
      }
      event "Stop": Value Change {
        n580 = event-data() -> ()  [unwired: 1 in, 5 out]
        n581 = local read "Stop"() -> (w915:bool)
      }
    }
    n582 = node-c288() -> ()  [unwired: 1 in, 1 out]
  }
  n583 = call <vilib>:"Simple Error Handler.vi"("error in (no error)"=w106) -> ()  [unwired: 4 in, 5 out]
  n584 = node-c288(2 ("Processor")) -> (w76:T12)  [unwired: 3 in]
  n585 = node-c288(2 ("Processor")) -> (w27:T12)  [unwired: 3 in]
  n586 = timed-loop {
    timing: w76 -> [_]
    timing-out: [_] -> w75
    stop <- w918 stop-if-true
    n587 = node-c288() -> ()  [unwired: 1 in, 1 out]
    n588 = case shown="\"Current Saved Data\"" "Tab Control" {
      frame "Control" {
        n589 = case shown="True" "Start" {
          frame False {
          }
          frame True {
            w931 = T15 3 items=["no dialog", "OK message", "continue or stop message", "OK message + warnings", "continue/stop + warnings"] ("type of dialog (OK msg:1)")
            n590 = call "InitializeAcquireFF.vi"("DAQ Rate"="DAQ Rate", "Averaging Number"="Averaging Number", "Sampling Rate"="Sampling Rate") -> ("error out"=w925:errorcluster, "task out"=w924:refnum<k21>, "Final Sampling Rate"=→"Final Sampling Rate":dbl)  [unwired: 4 in, 2 out]
            n591 = while {
              tunnel: [w943] -> w930
              tunnel: [w942] -> w923
              tunnel: "Averaging Number" -> [w941]
              tunnel: w925 -> [w940]
              tunnel: w924 -> [w938]
              stop <- w939 continue-if-true
              n592 = call "Acquire2_QPD.vi"("task/channels in"=w938, "Save Data?"=FALSE ("Take Data?"), "Averaging Number"=w941, "error in"=w940) -> ("PSD 1"=→"PSD 1":cluster{dbl[], dbl[]}, "PSD 1 Sum"=→"PSD 1 Sum":dbl, "PSD 2"=→"PSD 2":cluster{dbl[], dbl[]}, "PSD 2 Sum"=→"PSD 2 Sum":dbl, "task out"=w943:refnum<k21>, "error out"=w942:errorcluster)  [unwired: 14 in, 4 out]
              n593 = local read "Start"() -> (w939:bool)
            }
            n594 = call <vilib>:"DAQmx Clear Task.vi"("task in"=w930, "error in"=w923) -> ("error out"=w932:errorcluster)  [unwired: 13 in]
            n595 = call <vilib>:"Simple Error Handler.vi"("type of dialog (OK msg:1)"=w931, "error in (no error)"=w932) -> ()  [unwired: 3 in, 5 out]
          }
        }
      }
      frame "Current Saved Data" {
      }
      frame "Data Acquisition" {
      }
      frame "Raw QPD Data" {
      }
    }
    n596 = local read "Stop"() -> (w918:bool)
    n597 = node-c288() -> ()  [unwired: 1 in, 1 out]
  }
  n598 = timed-loop {
    timing: w27 -> [_]
    timing-out: [_] -> w26
    stop <- w944 stop-if-true
    n599 = node-c288() -> ()  [unwired: 1 in, 1 out]
    n600 = event shown="[0] \"Pause Mouse/Mirror Connection\": Value Change" {
      selector: _ -> [_ _]
      dyn-events: _ -> [_ _]
      timeout: _ -> [_ _]
      tunnel: [w1037 _] -> w945
      tunnel: [_ w1038] -> w944
      event "Pause Mouse/Mirror Connection": Value Change {
        n601 = event-data() -> ("NewVal"=w1037:bool)  [unwired: 1 in]
      }
      event "Stop": Value Change {
        n602 = event-data() -> ("NewVal"=w1038:bool)  [unwired: 1 in]
      }
    }
    n603 = case shown="True" w945 {
      frame False {
      }
      frame True {
        n604 = call "InitializeMouseControl.vi"() -> ("error out 2"=w954:errorcluster, "task out"=w955:refnum<k21>, "error out"=w957:errorcluster, "device ID"=w956:refnum<k1>)  [unwired: 8 in]
        n605 = while {
          tunnel: w957 -> [w969]
          tunnel: w956 -> [w968]
          tunnel: w955 -> [w967]
          tunnel: w954 -> [w966]
          tunnel: [w965] -> w952
          tunnel: [w964] -> w951
          tunnel: [w963] -> w948
          tunnel: [w962] -> w949
          stop <- w961 stop-if-true
          n606 = case shown="True" "Use Mouse to Move Trap?" {
            tunnel: w968 -> [w976 w999]
            tunnel: w969 -> [w975 w998]
            tunnel: w967 -> [w974 w997]
            tunnel: w966 -> [w973 w996]
            tunnel: [w976 w995] -> w963
            tunnel: [w975 w994] -> w962
            tunnel: [w974 w993] -> w965
            tunnel: [w973 w992] -> w964
            frame False {
              (unwired) FALSE ("button 1")
            }
            frame True {
              w987 = 0.0 ("y")
              w989 = 10
              n607 = local read "Deflection"() -> (w1000:T4)
              n608 = call-poly <vilib>:"Acquire Input Data.vi"("device ID"=w999, "error in (no error)"=w998) -> ("device ID"=w995:refnum<k1>, "button info"=w1013:T16, "error out"=w994:errorcluster)  [unwired: 14 in, 1 out]
              n609 = Unbundle By Name(w1000) -> ("Horizontal"=w1002:i32, "Vertical"=w1001:i32)
              n610 = local read "Saved voltage"() -> (w978:cluster{dbl, dbl})
              n611 = Divide(x=w1002, y=30) -> (x/y=w1005:dbl)
              n612 = Divide(x=w1001, y=-20) -> (x/y=w1006:dbl)
              n613 = Unbundle By Name(w1013) -> ("button 1"=w991:bool, "button 2"=w1007:bool)
              n614 = Bundle(w1005, w1006) -> (w983:cluster{dbl, dbl})  [unwired: 1 in]
              n615 = local write "Reference Voltage"(w983) -> ()
              n616 = Add(x=w983, y=w978) -> (x+y=w1011:cluster{dbl, dbl})
              n617 = case shown="True" w991 {
                frame False {
                  n618 = stacked-sequence {
                    frame #0 {
                      n619 = local write "CoordinatesMousePressed"(T4 {"Horizontal"=0, "Vertical"=0} ("Coords when pressed")) -> ()
                      n620 = local write "Deflection"(T4 {"Horizontal"=0, "Vertical"=0} ("deflaction")) -> ()
                    }
                  }
                }
                frame True {
                  n621 = local read "CoordinatesMousePressed"() -> (w1036:T4)
                  n622 = local read "Real Coordinates"() -> (w1035:cluster{"Horizontal":i32, "Vertical":i32})
                  n623 = Subtract(x=w1035, y=w1036) -> (x-y=w1034:T4)
                  n624 = local write "Deflection"(w1034) -> ()
                }
              }
              n625 = Unbundle(w1011) -> (w988:dbl, w979:dbl)
              n626 = case shown="True" w1007 {
                frame False {
                }
                frame True {
                  n627 = local read "Reference Voltage"() -> (w1017:cluster{dbl, dbl})
                  n628 = local read "Saved voltage"() -> (w1015:cluster{dbl, dbl})
                  n629 = Add(x=w1017, y=w1015) -> (x+y=→"Saved voltage":cluster{dbl, dbl})
                  n630 = local read "Real Coordinates"() -> (w1016:cluster{"Horizontal":i32, "Vertical":i32})
                  n631 = local write "CoordinatesMousePressed"(w1016) -> ()
                }
              }
              n632 = Less?(x=w988, y=w989) -> (x < y?=w986:bool)
              n633 = Greater?(x=w988, y=w987) -> (0:w985:bool)
              n634 = Greater?(x=w979, y=w987) -> (0:w981:bool)
              n635 = Less?(x=w979, y=w989) -> (x < y?=w982:bool)
              n636 = And(x=w981, y=w982) -> (x .and. y?=w980:bool)
              n637 = And(x=w986, y=w985) -> (x .and. y?=w984:bool)
              n638 = case shown="False" w980 {
                tunnel: [w1027 w1031] -> w990
                tunnel: w979 -> [w1025 w1031]
                frame False {
                  n639 = Greater?(x=w1025, y=10.0) -> (0:w1028:bool)
                  n640 = case shown="True" w1028 {
                    tunnel: [0.0 10.0] -> w1027
                    frame False {
                    }
                    frame True {
                    }
                  }
                }
                frame True {
                }
              }
              n641 = case shown="False" w984 {
                tunnel: w988 -> [w1019 w1024]
                tunnel: [w1020 w1024] -> w1012
                frame False {
                  n642 = Greater?(x=w1019, y=10.0) -> (0:w1021:bool)
                  n643 = case shown="True" w1021 {
                    tunnel: [0.0 10.0] -> w1020
                    frame False {
                    }
                    frame True {
                    }
                  }
                }
                frame True {
                }
              }
              n644 = Bundle(w1012, w990) -> (w977:cluster{dbl, dbl})  [unwired: 1 in]
              n645 = Cluster To Array(cluster=w977) -> (array=w1008:dbl[])
              n646 = call-poly <vilib>:"DAQmx Write.vi"("task/channels in"=w997, "data"=w1008, "error in"=w996) -> ("task out"=w1010:refnum<k21>, "error out"=w1009:errorcluster)  [unwired: 10 in, 1 out]
              n647 = call <vilib>:"DAQmx Is Task Done.vi"("task/channels in"=w1010, "error in"=w1009) -> ("task out"=w993:refnum<k21>, "error out"=w992:errorcluster)  [unwired: 11 in, 1 out]
            }
          }
          n648 = event shown="[0] \"Pane\": Mouse Move" {
            selector: _ -> [_ _ _]
            dyn-events: _ -> [_ _ _]
            timeout: _ -> [_ _ _]
            event Mouse Move {
              n649 = event-data() -> ("Coords"=w971:T4)  [unwired: 1 in]
              n650 = local write "Real Coordinates"(w971) -> ()
            }
            event Mouse Down {
              n651 = event-data() -> ("Coords"=w972:T4)  [unwired: 1 in]
              n652 = local write "CoordinatesMousePressed"(w972) -> ()
            }
            event "Pause Mouse/Mirror Connection": Value Change {
              n653 = event-data() -> ()  [unwired: 1 in, 3 out]
            }
          }
          n654 = local read "Stop"() -> (w958:bool)
          n655 = Not(x="Pause Mouse/Mirror Connection") -> (.not. x?=w959:bool)
          n656 = Or(x=w959, y=w958) -> (x .or. y?=w961:bool)
        }
        n657 = call <vilib>:"DAQmx Clear Task.vi"("task in"=w952, "error in"=w951) -> ("error out"=w953:errorcluster)  [unwired: 13 in]
        n658 = call <vilib>:"Simple Error Handler.vi"("error in (no error)"=w953) -> ()  [unwired: 4 in, 5 out]
        n659 = call-poly <vilib>:"Close Input Device.vi"("error in (no error)"=w949, "device ID"=w948) -> ("error out"=w950:errorcluster)  [unwired: 8 in]
        n660 = call <vilib>:"Simple Error Handler.vi"("error in (no error)"=w950) -> ()  [unwired: 4 in, 5 out]
      }
    }
    n661 = node-c288() -> ()  [unwired: 1 in, 1 out]
  }
  n662 = call-poly <vilib>:"DAQmx Create Virtual Channel.vi"("lines"=w93) -> ("task out"=w92:refnum<k21>)  [unwired: 13 in, 1 out]
  n663 = call-poly <vilib>:"DAQmx Create Virtual Channel.vi"("lines"=w96) -> ("task out"=w95:refnum<k21>)  [unwired: 13 in, 1 out]
  n664 = node-c288(i64 100 ("Period")) -> (w90:T12)  [unwired: 3 in]
  n665 = timed-loop {
    tunnel: w92 -> [w1041]
    tunnel: [w1040] -> w91
    tunnel: w95 -> [w1043]
    tunnel: [w1042] -> w94
    timing: w90 -> [_]
    timing-out: [_] -> w89
    stop <- w1039 stop-if-true
    n666 = node-c288() -> ()  [unwired: 1 in, 1 out]
    n667 = event shown="[1] \"Shutter 2 (A)\": Value Change" {
      selector: _ -> [_ _ _]
      dyn-events: _ -> [_ _ _]
      timeout: _ -> [_ _ _]
      tunnel: w1043 -> [w1047 _ _]
      tunnel: [w1046 _ _] -> w1042
      tunnel: w1041 -> [_ w1067 _]
      tunnel: [_ w1065 _] -> w1040
      tunnel: [_ _ w1084] -> w1039
      event "Shutter 1 (B)": Value Change {
        n668 = event-data() -> ()  [unwired: 1 in, 1 out]
        n669 = flat-sequence {
          tunnel: [w1053] -> w1050
          tunnel: w1047 -> [w1052]
          tunnel: [w1057] -> w1049
          tunnel: [w1060] -> w1048
          tunnel: w1050 -> [w1055]
          tunnel: w1049 -> [w1064]
          tunnel: w1048 -> [w1062]
          tunnel: [w1061] -> w1046
          frame #0 {
            n670 = call-poly <vilib>:"DAQmx Write.vi"("task/channels in"=w1052, "data"=FALSE) -> ("task out"=w1053:refnum<k21>)  [unwired: 11 in, 2 out]
            n671 = Wait (ms)(milliseconds to wait=100) -> ()  [unwired: 1 out]
          }
          frame #1 {
            n672 = Or(x="Shutter 1 (B)", y=TRUE) -> (x .or. y?=w1057:bool)
            n673 = call-poly <vilib>:"DAQmx Write.vi"("task/channels in"=w1055, "data"=w1057) -> ("task out"=w1060:refnum<k21>)  [unwired: 11 in, 2 out]
            n674 = Wait (ms)(milliseconds to wait=100) -> ()  [unwired: 1 out]
          }
          frame #2 {
            n675 = Not(x=w1064) -> (.not. x?=w1063:bool)
            n676 = call-poly <vilib>:"DAQmx Write.vi"("task/channels in"=w1062, "data"=w1063) -> ("task out"=w1061:refnum<k21>)  [unwired: 11 in, 2 out]
          }
        }
      }
      event "Shutter 2 (A)": Value Change {
        n677 = event-data() -> ()  [unwired: 1 in, 1 out]
        n678 = flat-sequence {
          tunnel: w1067 -> [w1072]
          tunnel: [w1071] -> w1066
          tunnel: [w1076] -> w1069
          tunnel: [w1079] -> w1068
          tunnel: w1066 -> [w1074]
          tunnel: w1069 -> [w1083]
          tunnel: w1068 -> [w1081]
          tunnel: [w1080] -> w1065
          frame #0 {
            n679 = call-poly <vilib>:"DAQmx Write.vi"("task/channels in"=w1072, "data"=FALSE) -> ("task out"=w1071:refnum<k21>)  [unwired: 11 in, 2 out]
            n680 = Wait (ms)(milliseconds to wait=100) -> ()  [unwired: 1 out]
          }
          frame #1 {
            n681 = Or(x="Shutter 2 (A)", y=TRUE) -> (x .or. y?=w1076:bool)
            n682 = call-poly <vilib>:"DAQmx Write.vi"("task/channels in"=w1074, "data"=w1076) -> ("task out"=w1079:refnum<k21>)  [unwired: 11 in, 2 out]
            n683 = Wait (ms)(milliseconds to wait=100) -> ()  [unwired: 1 out]
          }
          frame #2 {
            n684 = Not(x=w1083) -> (.not. x?=w1082:bool)
            n685 = call-poly <vilib>:"DAQmx Write.vi"("task/channels in"=w1081, "data"=w1082) -> ("task out"=w1080:refnum<k21>)  [unwired: 11 in, 2 out]
          }
        }
      }
      event "Stop": Value Change {
        n686 = event-data() -> ("NewVal"=w1084:bool)  [unwired: 1 in, 5 out]
      }
    }
    n687 = node-c288() -> ()  [unwired: 1 in, 1 out]
  }
  n688 = node-c288(w89) -> ()  [unwired: 1 out]
  n689 = node-c288(w75) -> ()  [unwired: 1 out]
  n690 = call <vilib>:"DAQmx Clear Task.vi"("task in"=w91) -> ()  [unwired: 14 in, 1 out]
  n691 = call <vilib>:"DAQmx Clear Task.vi"("task in"=w94) -> ()  [unwired: 14 in, 1 out]
  n692 = node-c288(w26) -> ()  [unwired: 1 out]
  n693 = node-c288(w22) -> ()  [unwired: 1 out]
  n694 = VISA Close(VISA resource name=w19) -> (error out=w105:errorcluster)  [unwired: 1 in]
  n695 = disable-structure shown="Disabled" {
    frame Disabled {
      n696 = node-c288(2 ("Processor")) -> (w1088:T12)  [unwired: 3 in]
      n697 = timed-loop "Pump Control" {
        timing: w1088 -> [_]
        timing-out: [_] -> w1087
        tunnel: refnum<visa-resource-name> "COM6" ("VISA resource name") -> [w1090]
        stop <- w1089 stop-if-true
        n698 = node-c288() -> ()  [unwired: 1 in, 1 out]
        n699 = event shown="[4] \"Inject Pump 1\": Value Change" {
          selector: _ -> [_ _ _ _ _ _ _ _ _]
          dyn-events: _ -> [_ _ _ _ _ _ _ _ _]
          timeout: _ -> [_ _ _ _ _ _ _ _ _]
          tunnel: w1090 -> [w1098 w1194 _ w1270 w1398 w1541 w1586 w1644 w1703]
          tunnel: [_ _ w1269 _ _ _ _ _ _] -> w1089
          event "Flush Pump 1": Value Change {
            w1099 = "\r"
            n700 = event-data() -> ()  [unwired: 1 in, 5 out]
            n701 = call-poly "VISA Configure Serial Port"("VISA resource name"=w1098) -> ("VISA resource name out"=w1112:refnum<visa-resource-name>, "error out"=w1113:errorcluster)  [unwired: 13 in]
            n702 = local read "Write Wait"() -> (w1091:i32)
            n703 = Concatenate Strings("enter pump1", w1099) -> (w1100:string)
            n704 = flat-sequence {
              tunnel: w1113 -> [w1132]
              tunnel: w1112 -> [w1134]
              tunnel: [w1133] -> w1129
              tunnel: [w1131] -> w1128
              tunnel: w1100 -> [w1130]
              tunnel: w1129 -> [w1137]
              tunnel: [w1137] -> w1127
              tunnel: w1128 -> [w1136]
              tunnel: [w1136] -> w1126
              tunnel: w1091 -> [w1135]
              tunnel: [w1142] -> w1125
              tunnel: w1105 -> [w1141]
              tunnel: [w1138] -> w1124
              tunnel: w1127 -> [w1140]
              tunnel: w1126 -> [w1139]
              tunnel: w1125 -> [w1145]
              tunnel: [w1145] -> w1123
              tunnel: [w1144] -> w1122
              tunnel: w1124 -> [w1144]
              tunnel: w1091 -> [w1143]
              tunnel: w1123 -> [w1150]
              tunnel: [w1149] -> w1121
              tunnel: w1108 -> [w1148]
              tunnel: w1122 -> [w1147]
              tunnel: [w1146] -> w1120
              tunnel: w1121 -> [w1153]
              tunnel: [w1153] -> w1119
              tunnel: [w1152] -> w1118
              tunnel: w1120 -> [w1152]
              tunnel: w1091 -> [w1151]
              tunnel: w1119 -> [w1158]
              tunnel: [w1157] -> w1117
              tunnel: w1111 -> [w1156]
              tunnel: w1118 -> [w1155]
              tunnel: [w1154] -> w1116
              tunnel: [w1161] -> w1115
              tunnel: w1117 -> [w1161]
              tunnel: [w1160] -> w1114
              tunnel: w1116 -> [w1160]
              tunnel: w1091 -> [w1159]
              tunnel: w1115 -> [w1166]
              tunnel: w1114 -> [w1163]
              tunnel: [w1165] -> w1094
              tunnel: [w1164] -> w1092
              tunnel: [w1171] -> w1095
              tunnel: w1094 -> [w1171]
              tunnel: [w1170] -> w1093
              tunnel: w1092 -> [w1170]
              tunnel: w1091 -> [w1169]
              tunnel: w1095 -> [w1173]
              tunnel: w1093 -> [w1172]
              frame #0 {
                n705 = VISA Write(VISA resource name=w1134, write buffer=w1130, error in (no error)=w1132) -> (VISA resource name out=w1133:refnum<visa-resource-name>, error out=w1131:errorcluster)  [unwired: 1 out]
              }
              frame #1 {
                n706 = Wait (ms)(milliseconds to wait=w1135) -> ()  [unwired: 1 out]
              }
              frame #2 {
                n707 = VISA Write(VISA resource name=w1140, write buffer=w1141, error in (no error)=w1139) -> (VISA resource name out=w1142:refnum<visa-resource-name>, error out=w1138:errorcluster)  [unwired: 1 out]
              }
              frame #3 {
                n708 = Wait (ms)(milliseconds to wait=w1143) -> ()  [unwired: 1 out]
              }
              frame #4 {
                n709 = VISA Write(VISA resource name=w1150, write buffer=w1148, error in (no error)=w1147) -> (VISA resource name out=w1149:refnum<visa-resource-name>, error out=w1146:errorcluster)  [unwired: 1 out]
              }
              frame #5 {
                n710 = Wait (ms)(milliseconds to wait=w1151) -> ()  [unwired: 1 out]
              }
              frame #6 {
                n711 = VISA Write(VISA resource name=w1158, write buffer=w1156, error in (no error)=w1155) -> (VISA resource name out=w1157:refnum<visa-resource-name>, error out=w1154:errorcluster)  [unwired: 1 out]
              }
              frame #7 {
                n712 = Wait (ms)(milliseconds to wait=w1159) -> ()  [unwired: 1 out]
              }
              frame #8 {
                n713 = Concatenate Strings("start ", "\r") -> (w1162:string)
                n714 = VISA Write(VISA resource name=w1166, write buffer=w1162, error in (no error)=w1163) -> (VISA resource name out=w1165:refnum<visa-resource-name>, error out=w1164:errorcluster)  [unwired: 1 out]
              }
              frame #9 {
                n715 = Wait (ms)(milliseconds to wait=w1169) -> ()  [unwired: 1 out]
              }
              frame #10 {
                n716 = local write "Flush Pump 1"(FALSE ("Flush Pump 1")) -> ()
                n717 = Concatenate Strings("enter main ", "\r") -> (w1177:string)
                n718 = VISA Write(VISA resource name=w1173, write buffer=w1177, error in (no error)=w1172) -> (VISA resource name out=w1176:refnum<visa-resource-name>, error out=w1175:errorcluster)  [unwired: 1 out]
                n719 = VISA Close(VISA resource name=w1176, error in (no error)=w1175) -> ()  [unwired: 1 out]
              }
            }
            n720 = Concatenate Strings("set units 4 ", w1099) -> (w1105:string)
            n721 = Multiply(x="Flush\nRate (ul/min)", y=60) -> (x*y=w1103:dbl)
            n722 = Number To Decimal String(number=w1103) -> (decimal integer string=w1106:string)  [unwired: 1 in]
            n723 = Concatenate Strings("set rate ", w1106, w1099) -> (w1108:string)
            n724 = Number To Decimal String(number="Flush\nVolume (ul)") -> (decimal integer string=w1110:string)  [unwired: 1 in]
            n725 = Concatenate Strings("set volume ", w1110, w1099) -> (w1111:string)
          }
          event "Flush Pump 2": Value Change {
            w1185 = "\r"
            n726 = event-data() -> ()  [unwired: 1 in, 5 out]
            n727 = call-poly "VISA Configure Serial Port"("VISA resource name"=w1194) -> ("VISA resource name out"=w1205:refnum<visa-resource-name>, "error out"=w1206:errorcluster)  [unwired: 13 in]
            n728 = local read "Write Wait"() -> (w1180:i32)
            n729 = Concatenate Strings("enter pump2", w1185) -> (w1186:string)
            n730 = flat-sequence {
              tunnel: w1206 -> [w1221]
              tunnel: w1205 -> [w1223]
              tunnel: [w1222] -> w1191
              tunnel: [w1220] -> w1189
              tunnel: w1186 -> [w1219]
              tunnel: w1191 -> [w1226]
              tunnel: [w1226] -> w1190
              tunnel: w1189 -> [w1225]
              tunnel: [w1225] -> w1188
              tunnel: w1180 -> [w1224]
              tunnel: [w1231] -> w1218
              tunnel: w1198 -> [w1230]
              tunnel: [w1227] -> w1217
              tunnel: w1190 -> [w1229]
              tunnel: w1188 -> [w1228]
              tunnel: w1218 -> [w1234]
              tunnel: [w1234] -> w1216
              tunnel: [w1233] -> w1215
              tunnel: w1217 -> [w1233]
              tunnel: w1180 -> [w1232]
              tunnel: w1216 -> [w1239]
              tunnel: [w1238] -> w1214
              tunnel: w1201 -> [w1237]
              tunnel: w1215 -> [w1236]
              tunnel: [w1235] -> w1213
              tunnel: w1214 -> [w1242]
              tunnel: [w1242] -> w1212
              tunnel: [w1241] -> w1211
              tunnel: w1213 -> [w1241]
              tunnel: w1180 -> [w1240]
              tunnel: w1212 -> [w1247]
              tunnel: [w1246] -> w1210
              tunnel: w1204 -> [w1245]
              tunnel: w1211 -> [w1244]
              tunnel: [w1243] -> w1209
              tunnel: [w1250] -> w1208
              tunnel: w1210 -> [w1250]
              tunnel: [w1249] -> w1207
              tunnel: w1209 -> [w1249]
              tunnel: w1180 -> [w1248]
              tunnel: w1208 -> [w1257]
              tunnel: w1207 -> [w1256]
              tunnel: [w1252] -> w1184
              tunnel: [w1251] -> w1182
              tunnel: w1184 -> [w1260]
              tunnel: [w1260] -> w1183
              tunnel: w1182 -> [w1259]
              tunnel: [w1259] -> w1181
              tunnel: w1180 -> [w1258]
              tunnel: w1183 -> [w1264]
              tunnel: w1181 -> [w1263]
              frame #0 {
                n731 = VISA Write(VISA resource name=w1223, write buffer=w1219, error in (no error)=w1221) -> (VISA resource name out=w1222:refnum<visa-resource-name>, error out=w1220:errorcluster)  [unwired: 1 out]
              }
              frame #1 {
                n732 = Wait (ms)(milliseconds to wait=w1224) -> ()  [unwired: 1 out]
              }
              frame #2 {
                n733 = VISA Write(VISA resource name=w1229, write buffer=w1230, error in (no error)=w1228) -> (VISA resource name out=w1231:refnum<visa-resource-name>, error out=w1227:errorcluster)  [unwired: 1 out]
              }
              frame #3 {
                n734 = Wait (ms)(milliseconds to wait=w1232) -> ()  [unwired: 1 out]
              }
              frame #4 {
                n735 = VISA Write(VISA resource name=w1239, write buffer=w1237, error in (no error)=w1236) -> (VISA resource name out=w1238:refnum<visa-resource-name>, error out=w1235:errorcluster)  [unwired: 1 out]
              }
              frame #5 {
                n736 = Wait (ms)(milliseconds to wait=w1240) -> ()  [unwired: 1 out]
              }
              frame #6 {
                n737 = VISA Write(VISA resource name=w1247, write buffer=w1245, error in (no error)=w1244) -> (VISA resource name out=w1246:refnum<visa-resource-name>, error out=w1243:errorcluster)  [unwired: 1 out]
              }
              frame #7 {
                n738 = Wait (ms)(milliseconds to wait=w1248) -> ()  [unwired: 1 out]
              }
              frame #8 {
                n739 = Concatenate Strings("start ", "\r") -> (w1255:string)
                n740 = VISA Write(VISA resource name=w1257, write buffer=w1255, error in (no error)=w1256) -> (VISA resource name out=w1252:refnum<visa-resource-name>, error out=w1251:errorcluster)  [unwired: 1 out]
              }
              frame #9 {
                n741 = Wait (ms)(milliseconds to wait=w1258) -> ()  [unwired: 1 out]
              }
              frame #10 {
                n742 = local write "Flush Pump 2"(FALSE ("Flush Pump 1")) -> ()
                n743 = Concatenate Strings("enter main ", "\r") -> (w1265:string)
                n744 = VISA Write(VISA resource name=w1264, write buffer=w1265, error in (no error)=w1263) -> (VISA resource name out=w1262:refnum<visa-resource-name>, error out=w1261:errorcluster)  [unwired: 1 out]
                n745 = VISA Close(VISA resource name=w1262, error in (no error)=w1261) -> ()  [unwired: 1 out]
              }
            }
            n746 = Concatenate Strings("set units 4 ", w1185) -> (w1198:string)
            n747 = Multiply(x="Flush \nRate (ul/min)  2", y=60) -> (x*y=w1196:dbl)
            n748 = Number To Decimal String(number=w1196) -> (decimal integer string=w1199:string)  [unwired: 1 in]
            n749 = Concatenate Strings("set rate ", w1199, w1185) -> (w1201:string)
            n750 = Number To Decimal String(number="Flush\nVolume (ul)  2") -> (decimal integer string=w1203:string)  [unwired: 1 in]
            n751 = Concatenate Strings("set volume ", w1203, w1185) -> (w1204:string)
          }
          event "Stop": Value Change {
            n752 = event-data() -> ()  [unwired: 1 in, 5 out]
            n753 = local read "Stop"() -> (w1269:bool)
          }
          event "Inject Pump 2": Value Change {
            n754 = event-data() -> ()  [unwired: 1 in, 5 out]
            n755 = case shown="True" "Inject Pump 2" {
              tunnel: w1270 -> [w1273 w1315]
              frame False {
                n756 = local read "Write Wait"() -> (w1272:i32)
                n757 = call-poly "VISA Configure Serial Port"("VISA resource name"=w1273) -> ("VISA resource name out"=w1277:refnum<visa-resource-name>, "error out"=w1278:errorcluster)  [unwired: 13 in]
                n758 = Concatenate Strings("enter pump2", "\r") -> (w1275:string)
                n759 = flat-sequence {
                  tunnel: w1278 -> [w1289]
                  tunnel: w1277 -> [w1291]
                  tunnel: [w1290] -> w1286
                  tunnel: [w1288] -> w1285
                  tunnel: w1275 -> [w1287]
                  tunnel: w1286 -> [w1294]
                  tunnel: w1285 -> [w1293]
                  tunnel: [w1294] -> w1284
                  tunnel: [w1293] -> w1283
                  tunnel: w1272 -> [w1292]
                  tunnel: [w1298] -> w1282
                  tunnel: [w1297] -> w1281
                  tunnel: w1284 -> [w1296]
                  tunnel: w1283 -> [w1295]
                  tunnel: w1282 -> [w1304]
                  tunnel: [w1304] -> w1280
                  tunnel: w1281 -> [w1303]
                  tunnel: [w1303] -> w1279
                  tunnel: w1272 -> [w1302]
                  tunnel: w1280 -> [w1308]
                  tunnel: w1279 -> [w1307]
                  frame #0 {
                    n760 = VISA Write(VISA resource name=w1291, write buffer=w1287, error in (no error)=w1289) -> (VISA resource name out=w1290:refnum<visa-resource-name>, error out=w1288:errorcluster)  [unwired: 1 out]
                  }
                  frame #1 {
                    n761 = Wait (ms)(milliseconds to wait=w1292) -> ()  [unwired: 1 out]
                  }
                  frame #2 {
                    n762 = Concatenate Strings("stop ", "\r") -> (w1301:string)
                    n763 = VISA Write(VISA resource name=w1296, write buffer=w1301, error in (no error)=w1295) -> (VISA resource name out=w1298:refnum<visa-resource-name>, error out=w1297:errorcluster)  [unwired: 1 out]
                  }
                  frame #3 {
                    n764 = Wait (ms)(milliseconds to wait=w1302) -> ()  [unwired: 1 out]
                  }
                  frame #4 {
                    n765 = Concatenate Strings("enter main ", "\r") -> (w1309:string)
                    n766 = VISA Write(VISA resource name=w1308, write buffer=w1309, error in (no error)=w1307) -> (VISA resource name out=w1306:refnum<visa-resource-name>, error out=w1305:errorcluster)  [unwired: 1 out]
                    n767 = VISA Close(VISA resource name=w1306, error in (no error)=w1305) -> ()  [unwired: 1 out]
                  }
                }
              }
              frame True {
                w1328 = "\r"
                n768 = call-poly "VISA Configure Serial Port"("VISA resource name"=w1315) -> ("VISA resource name out"=w1317:refnum<visa-resource-name>, "error out"=w1316:errorcluster)  [unwired: 13 in]
                n769 = local read "Write Wait"() -> (w1312:i32)
                n770 = Concatenate Strings("enter pump2", w1328) -> (w1327:string)
                n771 = flat-sequence {
                  tunnel: w1316 -> [w1351]
                  tunnel: w1317 -> [w1353]
                  tunnel: [w1352] -> w1348
                  tunnel: [w1350] -> w1347
                  tunnel: w1327 -> [w1349]
                  tunnel: w1348 -> [w1356]
                  tunnel: [w1356] -> w1346
                  tunnel: w1347 -> [w1355]
                  tunnel: [w1355] -> w1345
                  tunnel: w1312 -> [w1354]
                  tunnel: [w1361] -> w1344
                  tunnel: w1324 -> [w1360]
                  tunnel: [w1357] -> w1343
                  tunnel: w1346 -> [w1359]
                  tunnel: w1345 -> [w1358]
                  tunnel: w1344 -> [w1364]
                  tunnel: [w1364] -> w1342
                  tunnel: [w1363] -> w1341
                  tunnel: w1343 -> [w1363]
                  tunnel: w1312 -> [w1362]
                  tunnel: w1342 -> [w1369]
                  tunnel: [w1368] -> w1340
                  tunnel: w1321 -> [w1367]
                  tunnel: w1341 -> [w1366]
                  tunnel: [w1365] -> w1339
                  tunnel: w1340 -> [w1372]
                  tunnel: [w1372] -> w1338
                  tunnel: [w1371] -> w1337
                  tunnel: w1339 -> [w1371]
                  tunnel: w1312 -> [w1370]
                  tunnel: w1338 -> [w1377]
                  tunnel: [w1376] -> w1336
                  tunnel: w1318 -> [w1375]
                  tunnel: w1337 -> [w1374]
                  tunnel: [w1373] -> w1335
                  tunnel: [w1380] -> w1334
                  tunnel: w1336 -> [w1380]
                  tunnel: [w1379] -> w1333
                  tunnel: w1335 -> [w1379]
                  tunnel: w1312 -> [w1378]
                  tunnel: w1334 -> [w1387]
                  tunnel: w1333 -> [w1386]
                  tunnel: [w1382] -> w1332
                  tunnel: [w1381] -> w1331
                  tunnel: w1332 -> [w1390]
                  tunnel: [w1390] -> w1330
                  tunnel: w1331 -> [w1389]
                  tunnel: [w1389] -> w1329
                  tunnel: w1312 -> [w1388]
                  tunnel: w1330 -> [w1394]
                  tunnel: w1329 -> [w1393]
                  frame #0 {
                    n772 = VISA Write(VISA resource name=w1353, write buffer=w1349, error in (no error)=w1351) -> (VISA resource name out=w1352:refnum<visa-resource-name>, error out=w1350:errorcluster)  [unwired: 1 out]
                  }
                  frame #1 {
                    n773 = Wait (ms)(milliseconds to wait=w1354) -> ()  [unwired: 1 out]
                  }
                  frame #2 {
                    n774 = VISA Write(VISA resource name=w1359, write buffer=w1360, error in (no error)=w1358) -> (VISA resource name out=w1361:refnum<visa-resource-name>, error out=w1357:errorcluster)  [unwired: 1 out]
                  }
                  frame #3 {
                    n775 = Wait (ms)(milliseconds to wait=w1362) -> ()  [unwired: 1 out]
                  }
                  frame #4 {
                    n776 = VISA Write(VISA resource name=w1369, write buffer=w1367, error in (no error)=w1366) -> (VISA resource name out=w1368:refnum<visa-resource-name>, error out=w1365:errorcluster)  [unwired: 1 out]
                  }
                  frame #5 {
                    n777 = Wait (ms)(milliseconds to wait=w1370) -> ()  [unwired: 1 out]
                  }
                  frame #6 {
                    n778 = VISA Write(VISA resource name=w1377, write buffer=w1375, error in (no error)=w1374) -> (VISA resource name out=w1376:refnum<visa-resource-name>, error out=w1373:errorcluster)  [unwired: 1 out]
                  }
                  frame #7 {
                    n779 = Wait (ms)(milliseconds to wait=w1378) -> ()  [unwired: 1 out]
                  }
                  frame #8 {
                    n780 = Concatenate Strings("start ", "\r") -> (w1385:string)
                    n781 = VISA Write(VISA resource name=w1387, write buffer=w1385, error in (no error)=w1386) -> (VISA resource name out=w1382:refnum<visa-resource-name>, error out=w1381:errorcluster)  [unwired: 1 out]
                  }
                  frame #9 {
                    n782 = Wait (ms)(milliseconds to wait=w1388) -> ()  [unwired: 1 out]
                  }
                  frame #10 {
                    n783 = Concatenate Strings("enter main ", "\r") -> (w1395:string)
                    n784 = VISA Write(VISA resource name=w1394, write buffer=w1395, error in (no error)=w1393) -> (VISA resource name out=w1392:refnum<visa-resource-name>, error out=w1391:errorcluster)  [unwired: 1 out]
                    n785 = VISA Close(VISA resource name=w1392, error in (no error)=w1391) -> ()  [unwired: 1 out]
                  }
                }
                n786 = local read "Normal \nRate (ul/hr)  2"() -> (w1313:dbl)
                n787 = Concatenate Strings("set units 4 ", w1328) -> (w1324:string)
                n788 = local read "Normal \nVolume (ul) 2"() -> (w1314:dbl)
                n789 = Number To Decimal String(number=w1313) -> (decimal integer string=w1323:string)  [unwired: 1 in]
                n790 = Concatenate Strings("set rate ", w1323, w1328) -> (w1321:string)
                n791 = Number To Decimal String(number=w1314) -> (decimal integer string=w1319:string)  [unwired: 1 in]
                n792 = Concatenate Strings("set volume ", w1319, w1328) -> (w1318:string)
              }
            }
          }
          event "Inject Pump 1": Value Change {
            n793 = event-data() -> ()  [unwired: 1 in, 5 out]
            n794 = case shown="True" "Inject Pump 1" {
              tunnel: w1398 -> [w1401 w1443]
              frame False {
                n795 = local read "Write Wait"() -> (w1400:i32)
                n796 = call-poly "VISA Configure Serial Port"("VISA resource name"=w1401) -> ("VISA resource name out"=w1405:refnum<visa-resource-name>, "error out"=w1406:errorcluster)  [unwired: 13 in]
                n797 = Concatenate Strings("enter pump1", "\r") -> (w1403:string)
                n798 = flat-sequence {
                  tunnel: w1406 -> [w1417]
                  tunnel: w1405 -> [w1419]
                  tunnel: [w1418] -> w1414
                  tunnel: [w1416] -> w1413
                  tunnel: w1403 -> [w1415]
                  tunnel: w1414 -> [w1422]
                  tunnel: w1413 -> [w1421]
                  tunnel: [w1422] -> w1412
                  tunnel: [w1421] -> w1411
                  tunnel: w1400 -> [w1420]
                  tunnel: [w1426] -> w1410
                  tunnel: [w1425] -> w1409
                  tunnel: w1412 -> [w1424]
                  tunnel: w1411 -> [w1423]
                  tunnel: w1410 -> [w1432]
                  tunnel: [w1432] -> w1408
                  tunnel: w1409 -> [w1431]
                  tunnel: [w1431] -> w1407
                  tunnel: w1400 -> [w1430]
                  tunnel: w1408 -> [w1436]
                  tunnel: w1407 -> [w1435]
                  frame #0 {
                    n799 = VISA Write(VISA resource name=w1419, write buffer=w1415, error in (no error)=w1417) -> (VISA resource name out=w1418:refnum<visa-resource-name>, error out=w1416:errorcluster)  [unwired: 1 out]
                  }
                  frame #1 {
                    n800 = Wait (ms)(milliseconds to wait=w1420) -> ()  [unwired: 1 out]
                  }
                  frame #2 {
                    n801 = Concatenate Strings("stop ", "\r") -> (w1429:string)
                    n802 = VISA Write(VISA resource name=w1424, write buffer=w1429, error in (no error)=w1423) -> (VISA resource name out=w1426:refnum<visa-resource-name>, error out=w1425:errorcluster)  [unwired: 1 out]
                  }
                  frame #3 {
                    n803 = Wait (ms)(milliseconds to wait=w1430) -> ()  [unwired: 1 out]
                  }
                  frame #4 {
                    n804 = Concatenate Strings("enter main ", "\r") -> (w1437:string)
                    n805 = VISA Write(VISA resource name=w1436, write buffer=w1437, error in (no error)=w1435) -> (VISA resource name out=w1434:refnum<visa-resource-name>, error out=w1433:errorcluster)  [unwired: 1 out]
                    n806 = VISA Close(VISA resource name=w1434, error in (no error)=w1433) -> ()  [unwired: 1 out]
                  }
                }
              }
              frame True {
                w1456 = "\r"
                n807 = call-poly "VISA Configure Serial Port"("VISA resource name"=w1443) -> ("VISA resource name out"=w1445:refnum<visa-resource-name>, "error out"=w1444:errorcluster)  [unwired: 13 in]
                n808 = local read "Write Wait"() -> (w1440:i32)
                n809 = flat-sequence {
                  tunnel: w1444 -> [w1479]
                  tunnel: w1445 -> [w1481]
                  tunnel: [w1480] -> w1476
                  tunnel: [w1478] -> w1475
                  tunnel: w1455 -> [w1477]
                  tunnel: w1476 -> [w1484]
                  tunnel: [w1484] -> w1474
                  tunnel: w1475 -> [w1483]
                  tunnel: [w1483] -> w1473
                  tunnel: w1440 -> [w1482]
                  tunnel: [w1489] -> w1472
                  tunnel: w1452 -> [w1488]
                  tunnel: [w1485] -> w1471
                  tunnel: w1474 -> [w1487]
                  tunnel: w1473 -> [w1486]
                  tunnel: w1472 -> [w1492]
                  tunnel: [w1492] -> w1470
                  tunnel: [w1491] -> w1469
                  tunnel: w1471 -> [w1491]
                  tunnel: w1440 -> [w1490]
                  tunnel: w1470 -> [w1497]
                  tunnel: [w1496] -> w1468
                  tunnel: w1449 -> [w1495]
                  tunnel: w1469 -> [w1494]
                  tunnel: [w1493] -> w1467
                  tunnel: w1468 -> [w1500]
                  tunnel: [w1500] -> w1466
                  tunnel: [w1499] -> w1465
                  tunnel: w1467 -> [w1499]
                  tunnel: w1440 -> [w1498]
                  tunnel: w1466 -> [w1505]
                  tunnel: [w1504] -> w1464
                  tunnel: w1446 -> [w1503]
                  tunnel: w1465 -> [w1502]
                  tunnel: [w1501] -> w1463
                  tunnel: [w1508] -> w1462
                  tunnel: w1464 -> [w1508]
                  tunnel: [w1507] -> w1461
                  tunnel: w1463 -> [w1507]
                  tunnel: w1440 -> [w1506]
                  tunnel: w1462 -> [w1515]
                  tunnel: w1461 -> [w1514]
                  tunnel: [w1510] -> w1460
                  tunnel: [w1509] -> w1459
                  tunnel: w1460 -> [w1518]
                  tunnel: [w1518] -> w1458
                  tunnel: w1459 -> [w1517]
                  tunnel: [w1517] -> w1457
                  tunnel: w1440 -> [w1516]
                  tunnel: w1458 -> [w1522]
                  tunnel: w1457 -> [w1521]
                  frame #0 {
                    n810 = VISA Write(VISA resource name=w1481, write buffer=w1477, error in (no error)=w1479) -> (VISA resource name out=w1480:refnum<visa-resource-name>, error out=w1478:errorcluster)  [unwired: 1 out]
                  }
                  frame #1 {
                    n811 = Wait (ms)(milliseconds to wait=w1482) -> ()  [unwired: 1 out]
                  }
                  frame #2 {
                    n812 = VISA Write(VISA resource name=w1487, write buffer=w1488, error in (no error)=w1486) -> (VISA resource name out=w1489:refnum<visa-resource-name>, error out=w1485:errorcluster)  [unwired: 1 out]
                  }
                  frame #3 {
                    n813 = Wait (ms)(milliseconds to wait=w1490) -> ()  [unwired: 1 out]
                  }
                  frame #4 {
                    n814 = VISA Write(VISA resource name=w1497, write buffer=w1495, error in (no error)=w1494) -> (VISA resource name out=w1496:refnum<visa-resource-name>, error out=w1493:errorcluster)  [unwired: 1 out]
                  }
                  frame #5 {
                    n815 = Wait (ms)(milliseconds to wait=w1498) -> ()  [unwired: 1 out]
                  }
                  frame #6 {
                    n816 = VISA Write(VISA resource name=w1505, write buffer=w1503, error in (no error)=w1502) -> (VISA resource name out=w1504:refnum<visa-resource-name>, error out=w1501:errorcluster)  [unwired: 1 out]
                  }
                  frame #7 {
                    n817 = Wait (ms)(milliseconds to wait=w1506) -> ()  [unwired: 1 out]
                  }
                  frame #8 {
                    n818 = Concatenate Strings("start ", "\r") -> (w1513:string)
                    n819 = VISA Write(VISA resource name=w1515, write buffer=w1513, error in (no error)=w1514) -> (VISA resource name out=w1510:refnum<visa-resource-name>, error out=w1509:errorcluster)  [unwired: 1 out]
                  }
                  frame #9 {
                    n820 = Wait (ms)(milliseconds to wait=w1516) -> ()  [unwired: 1 out]
                  }
                  frame #10 {
                    n821 = Concatenate Strings("enter main ", "\r") -> (w1523:string)
                    n822 = VISA Write(VISA resource name=w1522, write buffer=w1523, error in (no error)=w1521) -> (VISA resource name out=w1520:refnum<visa-resource-name>, error out=w1519:errorcluster)  [unwired: 1 out]
                    n823 = VISA Close(VISA resource name=w1520, error in (no error)=w1519) -> ()  [unwired: 1 out]
                  }
                }
                n824 = Concatenate Strings("enter pump1", w1456) -> (w1455:string)
                n825 = local read "Normal \nRate (ul/hr)"() -> (w1441:dbl)
                n826 = Concatenate Strings("set units 4 ", w1456) -> (w1452:string)
                n827 = local read "Normal \nVolume (ul)"() -> (w1442:dbl)
                n828 = Number To Decimal String(number=w1441) -> (decimal integer string=w1451:string)  [unwired: 1 in]
                n829 = Concatenate Strings("set rate ", w1451, w1456) -> (w1449:string)
                n830 = Number To Decimal String(number=w1442) -> (decimal integer string=w1447:string)  [unwired: 1 in]
                n831 = Concatenate Strings("set volume ", w1447, w1456) -> (w1446:string)
              }
            }
          }
          event "Normal \nVolume (ul)": Value Change {
            n832 = event-data() -> ()  [unwired: 1 in, 5 out]
            n833 = call-poly "VISA Configure Serial Port"("VISA resource name"=w1541) -> ("VISA resource name out"=w1543:refnum<visa-resource-name>, "error out"=w1542:errorcluster)  [unwired: 13 in]
            n834 = local read "Write Wait"() -> (w1526:i32)
            n835 = Concatenate Strings("enter pump1", "\r") -> (w1545:string)
            n836 = flat-sequence {
              tunnel: w1542 -> [w1555]
              tunnel: w1543 -> [w1557]
              tunnel: [w1556] -> w1535
              tunnel: [w1554] -> w1534
              tunnel: w1545 -> [w1553]
              tunnel: w1535 -> [w1560]
              tunnel: [w1560] -> w1533
              tunnel: w1534 -> [w1559]
              tunnel: [w1559] -> w1531
              tunnel: w1526 -> [w1558]
              tunnel: w1533 -> [w1564]
              tunnel: [w1565] -> w1532
              tunnel: w1531 -> [w1563]
              tunnel: [w1562] -> w1530
              tunnel: w1527 -> [w1561]
              tunnel: w1532 -> [w1568]
              tunnel: w1530 -> [w1567]
              tunnel: [w1568] -> w1552
              tunnel: [w1567] -> w1551
              tunnel: w1526 -> [w1566]
              tunnel: [w1573] -> w1550
              tunnel: [w1572] -> w1549
              tunnel: w1552 -> [w1571]
              tunnel: w1551 -> [w1570]
              tunnel: w1536 -> [w1569]
              tunnel: w1550 -> [w1576]
              tunnel: [w1576] -> w1548
              tunnel: w1549 -> [w1575]
              tunnel: [w1575] -> w1547
              tunnel: w1526 -> [w1574]
              tunnel: w1548 -> [w1580]
              tunnel: w1547 -> [w1579]
              frame #0 {
                n837 = VISA Write(VISA resource name=w1557, write buffer=w1553, error in (no error)=w1555) -> (VISA resource name out=w1556:refnum<visa-resource-name>, error out=w1554:errorcluster)  [unwired: 1 out]
              }
              frame #1 {
                n838 = Wait (ms)(milliseconds to wait=w1558) -> ()  [unwired: 1 out]
              }
              frame #2 {
                n839 = VISA Write(VISA resource name=w1564, write buffer=w1561, error in (no error)=w1563) -> (VISA resource name out=w1565:refnum<visa-resource-name>, error out=w1562:errorcluster)  [unwired: 1 out]
              }
              frame #3 {
                n840 = Wait (ms)(milliseconds to wait=w1566) -> ()  [unwired: 1 out]
              }
              frame #4 {
                n841 = VISA Write(VISA resource name=w1571, write buffer=w1569, error in (no error)=w1570) -> (VISA resource name out=w1573:refnum<visa-resource-name>, error out=w1572:errorcluster)  [unwired: 1 out]
              }
              frame #5 {
                n842 = Wait (ms)(milliseconds to wait=w1574) -> ()  [unwired: 1 out]
              }
              frame #6 {
                n843 = Concatenate Strings("enter main ", "\r") -> (w1581:string)
                n844 = VISA Write(VISA resource name=w1580, write buffer=w1581, error in (no error)=w1579) -> (VISA resource name out=w1578:refnum<visa-resource-name>, error out=w1577:errorcluster)  [unwired: 1 out]
                n845 = VISA Close(VISA resource name=w1578, error in (no error)=w1577) -> ()  [unwired: 1 out]
              }
            }
            n846 = Concatenate Strings("set units 4", "\r") -> (w1527:string)
            n847 = Number To Decimal String(number="Normal \nVolume (ul)") -> (decimal integer string=w1538:string)  [unwired: 1 in]
            n848 = Concatenate Strings("set volume", w1538, "\r") -> (w1536:string)
          }
          event "Normal \nRate (ul/hr)": Value Change {
            n849 = event-data() -> ()  [unwired: 1 in, 5 out]
            n850 = call-poly "VISA Configure Serial Port"("VISA resource name"=w1586) -> ("VISA resource name out"=w1594:refnum<visa-resource-name>, "error out"=w1593:errorcluster)  [unwired: 13 in]
            n851 = local read "Write Wait"() -> (w1584:i32)
            n852 = Concatenate Strings("enter pump1", "\r") -> (w1596:string)
            n853 = flat-sequence {
              tunnel: w1593 -> [w1613]
              tunnel: w1594 -> [w1615]
              tunnel: [w1614] -> w1609
              tunnel: [w1612] -> w1608
              tunnel: w1596 -> [w1611]
              tunnel: w1609 -> [w1618]
              tunnel: [w1618] -> w1607
              tunnel: w1608 -> [w1617]
              tunnel: [w1617] -> w1606
              tunnel: w1584 -> [w1616]
              tunnel: w1607 -> [w1622]
              tunnel: [w1623] -> w1605
              tunnel: w1606 -> [w1621]
              tunnel: [w1620] -> w1604
              tunnel: w1587 -> [w1619]
              tunnel: w1605 -> [w1626]
              tunnel: w1604 -> [w1625]
              tunnel: [w1626] -> w1603
              tunnel: [w1625] -> w1602
              tunnel: w1584 -> [w1624]
              tunnel: [w1631] -> w1601
              tunnel: [w1630] -> w1600
              tunnel: w1603 -> [w1629]
              tunnel: w1602 -> [w1628]
              tunnel: w1590 -> [w1627]
              tunnel: w1601 -> [w1634]
              tunnel: [w1634] -> w1599
              tunnel: w1600 -> [w1633]
              tunnel: [w1633] -> w1598
              tunnel: w1584 -> [w1632]
              tunnel: w1599 -> [w1638]
              tunnel: w1598 -> [w1637]
              frame #0 {
                n854 = VISA Write(VISA resource name=w1615, write buffer=w1611, error in (no error)=w1613) -> (VISA resource name out=w1614:refnum<visa-resource-name>, error out=w1612:errorcluster)  [unwired: 1 out]
              }
              frame #1 {
                n855 = Wait (ms)(milliseconds to wait=w1616) -> ()  [unwired: 1 out]
              }
              frame #2 {
                n856 = VISA Write(VISA resource name=w1622, write buffer=w1619, error in (no error)=w1621) -> (VISA resource name out=w1623:refnum<visa-resource-name>, error out=w1620:errorcluster)  [unwired: 1 out]
              }
              frame #3 {
                n857 = Wait (ms)(milliseconds to wait=w1624) -> ()  [unwired: 1 out]
              }
              frame #4 {
                n858 = VISA Write(VISA resource name=w1629, write buffer=w1627, error in (no error)=w1628) -> (VISA resource name out=w1631:refnum<visa-resource-name>, error out=w1630:errorcluster)  [unwired: 1 out]
              }
              frame #5 {
                n859 = Wait (ms)(milliseconds to wait=w1632) -> ()  [unwired: 1 out]
              }
              frame #6 {
                n860 = Concatenate Strings("enter main ", "\r") -> (w1639:string)
                n861 = VISA Write(VISA resource name=w1638, write buffer=w1639, error in (no error)=w1637) -> (VISA resource name out=w1636:refnum<visa-resource-name>, error out=w1635:errorcluster)  [unwired: 1 out]
                n862 = VISA Close(VISA resource name=w1636, error in (no error)=w1635) -> ()  [unwired: 1 out]
              }
            }
            n863 = Concatenate Strings("set units 4", "\r") -> (w1587:string)
            n864 = Number To Decimal String(number="Normal \nRate (ul/hr)") -> (decimal integer string=w1585:string)  [unwired: 1 in]
            n865 = Concatenate Strings("set rate", w1585, "\r") -> (w1590:string)
          }
          event "Normal \nRate (ul/hr)  2": Value Change {
            n866 = event-data() -> ()  [unwired: 1 in, 5 out]
            n867 = call-poly "VISA Configure Serial Port"("VISA resource name"=w1644) -> ("VISA resource name out"=w1652:refnum<visa-resource-name>, "error out"=w1651:errorcluster)  [unwired: 13 in]
            n868 = local read "Write Wait"() -> (w1642:i32)
            n869 = Concatenate Strings("enter pump2", "\r") -> (w1654:string)
            n870 = flat-sequence {
              tunnel: w1651 -> [w1671]
              tunnel: w1652 -> [w1673]
              tunnel: [w1672] -> w1667
              tunnel: [w1670] -> w1666
              tunnel: w1654 -> [w1669]
              tunnel: w1667 -> [w1676]
              tunnel: [w1676] -> w1665
              tunnel: w1666 -> [w1675]
              tunnel: [w1675] -> w1664
              tunnel: w1642 -> [w1674]
              tunnel: w1665 -> [w1680]
              tunnel: [w1681] -> w1663
              tunnel: w1664 -> [w1679]
              tunnel: [w1678] -> w1662
              tunnel: w1645 -> [w1677]
              tunnel: w1663 -> [w1684]
              tunnel: w1662 -> [w1683]
              tunnel: [w1684] -> w1661
              tunnel: [w1683] -> w1660
              tunnel: w1642 -> [w1682]
              tunnel: [w1689] -> w1659
              tunnel: [w1688] -> w1658
              tunnel: w1661 -> [w1687]
              tunnel: w1660 -> [w1686]
              tunnel: w1648 -> [w1685]
              tunnel: w1659 -> [w1692]
              tunnel: [w1692] -> w1657
              tunnel: w1658 -> [w1691]
              tunnel: [w1691] -> w1656
              tunnel: w1642 -> [w1690]
              tunnel: w1657 -> [w1696]
              tunnel: w1656 -> [w1695]
              frame #0 {
                n871 = VISA Write(VISA resource name=w1673, write buffer=w1669, error in (no error)=w1671) -> (VISA resource name out=w1672:refnum<visa-resource-name>, error out=w1670:errorcluster)  [unwired: 1 out]
              }
              frame #1 {
                n872 = Wait (ms)(milliseconds to wait=w1674) -> ()  [unwired: 1 out]
              }
              frame #2 {
                n873 = VISA Write(VISA resource name=w1680, write buffer=w1677, error in (no error)=w1679) -> (VISA resource name out=w1681:refnum<visa-resource-name>, error out=w1678:errorcluster)  [unwired: 1 out]
              }
              frame #3 {
                n874 = Wait (ms)(milliseconds to wait=w1682) -> ()  [unwired: 1 out]
              }
              frame #4 {
                n875 = VISA Write(VISA resource name=w1687, write buffer=w1685, error in (no error)=w1686) -> (VISA resource name out=w1689:refnum<visa-resource-name>, error out=w1688:errorcluster)  [unwired: 1 out]
              }
              frame #5 {
                n876 = Wait (ms)(milliseconds to wait=w1690) -> ()  [unwired: 1 out]
              }
              frame #6 {
                n877 = Concatenate Strings("enter main ", "\r") -> (w1697:string)
                n878 = VISA Write(VISA resource name=w1696, write buffer=w1697, error in (no error)=w1695) -> (VISA resource name out=w1694:refnum<visa-resource-name>, error out=w1693:errorcluster)  [unwired: 1 out]
                n879 = VISA Close(VISA resource name=w1694, error in (no error)=w1693) -> ()  [unwired: 1 out]
              }
            }
            n880 = Concatenate Strings("set units 4", "\r") -> (w1645:string)
            n881 = Number To Decimal String(number="Normal \nRate (ul/hr)  2") -> (decimal integer string=w1643:string)  [unwired: 1 in]
            n882 = Concatenate Strings("set rate", w1643, "\r") -> (w1648:string)
          }
          event "Normal \nVolume (ul) 2": Value Change {
            n883 = event-data() -> ()  [unwired: 1 in, 5 out]
            n884 = call-poly "VISA Configure Serial Port"("VISA resource name"=w1703) -> ("VISA resource name out"=w1707:refnum<visa-resource-name>, "error out"=w1708:errorcluster)  [unwired: 13 in]
            n885 = local read "Write Wait"() -> (w1700:i32)
            n886 = Concatenate Strings("enter pump2", "\r") -> (w1705:string)
            n887 = flat-sequence {
              tunnel: w1708 -> [w1729]
              tunnel: w1707 -> [w1731]
              tunnel: [w1730] -> w1726
              tunnel: [w1728] -> w1725
              tunnel: w1705 -> [w1727]
              tunnel: w1726 -> [w1734]
              tunnel: [w1734] -> w1724
              tunnel: w1725 -> [w1733]
              tunnel: [w1733] -> w1723
              tunnel: w1700 -> [w1732]
              tunnel: w1724 -> [w1738]
              tunnel: [w1739] -> w1722
              tunnel: w1723 -> [w1737]
              tunnel: [w1736] -> w1721
              tunnel: w1714 -> [w1735]
              tunnel: w1722 -> [w1742]
              tunnel: w1721 -> [w1741]
              tunnel: [w1742] -> w1720
              tunnel: [w1741] -> w1719
              tunnel: w1700 -> [w1740]
              tunnel: [w1747] -> w1718
              tunnel: [w1746] -> w1717
              tunnel: w1720 -> [w1745]
              tunnel: w1719 -> [w1744]
              tunnel: w1711 -> [w1743]
              tunnel: w1718 -> [w1750]
              tunnel: [w1750] -> w1716
              tunnel: w1717 -> [w1749]
              tunnel: [w1749] -> w1715
              tunnel: w1700 -> [w1748]
              tunnel: w1716 -> [w1754]
              tunnel: w1715 -> [w1753]
              frame #0 {
                n888 = VISA Write(VISA resource name=w1731, write buffer=w1727, error in (no error)=w1729) -> (VISA resource name out=w1730:refnum<visa-resource-name>, error out=w1728:errorcluster)  [unwired: 1 out]
              }
              frame #1 {
                n889 = Wait (ms)(milliseconds to wait=w1732) -> ()  [unwired: 1 out]
              }
              frame #2 {
                n890 = VISA Write(VISA resource name=w1738, write buffer=w1735, error in (no error)=w1737) -> (VISA resource name out=w1739:refnum<visa-resource-name>, error out=w1736:errorcluster)  [unwired: 1 out]
              }
              frame #3 {
                n891 = Wait (ms)(milliseconds to wait=w1740) -> ()  [unwired: 1 out]
              }
              frame #4 {
                n892 = VISA Write(VISA resource name=w1745, write buffer=w1743, error in (no error)=w1744) -> (VISA resource name out=w1747:refnum<visa-resource-name>, error out=w1746:errorcluster)  [unwired: 1 out]
              }
              frame #5 {
                n893 = Wait (ms)(milliseconds to wait=w1748) -> ()  [unwired: 1 out]
              }
              frame #6 {
                n894 = Concatenate Strings("enter main ", "\r") -> (w1755:string)
                n895 = VISA Write(VISA resource name=w1754, write buffer=w1755, error in (no error)=w1753) -> (VISA resource name out=w1752:refnum<visa-resource-name>, error out=w1751:errorcluster)  [unwired: 1 out]
                n896 = VISA Close(VISA resource name=w1752, error in (no error)=w1751) -> ()  [unwired: 1 out]
              }
            }
            n897 = Concatenate Strings("set units 4", "\r") -> (w1714:string)
            n898 = Number To Decimal String(number="Normal \nVolume (ul) 2") -> (decimal integer string=w1701:string)  [unwired: 1 in]
            n899 = Concatenate Strings("set volume", w1701, "\r") -> (w1711:string)
          }
        }
        n900 = node-c288() -> ()  [unwired: 1 in, 1 out]
      }
      n901 = node-c288(w1087) -> ()  [unwired: 1 out]
    }
    frame Enabled {
    }
  }
  n902 = node-c288() -> (w85:T12)  [unwired: 4 in]
  n903 = call <vilib>:"Simple Error Handler.vi"("error in (no error)"=w105) -> ()  [unwired: 4 in, 5 out]
  n904 = timed-loop {
    timing: w85 -> [_]
    timing-out: [_] -> w84
    stop <- w1764 stop-if-true
    n905 = node-c288() -> ()  [unwired: 1 in, 1 out]
    n906 = event shown="[1] \"Stop\": Value Change" {
      selector: _ -> [_ _]
      dyn-events: _ -> [_ _]
      timeout: _ -> [_ _]
      tunnel: [_ "Stop"] -> w1764
      event Timeout {
        n907 = event-data() -> ()  [unwired: 1 in, 2 out]
      }
      event "Stop": Value Change {
        n908 = event-data() -> ()  [unwired: 1 in, 4 out]
      }
    }
    n909 = node-c288() -> ()  [unwired: 1 in, 1 out]
  }
  n910 = case shown="True" w74 {
    tunnel: w79 -> [_ w1770]
    tunnel: w78 -> [_ w1769]
    tunnel: w77 -> [_ w1768]
    frame False {
    }
    frame True {
      w1772 = T15 3 items=["no dialog", "OK message", "continue or stop message", "OK message + warnings", "continue/stop + warnings"] ("type of dialog (OK msg:1)")
      w1771 = T15 3 items=["no dialog", "OK message", "continue or stop message", "OK message + warnings", "continue/stop + warnings"] ("type of dialog (OK msg:1)")
      n911 = call <vilib>:"DAQmx Clear Task.vi"("task in"=w1770, "error in"=w1768) -> ("error out"=w1773:errorcluster)  [unwired: 13 in]
      n912 = call <vilib>:"DAQmx Clear Task.vi"("task in"=w1769) -> ("error out"=w1774:errorcluster)  [unwired: 14 in]
      n913 = call <vilib>:"Simple Error Handler.vi"("type of dialog (OK msg:1)"=w1772, "error in (no error)"=w1773) -> ()  [unwired: 3 in, 5 out]
      n914 = call <vilib>:"Simple Error Handler.vi"("type of dialog (OK msg:1)"=w1771, "error in (no error)"=w1774) -> ()  [unwired: 3 in, 5 out]
    }
  }
  n915 = case shown="\"Force Feedback\", Default" "?" {
    frame "Force Feedback", Default {
    }
    frame "Raster scan" {
    }
  }
  n916 = node-c288(w84) -> ()  [unwired: 1 out]
  n917 = local write "Tether"(FALSE ("Tether")) -> ()
  n918 = node-c288(i64 50 ("Period"), 2 ("Processor")) -> (w88:T12)  [unwired: 2 in]
  n919 = local read "Path"() -> (w82:path)
  n920 = timed-loop {
    timing: w88 -> [_]
    timing-out: [_] -> w87
    tunnel: w82 -> [w1776]
    stop <- w1775 stop-if-true
    n921 = node-c288() -> ()  [unwired: 1 in, 1 out]
    n922 = event shown="[5] \"Raster scan\": Value Change" {
      selector: _ -> [_ _ _ _ _ _ _ _ _]
      dyn-events: _ -> [_ _ _ _ _ _ _ _ _]
      timeout: _ -> [_ _ _ _ _ _ _ _ _]
      tunnel: w1776 -> [_ w1780 _ _ _ _ _ _ _]
      tunnel: [_ _ w1800 _ _ _ _ _ _] -> w1775
      event Timeout {
        n923 = event-data() -> ()  [unwired: 1 in, 2 out]
      }
      event "Read Cal": Value Change {
        n924 = event-data() -> ()  [unwired: 1 in, 6 out]
        n925 = Path To String(path=w1780) -> (string=w1779:string)
        n926 = Format Date/Time String(time format string (%c)="%y%m%d") -> (date/time string=w1781:string)  [unwired: 2 in]
        n927 = Concatenate Strings(w1779, "\\" ("string"), w1781, "\\" ("string"), "current.cal") -> (w1799:string)
        n928 = String To Path(string=w1799) -> (path=w1798:path)
        n929 = Open/Create/Replace File(file path (use dialog)=w1798, operation (0:open)=T9."open", access (0:read/write)=enum16{"read/write", "read-only", "write-only"}."read-only") -> (refnum out=w1794:refnum<file>, error out=w1795:errorcluster)  [unwired: 3 in, 1 out]
        n930 = Deny Access(4:w1795, 7:w1794) -> (0:w1793:errorcluster, 3:w1792:refnum<file>)  [unwired: 1 in]
        n931 = Read from Binary File(5:0.0, 8:w1793, 9:T10."big-endian, network order" ("byte order (0:big-endian, network order)"), 10:12 ("count"), 11:w1792) -> (0:w1788:errorcluster, 2:w1786:dbl[], 3:w1789:refnum<file>)  [unwired: 1 in, 1 out]
        n932 = Array To Cluster(array=w1786) -> (cluster=→"Cal values":T17)
        n933 = Close File(refnum=w1789, error in=w1788) -> ()  [unwired: 2 out]
        n934 = local write "Read Cal"(FALSE ("Read Cal")) -> ()
      }
      event "Stop": Value Change {
        n935 = event-data() -> ("NewVal"=w1800:bool)  [unwired: 1 in, 5 out]
      }
      event "Trap position": Value Change {
        # "Need to rotate so X and Y don't get mixed up."
        n936 = event-data() -> ()  [unwired: 1 in, 6 out]
        n937 = local read "Mirror task"() -> (w1801:refnum<k21>)
        n938 = Cluster To Array(cluster="Trap position") -> (array=w1804:dbl[])
        n939 = Rotate 1D Array(1:w1804, 2:1 ("n")) -> (0:w1802:dbl[])
        n940 = call-poly <vilib>:"DAQmx Write.vi"("task/channels in"=w1801, "data"=w1802) -> ("task out"=w1807:refnum<k21>, "error out"=w1806:errorcluster)  [unwired: 11 in, 1 out]
        n941 = call <vilib>:"DAQmx Stop Task.vi"("task/channels in"=w1807, "error in"=w1806) -> ("error out"=w1805:errorcluster)  [unwired: 12 in, 1 out]
        n942 = call <vilib>:"Simple Error Handler.vi"("error in (no error)"=w1805) -> ()  [unwired: 4 in, 5 out]
      }
      event "Trap delta": Value Change {
        n943 = event-data() -> ()  [unwired: 1 in, 6 out]
        n944 = local read "Pulling direction"() -> (w1810:bool)
        n945 = local read "Fixed Y"() -> (w1814:dbl)
        n946 = local read "Fixed X"() -> (w1813:dbl)
        n947 = Select(t=w1814, s=w1810, f=w1813) -> (s? t:f=w1812:dbl)
        n948 = Add(x="Trap delta", y=w1812) -> (x+y=w1809:dbl)
        n949 = case shown="True" w1810 {
          tunnel: w1809 -> [w1815 w1816]
          frame False {
            n950 = property on="X" class="DigNum (strict)"("Val(Sgnl)"=w1815) -> ()  [unwired: 2 in, 2 out]
          }
          frame True {
            n951 = property on="Y" class="DigNum (strict)"("Val(Sgnl)"=w1816) -> ()  [unwired: 2 in, 2 out]
          }
        }
      }
      event "Raster scan": Value Change {
        n952 = event-data() -> ()  [unwired: 1 in, 6 out]
        n953 = case shown="True" "Raster scan" {
          frame False {
          }
          frame True {
            w1849 = T15 1 items=["no dialog", "OK message", "continue or stop message", "OK message + warnings", "continue/stop + warnings"] ("type of dialog (OK msg:1)")
            w1833 = 0.0 ("minimum value")
            w1832 = 10.0 ("maximum value")
            # "Grab offset in pulling\ndirection and add to \ndelta values"
            # "Send offset in direction\nof not-pulling to DAQ"
            n954 = local read "Min delta"() -> (w1838:dbl)
            n955 = local read "Max delta"() -> (w1835:dbl)
            n956 = call-poly <vilib>:"DAQmx Create Virtual Channel.vi"("maximum value"=w1832, "minimum value"=w1833, "physical channels"=tag "Dev1/ao0") -> ("task out"=w1854:refnum<k21>, "error out"=w1853:errorcluster)  [unwired: 11 in]
            n957 = local read "Fixed Y"() -> (w1842:dbl)
            n958 = local read "Fixed X"() -> (w1843:dbl)
            n959 = local read "Conv Y (nm/V)"() -> (w1828:dbl)
            n960 = local read "Conv X (nm/V)"() -> (w1830:dbl)
            n961 = local read "Speed (ms)"() -> (w1820:i32)
            n962 = Subtract(x=w1835, y=w1838) -> (x-y=w1826:dbl)
            n963 = Divide(x=w1820, y=2) -> (x/y=w1818:dbl)
            n964 = Select(t=w1843, s="Pulling direction", f=w1842) -> (s? t:f=w1845:dbl)
            n965 = Select(t=w1842, s="Pulling direction", f=w1843) -> (s? t:f=w1839:dbl)
            n966 = Select(t=w1828, s="Pulling direction", f=w1830) -> (s? t:f=w1827:dbl)
            n967 = Divide(x=w1826, y=w1818) -> (x/y=w1825:dbl)
            n968 = call-poly <vilib>:"DAQmx Create Virtual Channel.vi"("task in"=w1854, "maximum value"=w1832, "minimum value"=w1833, "physical channels"=tag "Dev1/ao1", "error in"=w1853) -> ("task out"=w1848:refnum<k21>, "error out"=w1847:errorcluster)  [unwired: 9 in]
            n969 = Multiply(x=w1826, y=w1827) -> (x*y=w1823:dbl)
            "Scan Range (nm)" <- w1823
            n970 = Add(x=w1839, y=w1835) -> (x+y=w1841:dbl)
            n971 = Divide(x=w1818, y=1000) -> (x/y=w1822:dbl)
            n972 = Add(x=w1839, y=w1838) -> (x+y=w1840:dbl)
            n973 = Divide(x=w1823, y=w1822) -> (x/y=→"Scan Speed (nm/s)":dbl)
            n974 = node-c288(i64 1 ("Period")) -> (w1858:T12)  [unwired: 3 in]
            n975 = timed-loop {
              tunnel: "Pulling direction" -> [w1878]
              tunnel: w1825 -> [w1874]
              tunnel: w1840 -> [w1877]
              tunnel: w1845 -> [w1866]
              tunnel: w1848 -> [w1876]
              tunnel: w1847 -> [w1875]
              tunnel: w1841 -> [w1873]
              tunnel: [w1870] -> w1852
              tunnel: [w1869] -> w1851
              tunnel: [w1864] -> w1837
              timing: w1858 -> [_]
              timing-out: [_] -> w1857
              tunnel: w1818 -> [w1865]
              tunnel: "Trap delta\nafter" -> [w1861]
              tunnel: [w1861] -> w1844
              i -> [w1868]
              stop <- w1864 stop-if-true
              n976 = node-c288() -> ()  [unwired: 1 in, 1 out]
              n977 = flat-sequence {
                tunnel: [w1887] -> w1872
                tunnel: [w1886] -> w1871
                tunnel: w1878 -> [w1885]
                tunnel: w1874 -> [w1892]
                tunnel: w1877 -> [w1891]
                tunnel: w1866 -> [w1890]
                tunnel: w1876 -> [w1889]
                tunnel: w1875 -> [w1888]
                tunnel: w1865 -> [w1884]
                tunnel: w1874 -> [w1923]
                tunnel: w1873 -> [w1922]
                tunnel: w1872 -> [w1929]
                tunnel: w1871 -> [w1928]
                tunnel: [w1927] -> w1870
                tunnel: [w1926] -> w1869
                tunnel: w1866 -> [w1924]
                frame #0 {
                  n978 = node-c288(i64 1 ("Period")) -> (w1883:T12)  [unwired: 3 in]
                  n979 = timed-loop {
                    tunnel: w1892 -> [w1912]
                    tunnel: w1891 -> [w1910]
                    tunnel: w1890 -> [w1895]
                    tunnel: w1889 -> [w1909]
                    tunnel: w1888 -> [w1908]
                    tunnel: [w1902] -> w1887
                    tunnel: [w1903] -> w1886
                    tunnel: w1885 -> [w1906]
                    tunnel: w1884 -> [w1904]
                    timing: w1883 -> [_]
                    timing-out: [_] -> w1882
                    i -> [w1900]
                    stop <- w1905 stop-if-true
                    n980 = node-c288() -> ()  [unwired: 1 in, 1 out]
                    n981 = Multiply(x=w1912, y=w1900) -> (x*y=w1911:dbl)
                    n982 = Add(x=w1910, y=w1911) -> (x+y=w1896:dbl)
                    n983 = local read "Stop saving"() -> (w1893:bool)
                    n984 = local read "Stop raster"() -> (w1894:bool)
                    n985 = Build Array(w1895, w1896) -> (w1897:dbl[])
                    n986 = Build Array(w1896, w1895) -> (w1899:dbl[])
                    n987 = Greater Or Equal?(x=w1900, y=w1904) -> (x >= y?=w1901:bool)
                    n988 = Select(t=w1897, s=w1906, f=w1899) -> (s? t:f=w1898:dbl[])
                    n989 = Compound Arithmetic op=OR(w1901, w1894, w1893) -> (w1905:bool)
                    n990 = call-poly <vilib>:"DAQmx Write.vi"("task/channels in"=w1909, "auto start"=TRUE, "data"=w1898, "error in"=w1908) -> ("task out"=w1902:refnum<k21>, "error out"=w1903:errorcluster)  [unwired: 9 in, 1 out]
                    n991 = node-c288() -> ()  [unwired: 1 in, 1 out]
                  }
                  n992 = node-c288(w1882) -> ()  [unwired: 1 out]
                }
                frame #1 {
                  n993 = local read "Pulling direction"() -> (w1925:bool)
                  n994 = node-c288(i64 1 ("Period")) -> (w1921:T12)  [unwired: 3 in]
                  n995 = timed-loop {
                    tunnel: w1923 -> [w1940]
                    tunnel: w1922 -> [w1943]
                    tunnel: w1924 -> [w1934]
                    tunnel: w1929 -> [w1952]
                    tunnel: w1928 -> [w1944]
                    tunnel: [w1936] -> w1927
                    tunnel: [w1946] -> w1926
                    tunnel: w1925 -> [w1948]
                    timing: w1921 -> [_]
                    timing-out: [_] -> w1920
                    i -> [w1941]
                    stop <- w1942 stop-if-true
                    n996 = node-c288() -> ()  [unwired: 1 in, 1 out]
                    n997 = Multiply(x=w1940, y=w1941) -> (x*y=w1939:dbl)
                    n998 = Subtract(x=w1943, y=w1939) -> (x-y=w1938:dbl)
                    n999 = Build Array(w1934, w1938) -> (w1947:dbl[])
                    n1000 = local read "Speed (ms)"() -> (w1931:i32)
                    n1001 = Build Array(w1938, w1934) -> (w1937:dbl[])
                    n1002 = Select(t=w1947, s=w1948, f=w1937) -> (s? t:f=w1935:dbl[])
                    n1003 = Divide(x=w1931, y=2) -> (x/y=w1930:dbl)
                    n1004 = local read "Stop raster"() -> (w1950:bool)
                    n1005 = local read "Stop saving"() -> (w1933:bool)
                    n1006 = Decrement(x=w1930) -> (x-1=w1945:dbl)
                    n1007 = call-poly <vilib>:"DAQmx Write.vi"("task/channels in"=w1952, "auto start"=TRUE, "data"=w1935, "error in"=w1944) -> ("task out"=w1936:refnum<k21>, "error out"=w1946:errorcluster)  [unwired: 9 in, 1 out]
                    n1008 = Greater Or Equal?(x=w1941, y=w1945) -> (x >= y?=w1951:bool)
                    n1009 = node-c288() -> ()  [unwired: 1 in, 1 out]
                    n1010 = Compound Arithmetic op=OR(w1951, w1950, w1933) -> (w1942:bool)
                  }
                  n1011 = node-c288(w1920) -> ()  [unwired: 1 out]
                }
              }
              n1012 = local read "# scans"() -> (w1860:i32)
              n1013 = local read "Stop saving"() -> (w1859:bool)
              n1014 = Decrement(x=w1860) -> (x-1=w1862:i32)
              n1015 = Greater Or Equal?(x=w1868, y=w1862) -> (x >= y?=w1867:bool)
              n1016 = Compound Arithmetic op=OR(w1867, "Stop raster", w1859) -> (w1864:bool)
              n1017 = node-c288() -> ()  [unwired: 1 in, 1 out]
            }
            n1018 = node-c288(w1857) -> ()  [unwired: 1 out]
            n1019 = call <vilib>:"DAQmx Clear Task.vi"("task in"=w1852, "error in"=w1851) -> ("error out"=w1850:errorcluster)  [unwired: 13 in]
            n1020 = Not(x=w1837) -> (.not. x?=w1846:bool)
            n1021 = Not(x=w1837) -> (.not. x?=w1836:bool)
            n1022 = property on="Trap delta" class="DigNum (strict)"("Val(Sgnl)"=w1844) -> ()  [unwired: 2 in, 2 out]
            n1023 = call <vilib>:"Simple Error Handler.vi"("type of dialog (OK msg:1)"=w1849, "error in (no error)"=w1850) -> ()  [unwired: 3 in, 5 out]
            n1024 = local write "Stop raster"(w1846) -> ()
            n1025 = property on="Stop saving" class="Bool (strict)"("Val(Sgnl)"=w1837) -> ()  [unwired: 2 in, 2 out]
            n1026 = local write "Raster scanning..."(w1836) -> ()
          }
        }
      }
      event "Fish": Value Change {
        n1027 = event-data() -> ()  [unwired: 1 in, 6 out]
        n1028 = local read "Fish"() -> (w1963:bool)
        n1029 = case shown="True" w1963 {
          frame False {
          }
          frame True {
            w1972 = 0.0 ("minimum value")
            w1973 = 10.0 ("maximum value")
            # "Grab offset in pulling\ndirection and add to \ndelta values"
            n1030 = call-poly <vilib>:"DAQmx Create Virtual Channel.vi"("maximum value"=w1973, "minimum value"=w1972, "physical channels"=tag "Dev1/ao0") -> ("task out"=w1977:refnum<k21>, "error out"=w1976:errorcluster)  [unwired: 11 in]
            n1031 = call-poly <vilib>:"DAQmx Create Virtual Channel.vi"("task in"=w1977, "maximum value"=w1973, "minimum value"=w1972, "physical channels"=tag "Dev1/ao1", "error in"=w1976) -> ("task out"=w1971:refnum<k21>, "error out"=w1970:errorcluster)  [unwired: 9 in]
            n1032 = node-c288(i64 1 ("Period")) -> (w1979:T12)  [unwired: 3 in]
            n1033 = timed-loop {
              timing: w1979 -> [_]
              timing-out: [_] -> w1978
              tunnel: w1971 -> [w2028]
              tunnel: w1970 -> [w2027]
              tunnel: [w2026] -> w1966
              tunnel: [w2025] -> w1965
              tunnel: [w1993] -> w1968
              tunnel: [w2007] -> w1964
              i -> [w2011]
              stop <- w2007 stop-if-true
              # "Send offset in direction\nof not-pulling to DAQ"
              n1034 = node-c288() -> ()  [unwired: 1 in, 1 out]
              n1035 = local read "Pulling direction"() -> (w1995:bool)
              n1036 = local read "Fixed Y"() -> (w1997:dbl)
              n1037 = local read "Fixed X"() -> (w1998:dbl)
              n1038 = Select(t=w1997, s=w1995, f=w1998) -> (s? t:f=w1999:dbl)
              n1039 = Add(x=w1999, y="Max fish\ndelta (V)") -> (x+y=w2001:dbl)
              n1040 = Subtract(x="Max fish\ndelta (V)", y="Min fish\ndelta (V)") -> (x-y=w2003:dbl)
              n1041 = Select(t=w1998, s=w1995, f=w1997) -> (s? t:f=w1996:dbl)
              n1042 = Divide(x=w2003, y="Fish Speed (ms)") -> (x/y=w2004:dbl)
              n1043 = flat-sequence {
                tunnel: w1995 -> [w2047]
                tunnel: w1996 -> [w2046]
                tunnel: w2028 -> [w2045]
                tunnel: w2027 -> [w2044]
                tunnel: w2004 -> [w2043]
                tunnel: w2001 -> [w2042]
                tunnel: "Fish Speed (ms)" -> [w2037]
                tunnel: [w2041] -> w2024
                tunnel: [w2040] -> w2023
                tunnel: [w2039] -> w2022
                tunnel: [w2038] -> w2021
                tunnel: [w2031] -> w2010
                tunnel: [w2030] -> w1994
                tunnel: [w2029] -> w1991
                tunnel: [w2094] -> w2020
                tunnel: w2024 -> [w2094]
                tunnel: [w2093] -> w2019
                tunnel: w2023 -> [w2093]
                tunnel: [w2092] -> w2018
                tunnel: w2022 -> [w2092]
                tunnel: [w2091] -> w2017
                tunnel: w2021 -> [w2091]
                tunnel: w2010 -> [w2090]
                tunnel: [w2090] -> w2009
                tunnel: w1994 -> [w2089]
                tunnel: [w2088] -> w1992
                tunnel: w1991 -> [w2088]
                tunnel: w2020 -> [w2105]
                tunnel: w2019 -> [w2104]
                tunnel: w2018 -> [w2103]
                tunnel: w2017 -> [w2102]
                tunnel: w2006 -> [w2101]
                tunnel: [w2100] -> w2026
                tunnel: [w2099] -> w2025
                tunnel: w2009 -> [w2098]
                tunnel: [w2097] -> w1993
                tunnel: w1992 -> [w2096]
                frame #0 {
                  n1044 = local read "Mean force (pN)"() -> (w2036:dbl)
                  n1045 = local read "Cutoff force (pN)"() -> (w2035:dbl)
                  n1046 = Less Or Equal?(x=w2036, y=w2035) -> (x <= y?=w2033:bool)
                  n1047 = And(x="Fish", y=w2033) -> (x .and. y?=w2034:bool)
                  n1048 = case shown="True" w2034 {
                    selector: w2034 -> [w2049 _]
                    tunnel: w2047 -> [w2052 w2068]
                    tunnel: w2046 -> [_ w2067]
                    tunnel: w2045 -> [w2054 w2066]
                    tunnel: w2044 -> [w2053 w2065]
                    tunnel: w2043 -> [w2051 w2064]
                    tunnel: w2042 -> [w2050 w2063]
                    tunnel: [w2054 w2062] -> w2041
                    tunnel: [w2053 w2061] -> w2040
                    tunnel: [w2052 w2060] -> w2039
                    tunnel: [w2050 w2059] -> w2029
                    tunnel: [w2051 w2058] -> w2038
                    tunnel: w2037 -> [_ w2057]
                    tunnel: [w2049 w2056] -> w2031
                    tunnel: [FALSE w2055] -> w2030
                    frame False {
                    }
                    frame True {
                      n1049 = while {
                        tunnel: w2068 -> [w2077]
                        tunnel: w2067 -> [w2076]
                        tunnel: w2066 -> [w2084]
                        tunnel: w2065 -> [w2083]
                        tunnel: w2064 -> [w2075]
                        tunnel: w2063 -> [w2081]
                        tunnel: [w2079] -> w2062
                        tunnel: [w2078] -> w2061
                        tunnel: [w2077] -> w2060
                        tunnel: [w2076] -> w2059
                        tunnel: [w2075] -> w2058
                        tunnel: w2057 -> [w2074]
                        tunnel: [w2069] -> w2056
                        tunnel: [w2069] -> w2055
                        i -> [w2073]
                        stop <- w2070 stop-if-true
                        n1050 = Multiply(x=w2075, y=w2073) -> (x*y=w2082:dbl)
                        n1051 = Subtract(x=w2081, y=w2082) -> (x-y=w2080:dbl)
                        n1052 = Build Array(w2076, w2080) -> (w2087:dbl[])
                        n1053 = Build Array(w2080, w2076) -> (w2086:dbl[])
                        n1054 = Greater Or Equal?(x=w2073, y=w2074) -> (x >= y?=w2069:bool)
                        n1055 = Select(t=w2087, s=w2077, f=w2086) -> (s? t:f=w2085:dbl[])
                        n1056 = local read "Fish"() -> (w2071:bool)
                        n1057 = Not(x=w2071) -> (.not. x?=w2072:bool)
                        n1058 = call-poly <vilib>:"DAQmx Write.vi"("task/channels in"=w2084, "data"=w2085, "error in"=w2083) -> ("task out"=w2079:refnum<k21>, "error out"=w2078:errorcluster)  [unwired: 10 in, 1 out]
                        n1059 = Compound Arithmetic op=OR(w2069, w2072) -> (w2070:bool)
                      }
                    }
                  }
                }
                frame #1 {
                  n1060 = case shown="True" w2089 {
                    frame False {
                    }
                    frame True {
                      n1061 = Wait (ms)(milliseconds to wait="Wait (ms)") -> ()  [unwired: 1 out]
                    }
                  }
                }
                frame #2 {
                  n1062 = case shown="True" w2098 {
                    tunnel: w2105 -> [w2108 w2117]
                    tunnel: w2104 -> [w2107 w2116]
                    tunnel: w2103 -> [_ w2115]
                    tunnel: w2102 -> [_ w2114]
                    tunnel: w2101 -> [_ w2113]
                    tunnel: [w2108 w2112] -> w2100
                    tunnel: [w2107 w2111] -> w2099
                    tunnel: [FALSE w2110] -> w2097
                    tunnel: w2096 -> [_ w2109]
                    frame False {
                    }
                    frame True {
                      n1063 = while {
                        tunnel: w2117 -> [w2145]
                        tunnel: w2116 -> [w2144]
                        tunnel: w2115 -> [w2127]
                        tunnel: w2114 -> [w2142]
                        tunnel: w2113 -> [w2141]
                        tunnel: [w2137] -> w2112
                        tunnel: [w2136] -> w2111
                        tunnel: [w2123] -> w2110
                        tunnel: w2109 -> [w2119]
                        i -> [w2128]
                        stop <- w2133 stop-if-true
                        # "If tether formed,\nimmediately change\nto new delta."
                        n1064 = local read "Fixed Y"() -> (w2118:dbl)
                        n1065 = local read "Fixed X"() -> (w2126:dbl)
                        n1066 = local read "Cutoff force (pN)"() -> (w2129:dbl)
                        n1067 = Multiply(x=w2142, y=w2128) -> (x*y=w2143:dbl)
                        n1068 = local read "Mean force (pN)"() -> (w2130:dbl)
                        n1069 = Add(x=w2141, y=w2143) -> (x+y=w2121:dbl)
                        n1070 = Select(t=w2118, s=w2127, f=w2126) -> (s? t:f=w2125:dbl)
                        n1071 = Greater?(x=w2130, y=w2129) -> (0:w2123:bool)
                        n1072 = Add(x=w2125, y="Delta after tether") -> (x+y=w2122:dbl)
                        n1073 = Select(t=w2122, s=w2123, f=w2121) -> (s? t:f=w2120:dbl)
                        n1074 = local read "Fish Speed (ms)"() -> (w2135:i32)
                        n1075 = Build Array(w2119, w2120) -> (w2140:dbl[])
                        n1076 = Build Array(w2120, w2119) -> (w2139:dbl[])
                        n1077 = Select(t=w2140, s=w2127, f=w2139) -> (s? t:f=w2138:dbl[])
                        n1078 = local read "Fish"() -> (w2132:bool)
                        n1079 = Greater Or Equal?(x=w2128, y=w2135) -> (x >= y?=w2134:bool)
                        n1080 = Not(x=w2132) -> (.not. x?=w2131:bool)
                        n1081 = call-poly <vilib>:"DAQmx Write.vi"("task/channels in"=w2145, "data"=w2138, "error in"=w2144) -> ("task out"=w2137:refnum<k21>, "error out"=w2136:errorcluster)  [unwired: 10 in, 1 out]
                        n1082 = Compound Arithmetic op=OR(w2134, w2131, w2123) -> (w2133:bool)
                      }
                    }
                  }
                }
              }
              n1083 = Add(x=w1999, y="Min fish\ndelta (V)") -> (x+y=w2006:dbl)
              n1084 = Decrement(x="# attempts") -> (x-1=w2015:dbl)
              n1085 = Greater Or Equal?(x=w2011, y=w2015) -> (x >= y?=w2014:bool)
              n1086 = local read "Mean force (pN)"() -> (w2013:dbl)
              n1087 = Greater?(x=w2013, y="Cutoff force (pN)") -> (0:w2008:bool)
              n1088 = Compound Arithmetic op=OR(w1993, w2008, w2014) -> (w2007:bool)
              n1089 = case shown="True" w1993 {
                frame False {
                }
                frame True {
                  n1090 = call <vilib>:"Beep.vi"() -> ()  [unwired: 12 in]
                }
              }
              n1091 = node-c288() -> ()  [unwired: 1 in, 1 out]
              "Tether" <- w1993
              "Attempt #" <- w2011
            }
            n1092 = node-c288(w1978) -> ()  [unwired: 1 out]
            n1093 = flat-sequence {
              tunnel: w1968 -> [w1986]
              tunnel: [w1986] -> w1967
              tunnel: w1966 -> [w1983]
              tunnel: w1965 -> [w1982]
              tunnel: w1964 -> [w1981]
              tunnel: w1967 -> [w1988]
              frame #0 {
                w1985 = T15 1 items=["no dialog", "OK message", "continue or stop message", "OK message + warnings", "continue/stop + warnings"] ("type of dialog (OK msg:1)")
                n1094 = call <vilib>:"DAQmx Clear Task.vi"("task in"=w1983, "error in"=w1982) -> ("error out"=w1984:errorcluster)  [unwired: 13 in]
                n1095 = Not(x=w1981) -> (.not. x?=w1980:bool)
                n1096 = local write "Fish"(w1980) -> ()
                n1097 = call <vilib>:"Simple Error Handler.vi"("type of dialog (OK msg:1)"=w1985, "error in (no error)"=w1984) -> ()  [unwired: 3 in, 5 out]
              }
              frame #1 {
                n1098 = And(x=w1988, y="Raster after\n tether?") -> (x .and. y?=w1989:bool)
                n1099 = case shown="True" w1989 {
                  selector: w1989 -> [_ w1990]
                  frame False {
                  }
                  frame True {
                    n1100 = property on="Raster scan" class="Bool (strict)"("Val(Sgnl)"=w1990) -> ()  [unwired: 2 in, 2 out]
                  }
                }
              }
            }
          }
        }
      }
      event "Load param": Value Change {
        n1101 = event-data() -> ()  [unwired: 1 in, 6 out]
        n1102 = property on="Scan Parameters" class="Arr (strict)"() -> ("Index Values"=w2161:u32[])  [unwired: 2 in, 2 out]
        n1103 = Index Array(array=w2161, index=0) -> (element=w2158:u32)
        n1104 = Index Array(array="Scan Parameters", index=w2158) -> (element=w2157:T18)
        n1105 = Unbundle(w2157) -> ("Max delta 2"=w2156:dbl, "Min delta 2"=w2152:dbl, "Speed (ms) 2"=w2155:i32, "# scans 2"=w2154:i32)  [unwired: 1 out]
        n1106 = property on="Max delta" class="DigNum (strict)"("Val(Sgnl)"=w2156) -> ()  [unwired: 2 in, 2 out]
        n1107 = local write "Load param"(FALSE ("Load param")) -> ()
        n1108 = property on="# scans" class="DigNum (strict)"("Val(Sgnl)"=w2154) -> ()  [unwired: 2 in, 2 out]
        n1109 = property on="Speed (ms)" class="DigNum (strict)"("Val(Sgnl)"=w2155) -> ()  [unwired: 2 in, 2 out]
        n1110 = property on="Min delta" class="DigNum (strict)"("Val(Sgnl)"=w2152) -> ()  [unwired: 2 in, 2 out]
      }
      event "Averaging Number": Value Change {
        n1111 = event-data() -> ()  [unwired: 1 in, 6 out]
        n1112 = local read "# Samples/channel (in)"() -> (w2165:i32)
        n1113 = local read "Averaging Number"() -> (w2163:i32)
        n1114 = Quotient & Remainder(x=w2165, y=w2163) -> (floor(x/y)=w2164:i32)  [unwired: 1 out]
        n1115 = Multiply(x=w2164, y=w2163) -> (x*y=w2162:i32)
        n1116 = local write "# Samples/channel (in)"(w2162) -> ()
      }
    }
    n1117 = node-c288() -> ()  [unwired: 1 in, 1 out]
  }
  n1118 = local write "Pause Mouse/Mirror Connection"(FALSE ("Pause Mouse/Mirror Connection")) -> ()
  n1119 = local write "Stop"(FALSE ("Stop all")) -> ()
  n1120 = node-c288(w87) -> ()  [unwired: 1 out]
  "CoordinatesMousePressed" <- T4 {"Horizontal"=0, "Vertical"=0} ("Coords when pressed")
  "Deflection" <- T4 {"Horizontal"=0, "Vertical"=0} ("Coords when pressed")
